vi "SubMatrixVg.vi"(0 "Target Voltage, V":dbl=1.0 min=-4.0 max=4.0 step=0.1 format="%.4f", 2 "Sweep rate, V/min":dbl=0.1 min=0.0 max=1.0 step=0.01 format="%.4f", 3 "Custom Folder":string, 4 "Time Stamp":timestamp, 5 "optional Bias (V)":dbl=1e-08) -> ()   [LabVIEW 2015]
uses:
  <vilib>/Utility/file.llb/Write To Spreadsheet File (DBL).vi
panel:
  out "Comments":string[](array[string])
  out "ArrayBoolian":bool[][](array[boolean])
  out "Numeric 4":i32
  in  "Commutator":bool
  in  "Commute SorceMeter":enum32{"Radio Selection 1", "Radio Selection 2"}(radio)
  out "Numeric 3":i32
  in  "Channel 2 (Vnano3b)":bool
  in  "Channel 1 (Vnano3)":bool
  out "Numeric":i32
  in  "Capacitance (C) and Loss (L)":bool
  in  "Magnetic Field (B)":bool=TRUE
  in  "Current (Ik3)":bool
  in  "Voltage (Vk3)":bool
  in  "Current (Ik2)":bool
  in  "Voltage (Vk2)":bool
  in  "Channel 2 (Vnano2b)":bool
  in  "Channel 1 (Vnano2)":bool
  in  "Thermometer 1 (T1)":bool=TRUE
  in  "Channel 2 (Vnano1b)":bool
  in  "Channel 1 (Vnano1)":bool
  in  "Current (Ik1)":bool=TRUE
  in  "Voltage (Vk1)":bool
  out "Numeric Current":dbl
  out "Main Keithly2614B address":string="12"
  out "Delib Time delay":i32
  in  "points at each Vg":i32=1
  out "XY Graph":cluster{dbl[], dbl[]}(graph)={[1.0, 0.8, 0.6000000000000001, 0.4000000000000001, 0.20000000000000007, 5.551115123125783e-17, -0.19999999999999996, -0.39999999999999997, -0.6, -0.8, -1.0], [0.03352775, 0.056811, 0.03911575, 0.04330675, -0.02468015, 0.011641600000000002, 0.10151450000000001, 0.12386675000000001, 0.08288825000000001, -0.00186266, -0.038650000000000004]}
  in  "Time btw \npoints, sec":dbl=1.0 format="%.2f"
  out "Array 2":dbl[][](array[numeric])
  out "array for data":dbl[](array[numeric])
  out "Array":string[](array[string])
  in  "Addr 1 lock-in oop":bool=TRUE
  in  "Ring":u16(ring) caption="Y-axis:" items=["Vg", "I", "R1", "R1oop", "Ik1", "T1", "B"]
  out "String":string
  out "Data file:":path
  in  "Set compliance limit, mkA":dbl=0.05 min=0.0 max=1.0 step=0.01 format="%.3f"
  in  "error in (no error)":errorcluster
  in  "Ring 3":u16(ring)=1 items=["1 kOhm", "10 kOhm", "100 kOhm", "1 Mohm", "10 mOhm"]
  in  "Ring 2":u16(ring)=4 items=["1 kOhm", "10 kOhm", "100 kOhm", "1 Mohm", "10 mOhm"]
  in  "Fixed Current mkA":dbl=0.5
  in  "Current is:":T1(radio)
  in  "Ressitance measurements?":bool=TRUE
  in  "Addr 5 lock-in oop":bool
  in  "Addr 4 lock-in oop":bool
  in  "Addr 3 lock-in oop":bool
  in  "Addr 2 lock-in oop":bool
  in  "Addr 5 lock-in":bool
  in  "Addr 4 lock-in":bool
  in  "Addr 3 lock-in":bool
  in  "Addr 2 lock-in":bool
  in  "Addr 1 lock-in":bool=TRUE
  # "Keithley 2400: address 12"
  # "0"
  # "SourceMeters"
  # "Nanovoltmeters"
  # "Temperature"
  # "Main"
  # "Magnetic Field"
  # "(not recommended, too slow)"
  # "Capacitance & Loss"
  # "(not recommended, too slow)"
  # "(not recommended, too slow)"
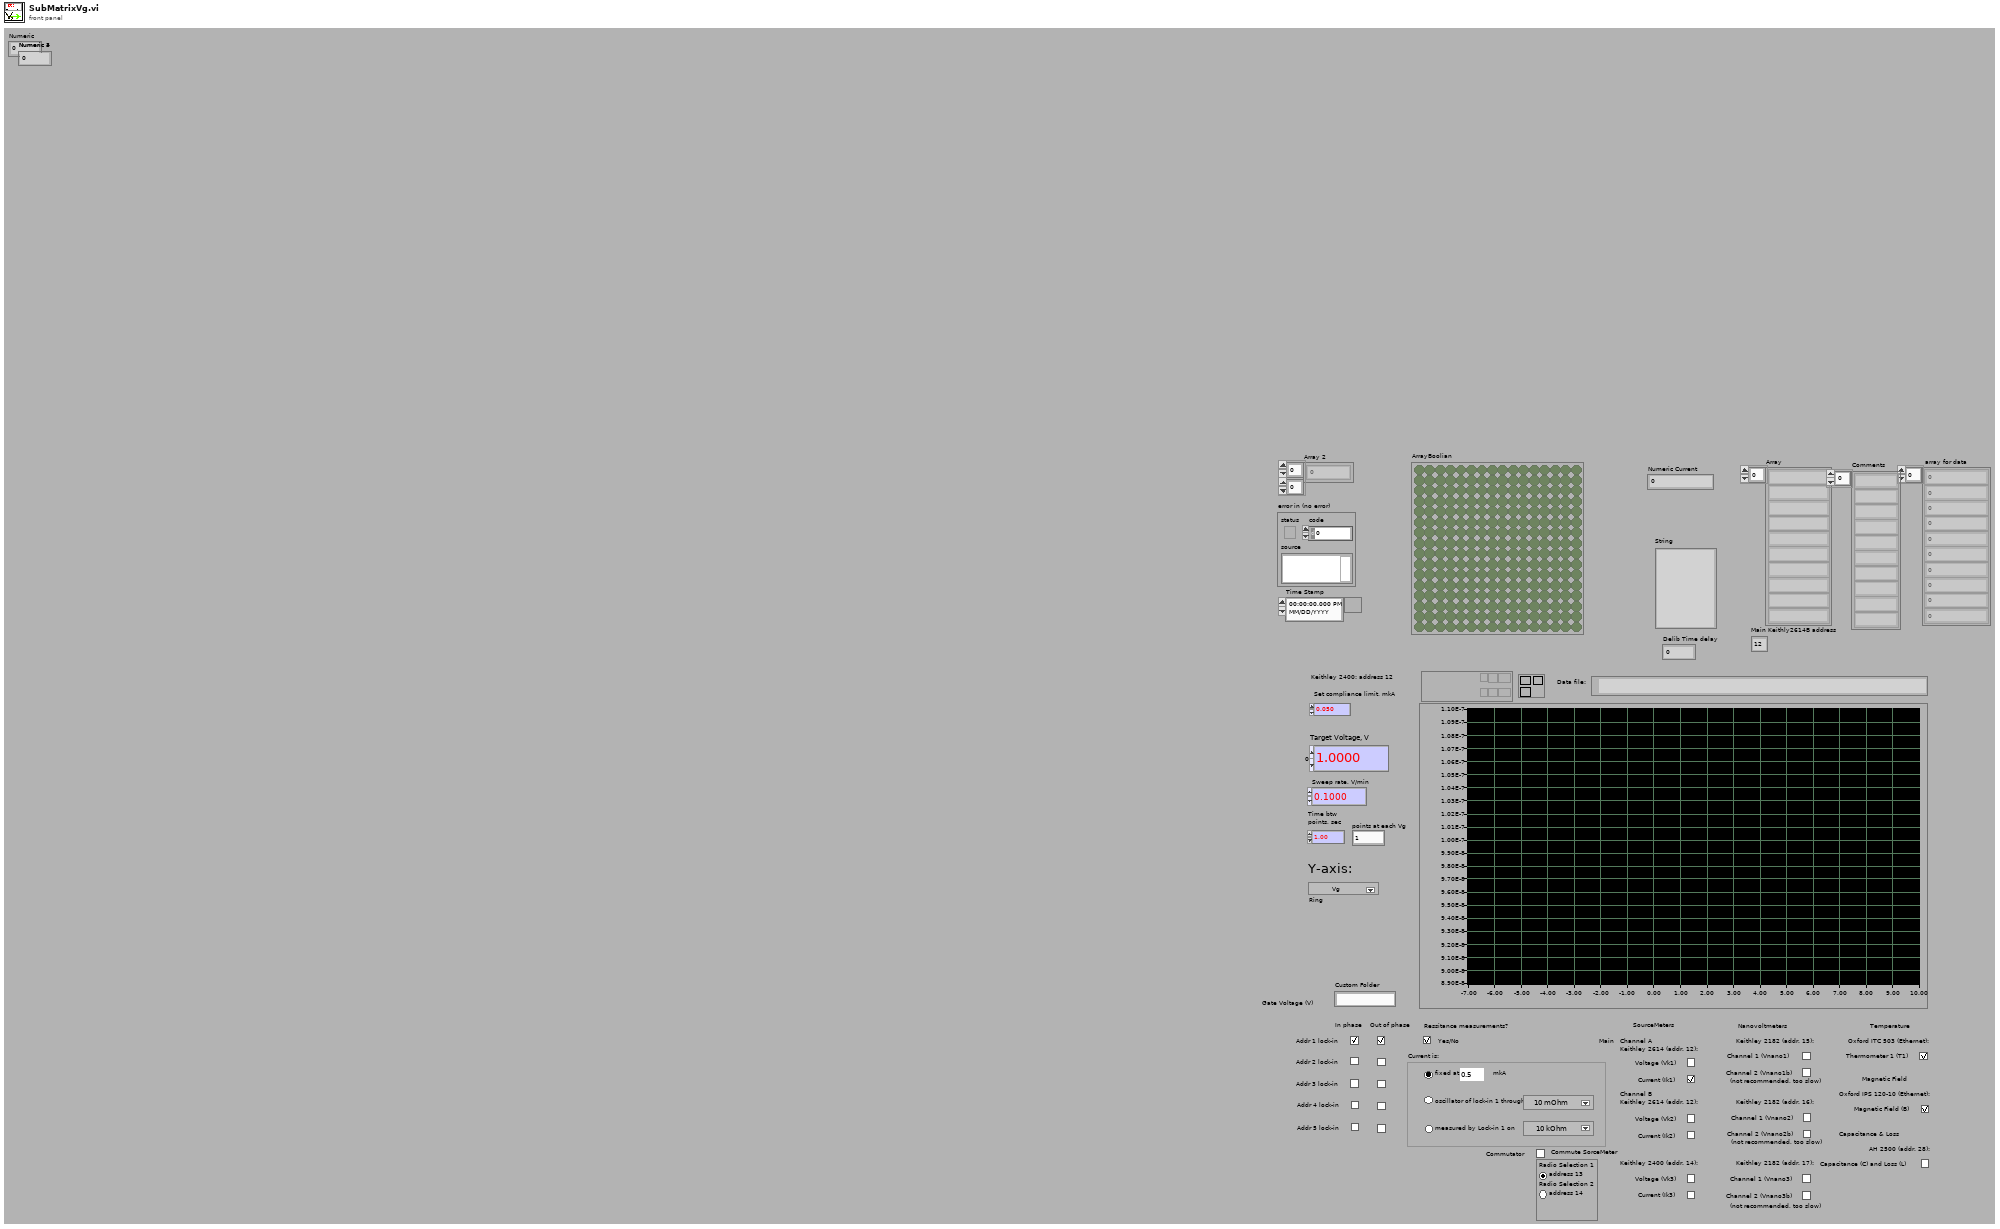
[diagram p1: front panel]
types:
  T1 = enum32{"Radio Selection 1", "Radio Selection 2", "Radio Selection 3"}
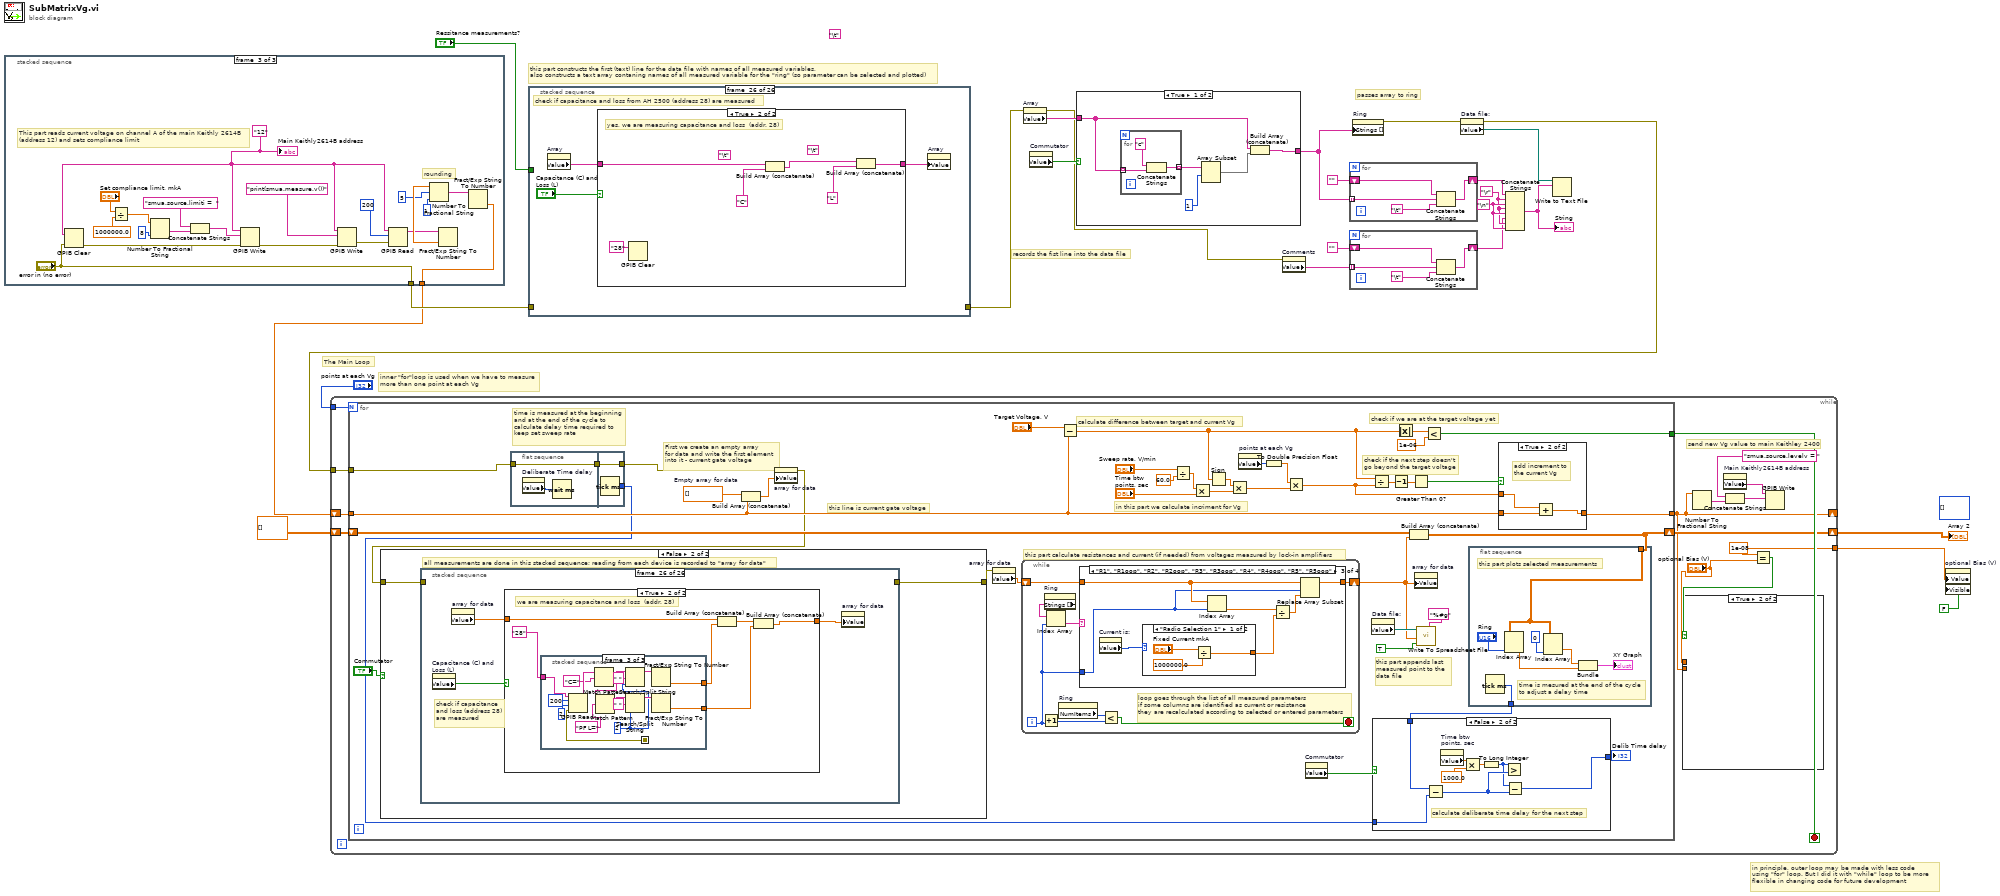
[diagram p0: block diagram]
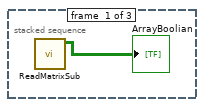
[diagram p3: hidden frame]
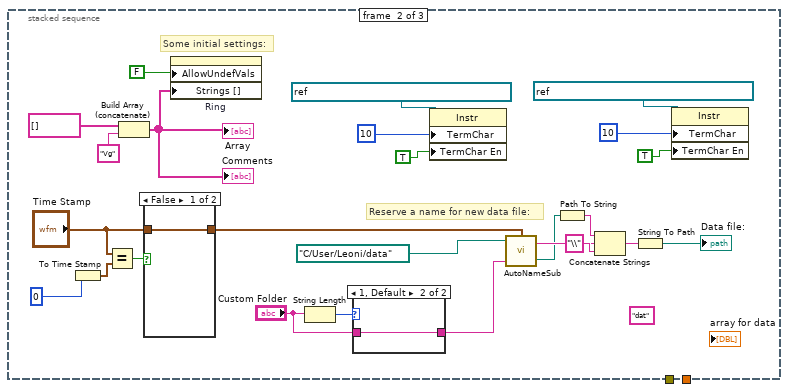
[diagram p4: hidden frame]
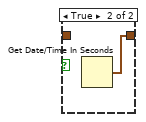
[diagram p5: hidden frame]
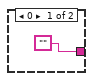
[diagram p6: hidden frame]
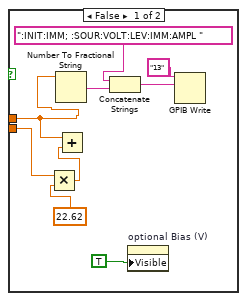
[diagram p7: hidden frame]
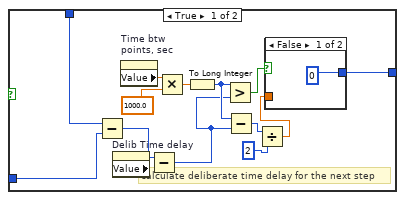
[diagram p8: hidden frame]
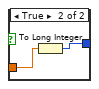
[diagram p9: hidden frame]
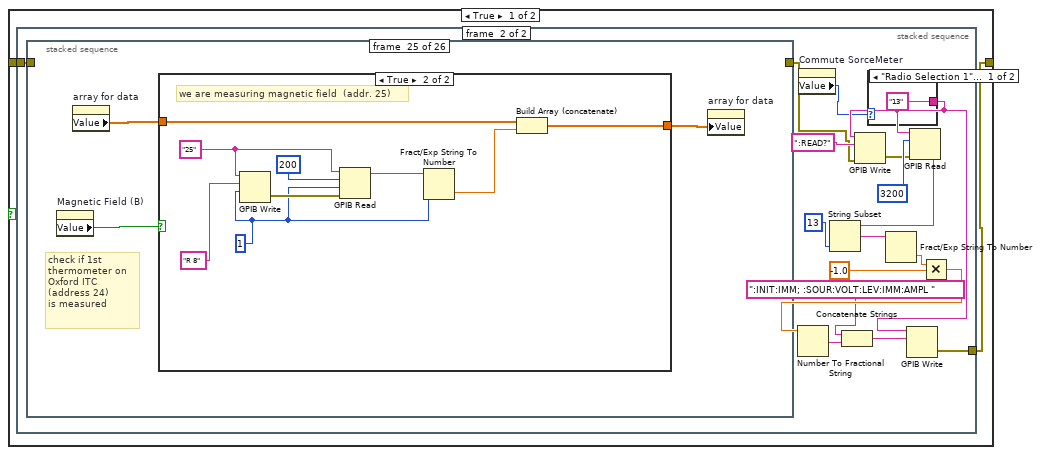
[diagram p10: hidden frame]
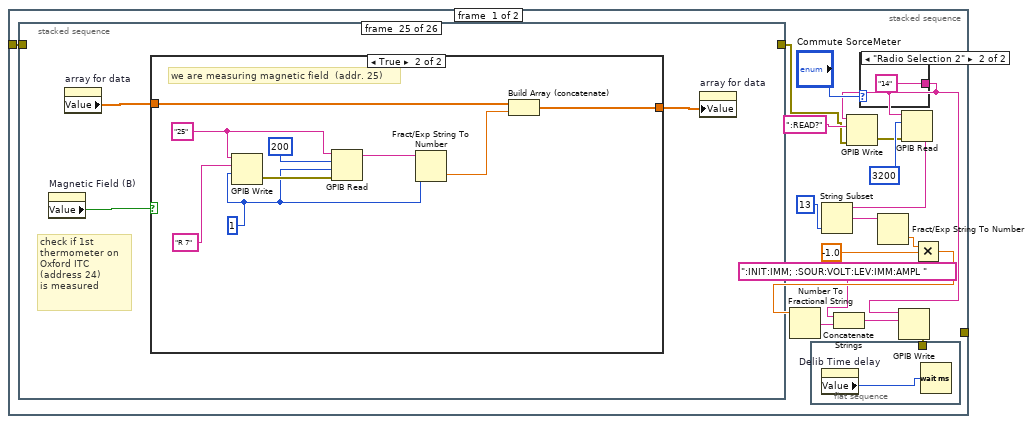
[diagram p11: hidden frame]
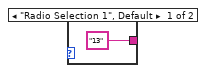
[diagram p12: hidden frame]
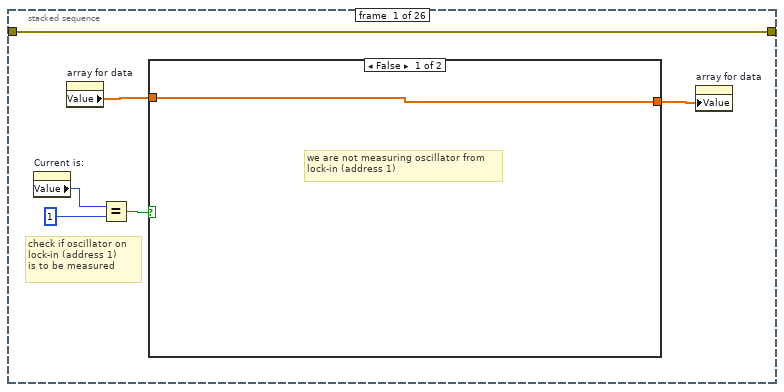
[diagram p13: hidden frame]
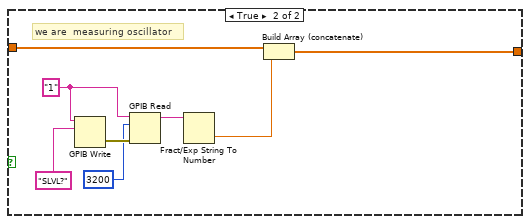
[diagram p14: hidden frame]
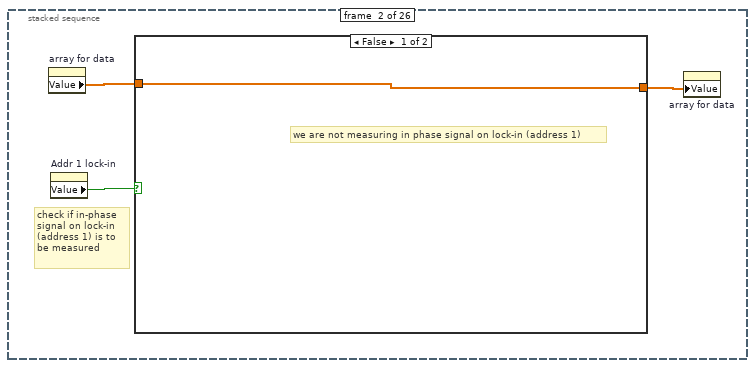
[diagram p15: hidden frame]
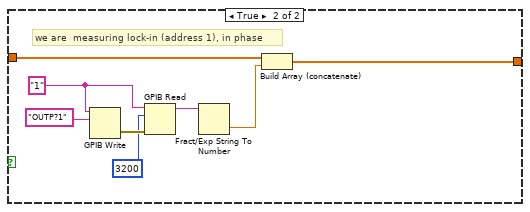
[diagram p16: hidden frame]
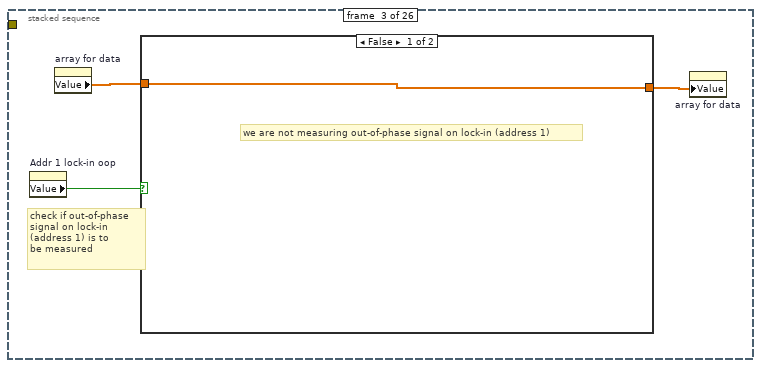
[diagram p17: hidden frame]
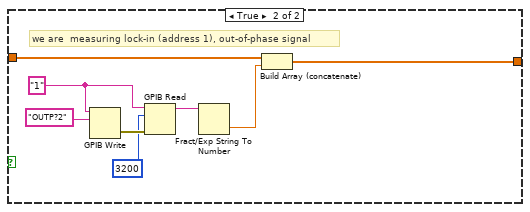
[diagram p18: hidden frame]
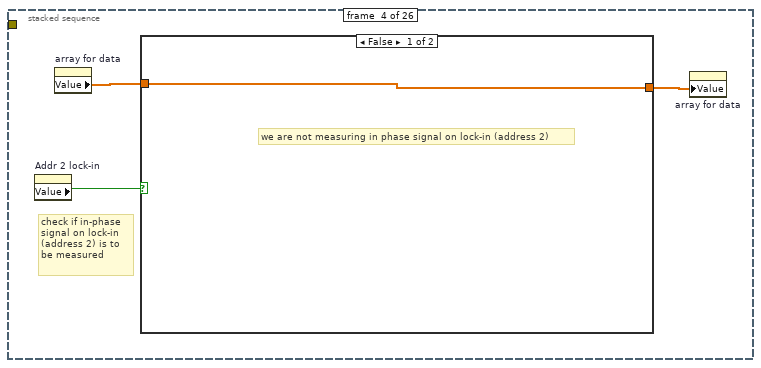
[diagram p19: hidden frame]
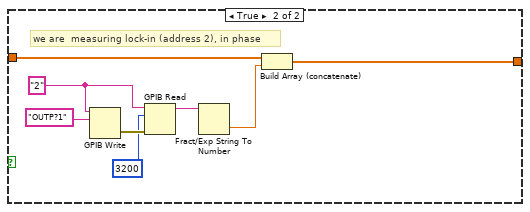
[diagram p20: hidden frame]
diagram:
  (unwired) "\t"
  w3 = "\r"
  w4 = "\n"
  (unwired) i32[][] []
  # "passes array to ring"
  # "in principle, outer loop may be made with less code\nusing \"for\" loop. But I did it with \"while\" loop to be more \nflexible in changing code for future development"
  # "inner \"for\"loop is used when we have to measure\nmore than one point at each Vg"
  # "The Main Loop"
  # "records the fist line into the data file"
  # "this part constructs the first (text) line for the data file with names of all measured variables,\nalso constructs a text array contaning names of all measured variable for the \"ring\" (so parameter can be selected and plotted)"
  n1 = stacked-sequence {
    tunnel: [_ _ "error in (no error)"] -> w24
    tunnel: [_ _ w55] -> w13
    frame #0 {
      n2 = call "ReadMatrixSub.vi"() -> ("Array"=→"ArrayBoolian":bool[][])  [unwired: 9 in, 2 out]
    }
    frame #1 {
      (unwired) "dat"
      # "Some initial settings:"
      # "Reserve a name for new data file:"
      n3 = To Time Stamp(1:0) -> (0:w29:timestamp)
      n4 = Equal?(x="Time Stamp", y=w29) -> (x = y?=w28:bool)
      n5 = Build Array (concatenate)(string[] [], "Vg") -> (w31:string[])
      "Array" <- w31
      "Comments" <- w31
      n6 = case shown="False" w28 {
        tunnel: "Time Stamp" -> [w51 _]
        tunnel: [w51 w52] -> w26
        frame False {
        }
        frame True {
          n7 = Get Date/Time In Seconds() -> (seconds since 1Jan1904=w52:timestamp)
        }
      }
      n8 = property on="Ring" class="Ring (strict)"("AllowUndefVals"=FALSE, "Strings []"=w31) -> ()  [unwired: 2 in, 2 out]
      n9 = String Length(string="Custom Folder") -> (length=w41:i32)
      n10 = case shown="1, Default" w41 {
        tunnel: "Custom Folder" -> [_ w54]
        tunnel: ["" w54] -> w39
        frame 0 {
        }
        frame 1, Default {
        }
      }
      n11 = property class="Instr"(reference=refnum<visa-resource-name> "TCPIP0::192.168.128.3::7020::SOCKET" ("VISA resource name"), "TermChar"=10, "TermChar En"=TRUE) -> ()  [unwired: 1 in, 2 out]
      n12 = call "AutoNameSub.vi"("Time Stamp"=w26, "Custom Folder"=w39, "User Data Folder"=path "C:/User/Leoni/data") -> ("created path"=w49:path, "String"=w50:string)  [unwired: 1 in]
      n13 = Path To String(path=w49) -> (string=w44:string)
      n14 = Concatenate Strings(w44, "\\", w50) -> (w46:string)
      n15 = String To Path(string=w46) -> (path=→"Data file:":path)
      n16 = property class="Instr"(reference=refnum<visa-resource-name> "TCPIP0::192.168.128.2::7020::SOCKET" ("VISA resource name"), "TermChar"=10, "TermChar En"=TRUE) -> ()  [unwired: 1 in, 2 out]
    }
    frame #2 {
      w62 = "12"
      # "rounding"
      # "This part reads current voltage on channel A of the main Keithly 2614B \n(address 12) and sets compliance limit"
      n17 = GPIB Clear(2:"error in (no error)", 3:w62) -> (0:w67:errorcluster)  [unwired: 1 out]
      n18 = Divide(x="Set compliance limit, mkA", y=1000000.0) -> (x/y=w73:dbl)
      n19 = Number To Fractional String(number=w73, precision (6)=i16 8) -> (F-format string=w69:string)  [unwired: 2 in]
      n20 = Concatenate Strings("smua.source.limiti =  " ("data"), w69) -> (w68:string)
      n21 = GPIB Write(0:w62, 1:w68, 3:w67) -> (6:w63:errorcluster)  [unwired: 2 in, 1 out]
      n22 = GPIB Write(0:w62, 1:"print(smua.measure.v())" ("data"), 3:w63) -> (6:w66:errorcluster)  [unwired: 2 in, 1 out]
      n23 = GPIB Read(0:w62, 1:200 ("byte count"), 3:w66) -> (5:w56:string)  [unwired: 2 in, 2 out]
      n24 = Fract/Exp String To Number(string=w56) -> (number=w60:dbl)  [unwired: 3 in, 1 out]
      n25 = Number To Fractional String(number=w60, width (-)=5, precision (6)=1) -> (F-format string=w57:string)  [unwired: 1 in]
      n26 = Fract/Exp String To Number(string=w57) -> (number=w55:dbl)  [unwired: 3 in, 1 out]
      "Main Keithly2614B address" <- w62
    }
  }
  n27 = stacked-sequence {
    tunnel: "Ressitance measurements?" -> [w82 w103 w130 w147 w167 w179 w191 w203 w215 w227 w239 _ _ _ _ _ _ _ _ _ _ _ _ _ _ _]
    tunnel: w24 -> [_ w102 _ _ _ _ _ _ _ _ _ _ _ _ _ _ _ _ _ _ _ _ _ _ _ _]
    tunnel: [_ w102 _ _ _ _ _ _ _ _ _ _ _ _ _ _ _ _ _ _ _ _ _ _ _ _] -> w21
    frame #0 {
      # "check if oscillator of  lock-in (address 1) is to be measured"
      n28 = property on="Array" class="Arr (strict)"() -> ("Value"=w78:string[])  [unwired: 2 in, 2 out]
      n29 = property on="Comments" class="Arr (strict)"() -> ("Value"=w75:string[])  [unwired: 2 in, 2 out]
      n30 = Equal?(x="Current is:", y=1) -> (x = y?=w80:bool)
      n31 = case shown="True" w80 {
        tunnel: w82 -> [_ _]
        tunnel: w78 -> [w84 w95]
        tunnel: [w84 w94] -> w77
        tunnel: [w83 w87] -> w76
        tunnel: w75 -> [w83 w86]
        frame False {
          # "we are not measuring oscillator from\nlock-in (address 1)"
        }
        frame True {
          # "This subVI takes the matrix column # (instrument\nconnection point) as an argument and finds the raw\n# (contact) to which the instrument is connected"
          # "we are  measuring oscillator"
          n32 = property on="ArrayBoolian" class="Arr (strict)"() -> ("Value"=w91:bool[][])  [unwired: 2 in, 2 out]
          n33 = GPIB Clear(3:"1") -> ()  [unwired: 1 in, 2 out]
          n34 = call "FindInstrConnect.vi"("Column #"=1, "ArrayBoolian"=w91) -> ("String"=w92:string)  [unwired: 1 in, 2 out]
          n35 = call "FindInstrConnect.vi"("Column #"=0, "ArrayBoolian"=w91) -> ("String"=w89:string)  [unwired: 1 in, 2 out]
          n36 = Concatenate Strings(w89, "-", w92) -> (w85:string)
          n37 = Build Array (concatenate)(w95, "I") -> (w94:string[])
          n38 = Build Array (concatenate)(w86, w85) -> (w87:string[])
        }
      }
      n39 = property on="Comments" class="Arr (strict)"("Value"=w76) -> ()  [unwired: 2 in, 2 out]
      n40 = property on="Array" class="Arr (strict)"("Value"=w77) -> ()  [unwired: 2 in, 2 out]
    }
    frame #1 {
      # "check if lock-in (address 1) is to be measured"
      n41 = property on="Array" class="Arr (strict)"() -> ("Value"=w101:string[])  [unwired: 2 in, 2 out]
      n42 = property on="Comments" class="Arr (strict)"() -> ("Value"=w99:string[])  [unwired: 2 in, 2 out]
      n43 = case shown="True" "Addr 1 lock-in" {
        tunnel: w103 -> [_ w119]
        tunnel: w101 -> [w106 w117]
        tunnel: [w106 w118] -> w100
        tunnel: w99 -> [w105 w108]
        tunnel: [w105 w109] -> w98
        frame False {
          # "we are not measuring in phase signal from\nlock-in (address 1)"
        }
        frame True {
          # "are we measuring resistance?"
          n44 = case shown="True" w119 {
            tunnel: ["V1" w121] -> w110
            frame False {
              # "no, we are not measuring resistanse;\nall lock-ins are measuring voltage"
            }
            frame True {
              # "are we measuring current as well?"
              n45 = property on="Current is:" class="RadioBtnsControl (strict)"() -> ("Value"=w123:T1)  [unwired: 2 in, 2 out]
              n46 = Equal?(x=w123, y=2) -> (x = y?=w124:bool)
              n47 = case shown="False" w124 {
                tunnel: ["R1" "I"] -> w121
                frame False {
                  # "no, we are not \nmeasuring current\nby lock-in \n(address 1); \nso this lock-in is \nmeasuring resistance"
                }
                frame True {
                  # "yes, we are measuring \ncurrent by lock-in \n(address 1) as \nvoltage drop on \nknown resistance"
                }
              }
            }
          }
          n48 = property on="ArrayBoolian" class="Arr (strict)"() -> ("Value"=w111:bool[][])  [unwired: 2 in, 2 out]
          n49 = call "FindInstrConnect.vi"("Column #"=3, "ArrayBoolian"=w111) -> ("String"=w114:string)  [unwired: 1 in, 2 out]
          n50 = call "FindInstrConnect.vi"("Column #"=2, "ArrayBoolian"=w111) -> ("String"=w112:string)  [unwired: 1 in, 2 out]
          n51 = Concatenate Strings(w112, "-", w114) -> (w107:string)
          n52 = Build Array (concatenate)(w117, w110) -> (w118:string[])
          n53 = Build Array (concatenate)(w108, w107) -> (w109:string[])
        }
      }
      n54 = property on="Array" class="Arr (strict)"("Value"=w100) -> ()  [unwired: 2 in, 2 out]
      n55 = property on="Comments" class="Arr (strict)"("Value"=w98) -> ()  [unwired: 2 in, 2 out]
    }
    frame #2 {
      # "check if out-of-phase signal on  lock-in (address 1) is to be measured"
      n56 = property on="Array" class="Arr (strict)"() -> ("Value"=w129:string[])  [unwired: 2 in, 2 out]
      n57 = case shown="True" "Addr 1 lock-in oop" {
        tunnel: w130 -> [_ w136]
        tunnel: w129 -> [w131 w133]
        tunnel: [w131 w134] -> w128
        frame False {
          # "we are not measuring iout-of-phase signal from\nlock-in (address 1)"
        }
        frame True {
          # "are we measuring resistance?"
          n58 = GPIB Clear(3:"1") -> ()  [unwired: 1 in, 2 out]
          n59 = case shown="False" w136 {
            tunnel: ["V1oop" w138] -> w132
            frame False {
              # "no, we are not measuring resistance;\nall lock-ins are measuring voltage"
            }
            frame True {
              # "are we measuring out-of-phase current as well?"
              n60 = property on="Current is:" class="RadioBtnsControl (strict)"() -> ("Value"=w140:T1)  [unwired: 2 in, 2 out]
              n61 = Equal?(x=w140, y=2) -> (x = y?=w141:bool)
              n62 = case shown="True" w141 {
                tunnel: ["R1oop" "Ioop"] -> w138
                frame False {
                  # "no, we are not \nmeasuring current\nby lock-in \n(address 1); so this \nlock-in is measuring\nout-of-phase resistance"
                }
                frame True {
                  # "yes, we are measuring \nout-of phase current \nby lock-in (address 1) \nas voltage drop on \nknown resistance"
                }
              }
            }
          }
          n63 = Build Array (concatenate)(w133, w132) -> (w134:string[])
        }
      }
      n64 = property on="Array" class="Arr (strict)"("Value"=w128) -> ()  [unwired: 2 in, 2 out]
    }
    frame #3 {
      # "check if in-phase signal on  lock-in (address 2) is to be measured"
      n65 = property on="Array" class="Arr (strict)"() -> ("Value"=w146:string[])  [unwired: 2 in, 2 out]
      n66 = case shown="False" "Addr 2 lock-in" {
        tunnel: w147 -> [_ w161]
        tunnel: w146 -> [w148 w158]
        tunnel: [w148 w159] -> w145
        frame False {
          # "we are not measuring in-phase signal from\nlock-in (address 2)"
        }
        frame True {
          (unwired) "\t"
          # "are we measuring resistance?"
          n67 = GPIB Clear(3:"2") -> ()  [unwired: 1 in, 2 out]
          n68 = case shown="False" w161 {
            tunnel: ["R2 (" "V2 ("] -> w150
            frame True {
              # "we are measuring \nresistance by lock-in \n(address 2)"
            }
            frame False, Default {
              # "no, we are not \nmeasuring resistance;\nall lock-ins are \nmeasuring voltage"
            }
          }
          n69 = property on="ArrayBoolian" class="Arr (strict)"() -> ("Value"=w149:bool[][])  [unwired: 2 in, 2 out]
          n70 = call "FindInstrConnect.vi"("Column #"=5, "ArrayBoolian"=w149) -> ("String"=w154:string)  [unwired: 1 in, 2 out]
          n71 = call "FindInstrConnect.vi"("Column #"=4, "ArrayBoolian"=w149) -> ("String"=w152:string)  [unwired: 1 in, 2 out]
          n72 = Concatenate Strings(w150, w152, "-", w154, ")") -> (w151:string)
          n73 = Build Array (concatenate)(w158, w151) -> (w159:string[])
        }
      }
      n74 = property on="Array" class="Arr (strict)"("Value"=w145) -> ()  [unwired: 2 in, 2 out]
    }
    frame #4 {
      # "check if out-of-phase signal on  lock-in (address 2) is to be measured"
      n75 = property on="Array" class="Arr (strict)"() -> ("Value"=w166:string[])  [unwired: 2 in, 2 out]
      n76 = case shown="True" "Addr 2 lock-in oop" {
        tunnel: w167 -> [_ w173]
        tunnel: w166 -> [w168 w170]
        tunnel: [w168 w171] -> w165
        frame False {
          # "we are not measuring out-of-phase signal from\nlock-in (address 2)"
        }
        frame True {
          (unwired) "\t"
          # "are we measuring resistance?"
          n77 = GPIB Clear(3:"2") -> ()  [unwired: 1 in, 2 out]
          n78 = case shown="True" w173 {
            tunnel: ["R2oop" "V2oop"] -> w169
            frame True {
              # "we are measuring out-of-phase resistance by lock-in (address 2)\n(address 2)"
            }
            frame False, Default {
              # "no, we are not measuring resistance;\nall lock-ins are measuring voltage"
            }
          }
          n79 = Build Array (concatenate)(w170, w169) -> (w171:string[])
        }
      }
      n80 = property on="Array" class="Arr (strict)"("Value"=w165) -> ()  [unwired: 2 in, 2 out]
    }
    frame #5 {
      # "check if in-phase signal on  lock-in (address 3) is to be measured"
      n81 = property on="Array" class="Arr (strict)"() -> ("Value"=w178:string[])  [unwired: 2 in, 2 out]
      n82 = case shown="True" "Addr 3 lock-in" {
        tunnel: w179 -> [_ w185]
        tunnel: w178 -> [w180 w182]
        tunnel: [w180 w183] -> w177
        frame False {
          # "we are not measuring in-phase signal from\nlock-in (address 3)"
        }
        frame True {
          (unwired) "\t"
          # "are we measuring resistance?"
          n83 = GPIB Clear(3:"3") -> ()  [unwired: 1 in, 2 out]
          n84 = case shown="True" w185 {
            tunnel: ["R3" "V3"] -> w181
            frame True {
              # "we are measuring \nresistance by lock-in \n(address 3)"
            }
            frame False, Default {
              # "no, we are not measuring resistance;\nall lock-ins are measuring voltage"
            }
          }
          n85 = Build Array (concatenate)(w182, w181) -> (w183:string[])
        }
      }
      n86 = property on="Array" class="Arr (strict)"("Value"=w177) -> ()  [unwired: 2 in, 2 out]
    }
    frame #6 {
      # "check if out-of-phase signal on  lock-in (address 3) is to be measured"
      n87 = property on="Array" class="Arr (strict)"() -> ("Value"=w190:string[])  [unwired: 2 in, 2 out]
      n88 = case shown="False" "Addr 3 lock-in oop" {
        tunnel: w191 -> [_ w197]
        tunnel: w190 -> [w192 w194]
        tunnel: [w192 w195] -> w189
        frame False {
          # "we are not measuring out-of-phase signal from\nlock-in (address 3)"
        }
        frame True {
          (unwired) "\t"
          # "are we measuring resistance?"
          n89 = GPIB Clear(3:"3") -> ()  [unwired: 1 in, 2 out]
          n90 = case shown="True" w197 {
            tunnel: ["R3oop" "V3oop"] -> w193
            frame True {
              # "we are measuring out-of-phase resistance by lock-in (address 3)\n(address 2)"
            }
            frame False, Default {
              # "no, we are not measuring resistance;\nall lock-ins are measuring voltage"
            }
          }
          n91 = Build Array (concatenate)(w194, w193) -> (w195:string[])
        }
      }
      n92 = property on="Array" class="Arr (strict)"("Value"=w189) -> ()  [unwired: 2 in, 2 out]
    }
    frame #7 {
      # "check if in-phase signal on  lock-in (address 4) is to be measured"
      n93 = property on="Array" class="Arr (strict)"() -> ("Value"=w202:string[])  [unwired: 2 in, 2 out]
      n94 = case shown="False" "Addr 4 lock-in" {
        tunnel: w203 -> [_ w209]
        tunnel: w202 -> [w204 w206]
        tunnel: [w204 w207] -> w201
        frame False {
          # "we are not measuring in-phase signal from\nlock-in (address 4)"
        }
        frame True {
          (unwired) "\t"
          # "are we measuring resistance?"
          n95 = GPIB Clear(3:"4") -> ()  [unwired: 1 in, 2 out]
          n96 = case shown="True" w209 {
            tunnel: ["R4" "V4"] -> w205
            frame True {
              # "we are measuring \nresistance by lock-in \n(address 4)"
            }
            frame False, Default {
              # "no, we are not measuring resistance;\nall lock-ins are measuring voltage"
            }
          }
          n97 = Build Array (concatenate)(w206, w205) -> (w207:string[])
        }
      }
      n98 = property on="Array" class="Arr (strict)"("Value"=w201) -> ()  [unwired: 2 in, 2 out]
    }
    frame #8 {
      # "check if out-of-phase signal on  lock-in (address 4) is to be measured"
      n99 = property on="Array" class="Arr (strict)"() -> ("Value"=w214:string[])  [unwired: 2 in, 2 out]
      n100 = case shown="False" "Addr 4 lock-in oop" {
        tunnel: w215 -> [_ w221]
        tunnel: w214 -> [w216 w218]
        tunnel: [w216 w219] -> w213
        frame False {
          # "we are not measuring out-of-phase signal from\nlock-in (address 4)"
        }
        frame True {
          (unwired) "\t"
          # "are we measuring resistance?"
          n101 = GPIB Clear(3:"4") -> ()  [unwired: 1 in, 2 out]
          n102 = case shown="True" w221 {
            tunnel: ["R4oop" "V4oop"] -> w217
            frame True {
              # "we are measuring out-of-phase resistance by lock-in (address 4)\n(address 2)"
            }
            frame False, Default {
              # "no, we are not measuring resistance;\nall lock-ins are measuring voltage"
            }
          }
          n103 = Build Array (concatenate)(w218, w217) -> (w219:string[])
        }
      }
      n104 = property on="Array" class="Arr (strict)"("Value"=w213) -> ()  [unwired: 2 in, 2 out]
    }
    frame #9 {
      # "check if in-phase signal on  lock-in (address 5) is to be measured"
      n105 = property on="Array" class="Arr (strict)"() -> ("Value"=w226:string[])  [unwired: 2 in, 2 out]
      n106 = case shown="False" "Addr 5 lock-in" {
        tunnel: w227 -> [_ w233]
        tunnel: w226 -> [w228 w230]
        tunnel: [w228 w231] -> w225
        frame False {
          # "we are not measuring in-phase signal from\nlock-in (address 5)"
        }
        frame True {
          (unwired) "\t"
          # "are we measuring resistance?"
          n107 = GPIB Clear(3:"5") -> ()  [unwired: 1 in, 2 out]
          n108 = case shown="True" w233 {
            tunnel: ["R5" "V5"] -> w229
            frame True {
              # "we are measuring \nresistance by lock-in \n(address 5)"
            }
            frame False, Default {
              # "no, we are not measuring resistance;\nall lock-ins are measuring voltage"
            }
          }
          n109 = Build Array (concatenate)(w230, w229) -> (w231:string[])
        }
      }
      n110 = property on="Array" class="Arr (strict)"("Value"=w225) -> ()  [unwired: 2 in, 2 out]
    }
    frame #10 {
      # "check if out-of-phase signal on  lock-in (address 5) is to be measured"
      n111 = property on="Array" class="Arr (strict)"() -> ("Value"=w238:string[])  [unwired: 2 in, 2 out]
      n112 = case shown="False" "Addr 5 lock-in oop" {
        tunnel: w239 -> [_ w245]
        tunnel: w238 -> [w240 w242]
        tunnel: [w240 w243] -> w237
        frame False {
          # "we are not measuring out-of-phase signal from\nlock-in (address 5)"
        }
        frame True {
          (unwired) "\t"
          # "are we measuring resistance?"
          n113 = GPIB Clear(3:"5") -> ()  [unwired: 1 in, 2 out]
          n114 = case shown="True" w245 {
            tunnel: ["R5oop" "V5oop"] -> w241
            frame True {
              # "we are measuring out-of-phase resistance by lock-in (address 5)\n(address 2)"
            }
            frame False, Default {
              # "no, we are not measuring resistance;\nall lock-ins are measuring voltage"
            }
          }
          n115 = Build Array (concatenate)(w242, w241) -> (w243:string[])
        }
      }
      n116 = property on="Array" class="Arr (strict)"("Value"=w237) -> ()  [unwired: 2 in, 2 out]
    }
    frame #11 {
      # "check if voltage on main Keithley 2400 (addr. 12) is measured"
      n117 = property on="Array" class="Arr (strict)"() -> ("Value"=w250:string[])  [unwired: 2 in, 2 out]
      n118 = case shown="False" "Voltage (Vk1)" {
        tunnel: w250 -> [w251 w253]
        tunnel: [w251 w254] -> w249
        frame False {
          # "no , we aren't measuring voltage \non main Keithley 2400 (addr. 12)"
        }
        frame True {
          (unwired) "\t"
          # "yes , we are measuring voltage \non main Keithley 2400 (addr. 12)"
          n119 = GPIB Clear(3:"12") -> ()  [unwired: 1 in, 2 out]
          n120 = Build Array (concatenate)(w253, "Vk1") -> (w254:string[])
        }
      }
      n121 = property on="Array" class="Arr (strict)"("Value"=w249) -> ()  [unwired: 2 in, 2 out]
    }
    frame #12 {
      # "check if current on main Keithley 2400 (addr. 12) is measured"
      n122 = property on="Array" class="Arr (strict)"() -> ("Value"=w258:string[])  [unwired: 2 in, 2 out]
      n123 = case shown="True" "Current (Ik1)" {
        tunnel: w258 -> [w259 w261]
        tunnel: [w259 w262] -> w257
        frame False {
          # "no , we aren't measuring current\non main Keithley 2400 (addr. 12)"
        }
        frame True {
          (unwired) "\t"
          # "yes , we are measuring current \non main Keithley 2400 (addr. 12)"
          n124 = GPIB Clear(3:"12") -> ()  [unwired: 1 in, 2 out]
          n125 = Build Array (concatenate)(w261, "Ik1") -> (w262:string[])
        }
      }
      n126 = property on="Array" class="Arr (strict)"("Value"=w257) -> ()  [unwired: 2 in, 2 out]
    }
    frame #13 {
      # "check if voltage on additional Keithley 2400 (addr. 13) is measured"
      n127 = property on="Array" class="Arr (strict)"() -> ("Value"=w266:string[])  [unwired: 2 in, 2 out]
      n128 = case shown="False" "Voltage (Vk2)" {
        tunnel: w266 -> [w267 w269]
        tunnel: [w267 w270] -> w265
        frame False {
          # "no , we aren't measuring voltage \non Keithley 2400 (addr. 13)"
        }
        frame True {
          (unwired) "\t"
          # "yes , we are measuring voltage \non Keithley 2400 (addr. 13)"
          n129 = GPIB Clear(3:"13") -> ()  [unwired: 1 in, 2 out]
          n130 = Build Array (concatenate)(w269, "Vk2") -> (w270:string[])
        }
      }
      n131 = property on="Array" class="Arr (strict)"("Value"=w265) -> ()  [unwired: 2 in, 2 out]
    }
    frame #14 {
      # "check if current on additional Keithley 2400 (addr. 13) is measured"
      n132 = property on="Array" class="Arr (strict)"() -> ("Value"=w274:string[])  [unwired: 2 in, 2 out]
      n133 = case shown="False" "Current (Ik2)" {
        tunnel: w274 -> [w275 w277]
        tunnel: [w275 w278] -> w273
        frame False {
          # "no , we aren't measuring current\non Keithley 2400 (addr. 13)"
        }
        frame True {
          (unwired) "\t"
          # "yes , we are measuring current \non Keithley 2400 (addr. 13)"
          n134 = GPIB Clear(3:"13") -> ()  [unwired: 1 in, 2 out]
          n135 = Build Array (concatenate)(w277, "Ik2") -> (w278:string[])
        }
      }
      n136 = property on="Array" class="Arr (strict)"("Value"=w273) -> ()  [unwired: 2 in, 2 out]
    }
    frame #15 {
      # "check if voltage on additional Keithley 2400 (addr. 14) is measured"
      n137 = property on="Array" class="Arr (strict)"() -> ("Value"=w282:string[])  [unwired: 2 in, 2 out]
      n138 = case shown="False" "Voltage (Vk3)" {
        tunnel: w282 -> [w283 w285]
        tunnel: [w283 w286] -> w281
        frame False {
          # "no , we aren't measuring voltage \non Keithley 2400 (addr. 14)"
        }
        frame True {
          (unwired) "\t"
          # "yes , we are measuring voltage \non Keithley 2400 (addr. 14)"
          n139 = GPIB Clear(3:"14") -> ()  [unwired: 1 in, 2 out]
          n140 = Build Array (concatenate)(w285, "Vk3") -> (w286:string[])
        }
      }
      n141 = property on="Array" class="Arr (strict)"("Value"=w281) -> ()  [unwired: 2 in, 2 out]
    }
    frame #16 {
      # "check if current on additional Keithley 2400 (addr. 14) is measured"
      n142 = property on="Array" class="Arr (strict)"() -> ("Value"=w290:string[])  [unwired: 2 in, 2 out]
      n143 = case shown="False" "Current (Ik3)" {
        tunnel: w290 -> [w291 w293]
        tunnel: [w291 w294] -> w289
        frame False {
          # "no , we aren't measuring current\non Keithley 2400 (addr. 14)"
        }
        frame True {
          (unwired) "\t"
          # "yes , we are measuring current \non Keithley 2400 (addr. 14)"
          n144 = GPIB Clear(3:"14") -> ()  [unwired: 1 in, 2 out]
          n145 = Build Array (concatenate)(w293, "Ik3") -> (w294:string[])
        }
      }
      n146 = property on="Array" class="Arr (strict)"("Value"=w289) -> ()  [unwired: 2 in, 2 out]
    }
    frame #17 {
      # "check if 1st channel of nanovoltmeter Keithley 2182 (addr. 15) is measured"
      n147 = property on="Array" class="Arr (strict)"() -> ("Value"=w298:string[])  [unwired: 2 in, 2 out]
      n148 = case shown="True" "Channel 1 (Vnano1)" {
        tunnel: w298 -> [w299 w302]
        tunnel: [w299 w303] -> w297
        frame False {
          # "no , we are not measuring 1st channel\non Keithley 2182 (addr. 15)"
        }
        frame True {
          (unwired) "\t"
          # "yes , we are measuring 1st channel\non Keithley 2182 (addr. 15)"
          n149 = GPIB Clear(3:"15") -> ()  [unwired: 1 in, 2 out]
          n150 = Build Array (concatenate)(w302, "Vnano1") -> (w303:string[])
        }
      }
      n151 = property on="Array" class="Arr (strict)"("Value"=w297) -> ()  [unwired: 2 in, 2 out]
    }
    frame #18 {
      # "check if 2nd channel of nanovoltmeter Keithley 2182 (addr. 15) is measured"
      n152 = property on="Array" class="Arr (strict)"() -> ("Value"=w306:string[])  [unwired: 2 in, 2 out]
      n153 = case shown="True" "Channel 2 (Vnano1b)" {
        tunnel: w306 -> [w307 w309]
        tunnel: [w307 w310] -> w305
        frame False {
          # "no , we are not measuring 2nd channel\non Keithley 2182 (addr. 15)"
        }
        frame True {
          (unwired) "\t"
          # "yes , we are measuring 2nd channel\non Keithley 2182 (addr. 15)"
          n154 = GPIB Clear(3:"15") -> ()  [unwired: 1 in, 2 out]
          n155 = Build Array (concatenate)(w309, "Vnano1b") -> (w310:string[])
        }
      }
      n156 = property on="Array" class="Arr (strict)"("Value"=w305) -> ()  [unwired: 2 in, 2 out]
    }
    frame #19 {
      # "check if 1st channel of nanovoltmeter Keithley 2182 (addr. 16) is measured"
      n157 = property on="Array" class="Arr (strict)"() -> ("Value"=w314:string[])  [unwired: 2 in, 2 out]
      n158 = case shown="False" "Channel 1 (Vnano2)" {
        tunnel: w314 -> [w315 w318]
        tunnel: [w315 w319] -> w313
        frame False {
          # "no , we are not measuring 1st channel\non Keithley 2182 (addr. 16)"
        }
        frame True {
          (unwired) "\t"
          # "yes , we are measuring 1st channel\non Keithley 2182 (addr. 16)"
          n159 = GPIB Clear(3:"16") -> ()  [unwired: 1 in, 2 out]
          n160 = Build Array (concatenate)(w318, "Vnano2") -> (w319:string[])
        }
      }
      n161 = property on="Array" class="Arr (strict)"("Value"=w313) -> ()  [unwired: 2 in, 2 out]
    }
    frame #20 {
      # "check if 2nd channel of nanovoltmeter Keithley 2182 (addr. 16) is measured"
      n162 = property on="Array" class="Arr (strict)"() -> ("Value"=w322:string[])  [unwired: 2 in, 2 out]
      n163 = case shown="False" "Channel 2 (Vnano2b)" {
        tunnel: w322 -> [w323 w325]
        tunnel: [w323 w326] -> w321
        frame False {
          # "no , we are not measuring 2nd channel\non Keithley 2182 (addr. 16)"
        }
        frame True {
          (unwired) "\t"
          # "yes , we are measuring 2nd channel\non Keithley 2182 (addr. 16)"
          n164 = GPIB Clear(3:"16") -> ()  [unwired: 1 in, 2 out]
          n165 = Build Array (concatenate)(w325, "Vnano2b") -> (w326:string[])
        }
      }
      n166 = property on="Array" class="Arr (strict)"("Value"=w321) -> ()  [unwired: 2 in, 2 out]
    }
    frame #21 {
      # "check if 1st channel of nanovoltmeter Keithley 2182 (addr. 17) is measured"
      n167 = property on="Array" class="Arr (strict)"() -> ("Value"=w330:string[])  [unwired: 2 in, 2 out]
      n168 = case shown="False" "Channel 1 (Vnano3)" {
        tunnel: w330 -> [w331 w333]
        tunnel: [w331 w334] -> w329
        frame False {
          # "no , we are not measuring 1st channel\non Keithley 2182 (addr. 17)"
        }
        frame True {
          (unwired) "\t"
          # "yes , we are measuring 1st channel\non Keithley 2182 (addr. 17)"
          n169 = GPIB Clear(3:"17") -> ()  [unwired: 1 in, 2 out]
          n170 = Build Array (concatenate)(w333, "Vnano3") -> (w334:string[])
        }
      }
      n171 = property on="Array" class="Arr (strict)"("Value"=w329) -> ()  [unwired: 2 in, 2 out]
    }
    frame #22 {
      # "check if 2nd channel of nanovoltmeter Keithley 2182 (addr. 16) is measured"
      n172 = property on="Array" class="Arr (strict)"() -> ("Value"=w338:string[])  [unwired: 2 in, 2 out]
      n173 = case shown="False" "Channel 2 (Vnano3b)" {
        tunnel: w338 -> [w339 w341]
        tunnel: [w339 w342] -> w337
        frame False {
          # "no , we are not measuring 2nd channel\non Keithley 2182 (addr. 17)"
        }
        frame True {
          (unwired) "\t"
          # "yes , we are measuring 2nd channel\non Keithley 2182 (addr. 17)"
          n174 = GPIB Clear(3:"17") -> ()  [unwired: 1 in, 2 out]
          n175 = Build Array (concatenate)(w341, "Vnano3b") -> (w342:string[])
        }
      }
      n176 = property on="Array" class="Arr (strict)"("Value"=w337) -> ()  [unwired: 2 in, 2 out]
    }
    frame #23 {
      # "check if 1st thermometer on Oxford ITC (address 24) is measured"
      n177 = property on="Array" class="Arr (strict)"() -> ("Value"=w346:string[])  [unwired: 2 in, 2 out]
      n178 = case shown="True" "Thermometer 1 (T1)" {
        tunnel: w346 -> [w347 w349]
        tunnel: [w347 w350] -> w345
        frame False {
          # "no, we are not measuring temperature\non thermometer 1 (addr. 24)"
        }
        frame True {
          (unwired) "\t"
          # "yes, we are measuring temperature,\nthermometer 1 (addr. 24)"
          n179 = GPIB Clear(3:"24") -> ()  [unwired: 1 in, 2 out]
          n180 = Build Array (concatenate)(w349, "T1") -> (w350:string[])
        }
      }
      n181 = property on="Array" class="Arr (strict)"("Value"=w345) -> ()  [unwired: 2 in, 2 out]
    }
    frame #24 {
      # "check if magnetic field from Oxford IPS 120 (address 25) is measured"
      n182 = property on="Array" class="Arr (strict)"() -> ("Value"=w354:string[])  [unwired: 2 in, 2 out]
      n183 = case shown="True" "Magnetic Field (B)" {
        tunnel: w354 -> [w355 w357]
        tunnel: [w355 w358] -> w353
        frame False {
          # "no, we are not measuring magnetic field  (addr. 25)"
        }
        frame True {
          (unwired) "\t"
          # "yes, we are measuring magnetic field  (addr. 25)"
          n184 = GPIB Clear(3:"25") -> ()  [unwired: 1 in, 2 out]
          n185 = Build Array (concatenate)(w357, "B") -> (w358:string[])
        }
      }
      n186 = property on="Array" class="Arr (strict)"("Value"=w353) -> ()  [unwired: 2 in, 2 out]
    }
    frame #25 {
      # "check if capacitance and loss from AH 2500 (address 28) are measured"
      n187 = property on="Array" class="Arr (strict)"() -> ("Value"=w362:string[])  [unwired: 2 in, 2 out]
      n188 = case shown="True" "Capacitance (C) and Loss (L)" {
        tunnel: w362 -> [w363 w365]
        tunnel: [w363 w368] -> w361
        frame False {
          # "no, we are not measuring capacitance  (addr. 28)"
        }
        frame True {
          (unwired) "\t"
          (unwired) "\t"
          # "yes, we are measuring capacitance and loss  (addr. 28)"
          n189 = GPIB Clear(3:"28") -> ()  [unwired: 1 in, 2 out]
          n190 = Build Array (concatenate)(w365, "C") -> (w364:string[])
          n191 = Build Array (concatenate)(w364, "L") -> (w368:string[])
        }
      }
      n192 = property on="Array" class="Arr (strict)"("Value"=w361) -> ()  [unwired: 2 in, 2 out]
    }
  }
  n193 = property on="Array" class="Arr (strict)"(error in=w21) -> (error out=w1:errorcluster, "Value"=w12:string[])  [unwired: 1 in, 1 out]
  n194 = property on="Commutator" class="Bool (strict)"() -> ("Value"=w11:bool)  [unwired: 2 in, 2 out]
  n195 = case shown="True" w11 {
    tunnel: w12 -> [w371 w378]
    tunnel: [w370 w378] -> w9
    frame True {
      n196 = for {
        tunnel: [w377] -> w374 mode=indexing
        tunnel: w371 -> [w375] mode=indexing
        n197 = Concatenate Strings("c", w375) -> (w377:string)
      }
      n198 = Array Subset(array=w374, index=1) -> (w372:string[])  [unwired: 1 in]
      n199 = Build Array (concatenate)(w371, w372) -> (w370:string[])
    }
    frame False {
    }
  }
  n200 = property on="Comments" class="Arr (strict)"(error in=w1) -> ("Value"=w5:string[])  [unwired: 1 in, 2 out]
  n201 = for {
    tunnel: w9 -> [w381] mode=indexing
    shift-right: [w379] -> w7
    shift-left: "" -> [w380]
    n202 = Concatenate Strings(w380, w381, "\t") -> (w379:string)
  }
  n203 = for {
    tunnel: w5 -> [w385] mode=indexing
    shift-right: [w383] -> w2
    shift-left: "" -> [w384]
    n204 = Concatenate Strings(w384, w385, "\t") -> (w383:string)
  }
  n205 = property on="Ring" class="Ring (strict)"("Strings []"=w9) -> (error out=w10:errorcluster)  [unwired: 2 in, 1 out]
  n206 = property on="Data file:" class="Path"(error in=w10) -> (error out=w18:errorcluster, "Value"=w20:path)  [unwired: 1 in, 1 out]
  n207 = while {
    tunnel: w18 -> [w400]
    shift-right: [w397] -> w17
    shift-left: dbl[][] [] -> [w399]
    shift-right: [w389] -> _
    shift-left: w13 -> [w396]
    tunnel: "points at each Vg" -> [w391]
    tunnel: [w387] -> w15
    stop <- w398 stop-if-true
    w387 = 1e-08
    # "send new Vg value to main Keithley 2400"
    n208 = for {
      N: w391 -> [_]
      tunnel: w400 -> [w416]
      tunnel: [w434] -> w398
      shift-right: [w421] -> w397
      shift-left: w399 -> [w447]
      tunnel: w396 -> [w432]
      tunnel: [w439] -> w389
      w433 = dbl[] []  # Empty array for data
      # "this part appends last\nmeasured point to the \ndata file"
      # "this line is current gate voltage"
      # "First we create an empty array \nfor data and write the first element \ninto it - current gate voltage"
      # "time is measured at the beginning\nand at the end of the cycle to\ncalculate delay time required to\nkeep set sweep rate"
      # "this part calculate resistances and current (if needed) from voltages measured by lock-in amplifiers"
      # "check if the next step doesn't\ngo beyond the target voltage"
      # "calculate difference between target and current Vg"
      # "check if we are at the target voltage yet"
      # "in this part we calculate incriment for Vg"
      n209 = flat-sequence {
        tunnel: w416 -> [w1621]
        tunnel: [w1621] -> w414
        tunnel: [w1623] -> w415
        tunnel: w414 -> [w1623]
        tunnel: [w1622] -> w413
        frame #0 {
          n210 = property on="Deliberate Time delay" class="DigNum (strict)"() -> ("Value"=w1620:i32)  [unwired: 2 in, 2 out]
          n211 = Wait (ms)(milliseconds to wait=w1620) -> ()  [unwired: 1 out]
        }
        frame #1 {
          n212 = Tick Count (ms)() -> (millisecond timer value=w1622:u32)
        }
      }
      n213 = Build Array (concatenate)(w433, w432) -> (w431:dbl[])
      n214 = property on="array for data" class="Arr (strict)"(error in=w415, "Value"=w431) -> (error out=w430:errorcluster)  [unwired: 1 in, 1 out]
      n215 = case shown="False" "Commutator" {
        tunnel: [w474 w1254] -> w448
        tunnel: w430 -> [w475 w1253]
        frame True {
          n216 = stacked-sequence {
            tunnel: w475 -> [w492 w881]
            tunnel: [_ w866] -> w474
            frame #0 {
              n217 = stacked-sequence {
                tunnel: w492 -> [w496 _ _ _ _ _ _ _ _ _ _ _ _ _ _ _ _ _ _ _ _ _ _ _ _ _]
                tunnel: [w496 _ _ _ _ _ _ _ _ _ _ _ _ _ _ _ _ _ _ _ _ _ _ _ _ _] -> w476
                frame #0 {
                  # "check if oscillator on \nlock-in (address 1)\nis to be measured"
                  n218 = property on="Current is:" class="RadioBtnsControl (strict)"() -> ("Value"=w499:T1)  [unwired: 2 in, 2 out]
                  n219 = property on="array for data" class="Arr (strict)"() -> ("Value"=w498:dbl[])  [unwired: 2 in, 2 out]
                  n220 = Equal?(x=w499, y=1) -> (x = y?=w500:bool)
                  n221 = case shown="False" w500 {
                    tunnel: w498 -> [w502 w510]
                    tunnel: [w502 w509] -> w497
                    frame False {
                      # "we are not measuring oscillator from\nlock-in (address 1)"
                    }
                    frame True {
                      w506 = "1"
                      # "we are  measuring oscillator"
                      n222 = GPIB Write(0:w506, 1:"SLVL?") -> (6:w507:errorcluster)  [unwired: 3 in, 1 out]
                      n223 = GPIB Read(0:w506, 1:3200, 3:w507) -> (5:w504:string)  [unwired: 2 in, 2 out]
                      n224 = Fract/Exp String To Number(string=w504) -> (number=w503:dbl)  [unwired: 3 in, 1 out]
                      n225 = Build Array (concatenate)(w510, w503) -> (w509:dbl[])
                    }
                  }
                  n226 = property on="array for data" class="Arr (strict)"("Value"=w497) -> ()  [unwired: 2 in, 2 out]
                }
                frame #1 {
                  # "check if in-phase\nsignal on lock-in \n(address 1) is to\nbe measured"
                  n227 = property on="array for data" class="Arr (strict)"() -> ("Value"=w513:dbl[])  [unwired: 2 in, 2 out]
                  n228 = property on="Addr 1 lock-in" class="Bool (strict)"() -> ("Value"=w511:bool)  [unwired: 2 in, 2 out]
                  n229 = case shown="False" w511 {
                    tunnel: w513 -> [w514 w522]
                    tunnel: [w514 w521] -> w512
                    frame False {
                      # "we are not measuring in phase signal on lock-in (address 1)"
                    }
                    frame True {
                      w519 = "1"
                      # "we are  measuring lock-in (address 1), in phase"
                      n230 = GPIB Write(0:w519, 1:"OUTP?1") -> (6:w520:errorcluster)  [unwired: 3 in, 1 out]
                      n231 = GPIB Read(0:w519, 1:3200, 3:w520) -> (5:w517:string)  [unwired: 2 in, 2 out]
                      n232 = Fract/Exp String To Number(string=w517) -> (number=w516:dbl)  [unwired: 3 in, 1 out]
                      n233 = Build Array (concatenate)(w522, w516) -> (w521:dbl[])
                    }
                  }
                  n234 = property on="array for data" class="Arr (strict)"("Value"=w512) -> ()  [unwired: 2 in, 2 out]
                }
                frame #2 {
                  # "check if out-of-phase\nsignal on lock-in \n(address 1) is to\nbe measured"
                  n235 = property on="Addr 1 lock-in oop" class="Bool (strict)"() -> ("Value"=w523:bool)  [unwired: 2 in, 2 out]
                  n236 = property on="array for data" class="Arr (strict)"() -> ("Value"=w525:dbl[])  [unwired: 2 in, 2 out]
                  n237 = case shown="False" w523 {
                    tunnel: w525 -> [w526 w534]
                    tunnel: [w526 w533] -> w524
                    frame False {
                      # "we are not measuring out-of-phase signal on lock-in (address 1)"
                    }
                    frame True {
                      w531 = "1"
                      # "we are  measuring lock-in (address 1), out-of-phase signal"
                      n238 = GPIB Write(0:w531, 1:"OUTP?2") -> (6:w532:errorcluster)  [unwired: 3 in, 1 out]
                      n239 = GPIB Read(0:w531, 1:3200, 3:w532) -> (5:w529:string)  [unwired: 2 in, 2 out]
                      n240 = Fract/Exp String To Number(string=w529) -> (number=w528:dbl)  [unwired: 3 in, 1 out]
                      n241 = Build Array (concatenate)(w534, w528) -> (w533:dbl[])
                    }
                  }
                  n242 = property on="array for data" class="Arr (strict)"("Value"=w524) -> ()  [unwired: 2 in, 2 out]
                }
                frame #3 {
                  # "check if in-phase\nsignal on lock-in \n(address 2) is to\nbe measured"
                  n243 = property on="Addr 2 lock-in" class="Bool (strict)"() -> ("Value"=w535:bool)  [unwired: 2 in, 2 out]
                  n244 = property on="array for data" class="Arr (strict)"() -> ("Value"=w537:dbl[])  [unwired: 2 in, 2 out]
                  n245 = case shown="False" w535 {
                    tunnel: w537 -> [w538 w546]
                    tunnel: [w538 w545] -> w536
                    frame False {
                      # "we are not measuring in phase signal on lock-in (address 2)"
                    }
                    frame True {
                      w543 = "2"
                      # "we are  measuring lock-in (address 2), in phase"
                      n246 = GPIB Write(0:w543, 1:"OUTP?1") -> (6:w544:errorcluster)  [unwired: 3 in, 1 out]
                      n247 = GPIB Read(0:w543, 1:3200, 3:w544) -> (5:w541:string)  [unwired: 2 in, 2 out]
                      n248 = Fract/Exp String To Number(string=w541) -> (number=w540:dbl)  [unwired: 3 in, 1 out]
                      n249 = Build Array (concatenate)(w546, w540) -> (w545:dbl[])
                    }
                  }
                  n250 = property on="array for data" class="Arr (strict)"("Value"=w536) -> ()  [unwired: 2 in, 2 out]
                }
                frame #4 {
                  # "check if out-of-phase\nsignal on lock-in \n(address 2) is to\nbe measured"
                  n251 = property on="Addr 2 lock-in oop" class="Bool (strict)"() -> ("Value"=w547:bool)  [unwired: 2 in, 2 out]
                  n252 = property on="array for data" class="Arr (strict)"() -> ("Value"=w549:dbl[])  [unwired: 2 in, 2 out]
                  n253 = case shown="False" w547 {
                    tunnel: w549 -> [w550 w558]
                    tunnel: [w550 w557] -> w548
                    tunnel: w547 -> [_ _]
                    frame False {
                      # "we are not measuring out-of-phase signal on lock-in (address 2)"
                    }
                    frame True {
                      w555 = "2"
                      # "we are  measuring lock-in (address 2), out-of-phase"
                      n254 = GPIB Write(0:w555, 1:"OUTP?2") -> (6:w556:errorcluster)  [unwired: 3 in, 1 out]
                      n255 = GPIB Read(0:w555, 1:3200, 3:w556) -> (5:w553:string)  [unwired: 2 in, 2 out]
                      n256 = Fract/Exp String To Number(string=w553) -> (number=w552:dbl)  [unwired: 3 in, 1 out]
                      n257 = Build Array (concatenate)(w558, w552) -> (w557:dbl[])
                    }
                  }
                  n258 = property on="array for data" class="Arr (strict)"("Value"=w548) -> ()  [unwired: 2 in, 2 out]
                }
                frame #5 {
                  # "check if in-phase\nsignal on lock-in \n(address 3) is to\nbe measured"
                  n259 = property on="Addr 3 lock-in" class="Bool (strict)"() -> ("Value"=w559:bool)  [unwired: 2 in, 2 out]
                  n260 = property on="array for data" class="Arr (strict)"() -> ("Value"=w561:dbl[])  [unwired: 2 in, 2 out]
                  n261 = case shown="False" w559 {
                    tunnel: w561 -> [w562 w570]
                    tunnel: [w562 w569] -> w560
                    frame False {
                      # "we are not measuring in phase signal on lock-in (address 3)"
                    }
                    frame True {
                      w567 = "3"
                      # "we are  measuring lock-in (address 3), in phase"
                      n262 = GPIB Write(0:w567, 1:"OUTP?1") -> (6:w568:errorcluster)  [unwired: 3 in, 1 out]
                      n263 = GPIB Read(0:w567, 1:3200, 3:w568) -> (5:w565:string)  [unwired: 2 in, 2 out]
                      n264 = Fract/Exp String To Number(string=w565) -> (number=w564:dbl)  [unwired: 3 in, 1 out]
                      n265 = Build Array (concatenate)(w570, w564) -> (w569:dbl[])
                    }
                  }
                  n266 = property on="array for data" class="Arr (strict)"("Value"=w560) -> ()  [unwired: 2 in, 2 out]
                }
                frame #6 {
                  # "check if out-of-phase\nsignal on lock-in \n(address 3) is to\nbe measured"
                  n267 = property on="Addr 3 lock-in oop" class="Bool (strict)"() -> ("Value"=w571:bool)  [unwired: 2 in, 2 out]
                  n268 = property on="array for data" class="Arr (strict)"() -> ("Value"=w573:dbl[])  [unwired: 2 in, 2 out]
                  n269 = case shown="False" w571 {
                    tunnel: w573 -> [w574 w582]
                    tunnel: [w574 w581] -> w572
                    frame False {
                      # "we are not measuring out-of-phase signal on lock-in (address 3)"
                    }
                    frame True {
                      w579 = "3"
                      # "we are  measuring lock-in (address 3), out-of-phase"
                      n270 = GPIB Write(0:w579, 1:"OUTP?2") -> (6:w580:errorcluster)  [unwired: 3 in, 1 out]
                      n271 = GPIB Read(0:w579, 1:3200, 3:w580) -> (5:w577:string)  [unwired: 2 in, 2 out]
                      n272 = Fract/Exp String To Number(string=w577) -> (number=w576:dbl)  [unwired: 3 in, 1 out]
                      n273 = Build Array (concatenate)(w582, w576) -> (w581:dbl[])
                    }
                  }
                  n274 = property on="array for data" class="Arr (strict)"("Value"=w572) -> ()  [unwired: 2 in, 2 out]
                }
                frame #7 {
                  # "check if in-phase\nsignal on lock-in \n(address 4) is to\nbe measured"
                  n275 = property on="Addr 4 lock-in" class="Bool (strict)"() -> ("Value"=w583:bool)  [unwired: 2 in, 2 out]
                  n276 = property on="array for data" class="Arr (strict)"() -> ("Value"=w585:dbl[])  [unwired: 2 in, 2 out]
                  n277 = case shown="False" w583 {
                    tunnel: w585 -> [w586 w594]
                    tunnel: [w586 w593] -> w584
                    frame False {
                      # "we are not measuring in phase signal on lock-in (address 4)"
                    }
                    frame True {
                      w591 = "4"
                      # "we are  measuring lock-in (address 4), in phase"
                      n278 = GPIB Write(0:w591, 1:"OUTP?1") -> (6:w592:errorcluster)  [unwired: 3 in, 1 out]
                      n279 = GPIB Read(0:w591, 1:3200, 3:w592) -> (5:w589:string)  [unwired: 2 in, 2 out]
                      n280 = Fract/Exp String To Number(string=w589) -> (number=w588:dbl)  [unwired: 3 in, 1 out]
                      n281 = Build Array (concatenate)(w594, w588) -> (w593:dbl[])
                    }
                  }
                  n282 = property on="array for data" class="Arr (strict)"("Value"=w584) -> ()  [unwired: 2 in, 2 out]
                }
                frame #8 {
                  # "check if out-of-phase\nsignal on lock-in \n(address 4) is to\nbe measured"
                  n283 = property on="Addr 4 lock-in oop" class="Bool (strict)"() -> ("Value"=w595:bool)  [unwired: 2 in, 2 out]
                  n284 = property on="array for data" class="Arr (strict)"() -> ("Value"=w597:dbl[])  [unwired: 2 in, 2 out]
                  n285 = case shown="False" w595 {
                    tunnel: w597 -> [w598 w606]
                    tunnel: [w598 w605] -> w596
                    frame False {
                      # "we are not measuring out-of-phase signal on lock-in (address 4)"
                    }
                    frame True {
                      w603 = "4"
                      # "we are  measuring lock-in (address 4), out-of-phase"
                      n286 = GPIB Write(0:w603, 1:"OUTP?2") -> (6:w604:errorcluster)  [unwired: 3 in, 1 out]
                      n287 = GPIB Read(0:w603, 1:3200, 3:w604) -> (5:w601:string)  [unwired: 2 in, 2 out]
                      n288 = Fract/Exp String To Number(string=w601) -> (number=w600:dbl)  [unwired: 3 in, 1 out]
                      n289 = Build Array (concatenate)(w606, w600) -> (w605:dbl[])
                    }
                  }
                  n290 = property on="array for data" class="Arr (strict)"("Value"=w596) -> ()  [unwired: 2 in, 2 out]
                }
                frame #9 {
                  # "check if in-phase\nsignal on lock-in \n(address 5) is to\nbe measured"
                  n291 = property on="Addr 5 lock-in" class="Bool (strict)"() -> ("Value"=w607:bool)  [unwired: 2 in, 2 out]
                  n292 = property on="array for data" class="Arr (strict)"() -> ("Value"=w609:dbl[])  [unwired: 2 in, 2 out]
                  n293 = case shown="False" w607 {
                    tunnel: w609 -> [w610 w618]
                    tunnel: [w610 w617] -> w608
                    frame False {
                      # "we are not measuring in phase signal on lock-in (address 5)"
                    }
                    frame True {
                      w615 = "5"
                      # "we are  measuring lock-in (address 5), in phase"
                      n294 = GPIB Write(0:w615, 1:"OUTP?1") -> (6:w616:errorcluster)  [unwired: 3 in, 1 out]
                      n295 = GPIB Read(0:w615, 1:3200, 3:w616) -> (5:w613:string)  [unwired: 2 in, 2 out]
                      n296 = Fract/Exp String To Number(string=w613) -> (number=w612:dbl)  [unwired: 3 in, 1 out]
                      n297 = Build Array (concatenate)(w618, w612) -> (w617:dbl[])
                    }
                  }
                  n298 = property on="array for data" class="Arr (strict)"("Value"=w608) -> ()  [unwired: 2 in, 2 out]
                }
                frame #10 {
                  # "check if out-of-phase\nsignal on lock-in \n(address 5) is to\nbe measured"
                  n299 = property on="Addr 5 lock-in oop" class="Bool (strict)"() -> ("Value"=w619:bool)  [unwired: 2 in, 2 out]
                  n300 = property on="array for data" class="Arr (strict)"() -> ("Value"=w621:dbl[])  [unwired: 2 in, 2 out]
                  n301 = case shown="False" w619 {
                    tunnel: w621 -> [w622 w630]
                    tunnel: [w622 w629] -> w620
                    frame False {
                      # "we are not measuring out-of-phase signal on lock-in (address 5)"
                    }
                    frame True {
                      w627 = "5"
                      # "we are  measuring lock-in (address 5), out-of-phase"
                      n302 = GPIB Write(0:w627, 1:"OUTP?2") -> (6:w628:errorcluster)  [unwired: 3 in, 1 out]
                      n303 = GPIB Read(0:w627, 1:3200, 3:w628) -> (5:w625:string)  [unwired: 2 in, 2 out]
                      n304 = Fract/Exp String To Number(string=w625) -> (number=w624:dbl)  [unwired: 3 in, 1 out]
                      n305 = Build Array (concatenate)(w630, w624) -> (w629:dbl[])
                    }
                  }
                  n306 = property on="array for data" class="Arr (strict)"("Value"=w620) -> ()  [unwired: 2 in, 2 out]
                }
                frame #11 {
                  # "check if voltage on \nmain Keithley 2400 \n(addr. 12) is to\nbe measured"
                  n307 = property on="Voltage (Vk1)" class="Bool (strict)"() -> ("Value"=w631:bool)  [unwired: 2 in, 2 out]
                  n308 = property on="array for data" class="Arr (strict)"() -> ("Value"=w633:dbl[])  [unwired: 2 in, 2 out]
                  n309 = case shown="False" w631 {
                    tunnel: w633 -> [w634 w644]
                    tunnel: [w634 w643] -> w632
                    frame False {
                      # "we aren't measuring voltage \non main Keithley 2400 (addr. 12)"
                    }
                    frame True {
                      w641 = "12"
                      # "we are measuring voltage \non main Keithley 2400 (addr. 12)"
                      n310 = GPIB Write(0:w641, 1:":READ?") -> (6:w642:errorcluster)  [unwired: 3 in, 1 out]
                      n311 = GPIB Read(0:w641, 1:3200, 3:w642) -> (5:w637:string)  [unwired: 2 in, 2 out]
                      n312 = String Subset(string=w637, length (rest)=13) -> (substring=w636:string)  [unwired: 1 in]
                      n313 = Fract/Exp String To Number(string=w636) -> (number=w639:dbl)  [unwired: 3 in, 1 out]
                      n314 = Build Array (concatenate)(w644, w639) -> (w643:dbl[])
                    }
                  }
                  n315 = property on="array for data" class="Arr (strict)"("Value"=w632) -> ()  [unwired: 2 in, 2 out]
                }
                frame #12 {
                  # "check if  current on \nmain Keithley 2400 \n(addr. 12) is to\nbe measured"
                  n316 = property on="Current (Ik1)" class="Bool (strict)"() -> ("Value"=w645:bool)  [unwired: 2 in, 2 out]
                  n317 = property on="array for data" class="Arr (strict)"() -> ("Value"=w647:dbl[])  [unwired: 2 in, 2 out]
                  n318 = case shown="True" w645 {
                    tunnel: w647 -> [w648 w659]
                    tunnel: [w648 w658] -> w646
                    frame False {
                      # "we aren't measuring current \non main Keithley 2400 (addr. 12)"
                    }
                    frame True {
                      w656 = "12"
                      # "we are measuring current\non main Keithley 2400 (addr. 12)"
                      n319 = GPIB Write(0:w656, 1:":READ?") -> (6:w657:errorcluster)  [unwired: 3 in, 1 out]
                      n320 = GPIB Read(0:w656, 1:3200, 3:w657) -> (5:w652:string)  [unwired: 2 in, 2 out]
                      n321 = String Subset(string=w652, offset (0)=14, length (rest)=13) -> (substring=w651:string)
                      n322 = Fract/Exp String To Number(string=w651) -> (number=w654:dbl)  [unwired: 3 in, 1 out]
                      n323 = Build Array (concatenate)(w659, w654) -> (w658:dbl[])
                    }
                  }
                  n324 = property on="array for data" class="Arr (strict)"("Value"=w646) -> ()  [unwired: 2 in, 2 out]
                }
                frame #13 {
                  # "check if voltage on \nadd. Keithley 2400 \n(addr. 13) is to\nbe measured"
                  n325 = property on="Voltage (Vk2)" class="Bool (strict)"() -> ("Value"=w660:bool)  [unwired: 2 in, 2 out]
                  n326 = property on="array for data" class="Arr (strict)"() -> ("Value"=w662:dbl[])  [unwired: 2 in, 2 out]
                  n327 = case shown="True" w660 {
                    tunnel: w662 -> [w663 w673]
                    tunnel: [w663 w672] -> w661
                    frame False {
                      # "we aren't measuring voltage \non additional Keithley 2400 (addr. 13)"
                    }
                    frame True {
                      w670 = "13"
                      # "we are measuring voltage \non additional Keithley 2400 (addr. 13)"
                      n328 = GPIB Write(0:w670, 1:":READ?") -> (6:w671:errorcluster)  [unwired: 3 in, 1 out]
                      n329 = GPIB Read(0:w670, 1:3200, 3:w671) -> (5:w666:string)  [unwired: 2 in, 2 out]
                      n330 = String Subset(string=w666, length (rest)=13) -> (substring=w665:string)  [unwired: 1 in]
                      n331 = Fract/Exp String To Number(string=w665) -> (number=w668:dbl)  [unwired: 3 in, 1 out]
                      n332 = Build Array (concatenate)(w673, w668) -> (w672:dbl[])
                    }
                  }
                  n333 = property on="array for data" class="Arr (strict)"("Value"=w661) -> ()  [unwired: 2 in, 2 out]
                }
                frame #14 {
                  # "check if  current on \nadd. Keithley 2400 \n(addr. 13) is to\nbe measured"
                  n334 = property on="Current (Ik2)" class="Bool (strict)"() -> ("Value"=w674:bool)  [unwired: 2 in, 2 out]
                  n335 = property on="array for data" class="Arr (strict)"() -> ("Value"=w676:dbl[])  [unwired: 2 in, 2 out]
                  n336 = case shown="True" w674 {
                    tunnel: w676 -> [w677 w688]
                    tunnel: [w677 w687] -> w675
                    frame False {
                      # "we aren't measuring current \non additional Keithley 2400 (addr. 13)"
                    }
                    frame True {
                      w685 = "13"
                      # "we are measuring current\non additional Keithley 2400 (addr. 13)"
                      n337 = GPIB Write(0:w685, 1:":READ?") -> (6:w686:errorcluster)  [unwired: 3 in, 1 out]
                      n338 = GPIB Read(0:w685, 1:3200, 3:w686) -> (5:w681:string)  [unwired: 2 in, 2 out]
                      n339 = String Subset(string=w681, offset (0)=14, length (rest)=13) -> (substring=w680:string)
                      n340 = Fract/Exp String To Number(string=w680) -> (number=w683:dbl)  [unwired: 3 in, 1 out]
                      n341 = Build Array (concatenate)(w688, w683) -> (w687:dbl[])
                    }
                  }
                  n342 = property on="array for data" class="Arr (strict)"("Value"=w675) -> ()  [unwired: 2 in, 2 out]
                }
                frame #15 {
                  # "check if voltage on \nadd. Keithley 2400 \n(addr. 14) is to\nbe measured"
                  n343 = property on="Voltage (Vk3)" class="Bool (strict)"() -> ("Value"=w689:bool)  [unwired: 2 in, 2 out]
                  n344 = property on="array for data" class="Arr (strict)"() -> ("Value"=w691:dbl[])  [unwired: 2 in, 2 out]
                  n345 = case shown="True" w689 {
                    tunnel: w691 -> [w692 w702]
                    tunnel: [w692 w701] -> w690
                    frame False {
                      # "we aren't measuring voltage \non additional Keithley 2400 (addr. 14)"
                    }
                    frame True {
                      w699 = "14"
                      # "we are measuring voltage \non additional Keithley 2400 (addr. 14)"
                      n346 = GPIB Write(0:w699, 1:":READ?") -> (6:w700:errorcluster)  [unwired: 3 in, 1 out]
                      n347 = GPIB Read(0:w699, 1:3200, 3:w700) -> (5:w695:string)  [unwired: 2 in, 2 out]
                      n348 = String Subset(string=w695, length (rest)=13) -> (substring=w694:string)  [unwired: 1 in]
                      n349 = Fract/Exp String To Number(string=w694) -> (number=w697:dbl)  [unwired: 3 in, 1 out]
                      n350 = Build Array (concatenate)(w702, w697) -> (w701:dbl[])
                    }
                  }
                  n351 = property on="array for data" class="Arr (strict)"("Value"=w690) -> ()  [unwired: 2 in, 2 out]
                }
                frame #16 {
                  # "check if  current on \nadd. Keithley 2400 \n(addr. 14) is to\nbe measured"
                  n352 = property on="Current (Ik3)" class="Bool (strict)"() -> ("Value"=w703:bool)  [unwired: 2 in, 2 out]
                  n353 = property on="array for data" class="Arr (strict)"() -> ("Value"=w705:dbl[])  [unwired: 2 in, 2 out]
                  n354 = case shown="True" w703 {
                    tunnel: w705 -> [w706 w717]
                    tunnel: [w706 w716] -> w704
                    frame False {
                      # "we aren't measuring current \non additional Keithley 2400 (addr. 14)"
                    }
                    frame True {
                      w714 = "14"
                      # "we are measuring current\non additional Keithley 2400 (addr. 14)"
                      n355 = GPIB Write(0:w714, 1:":READ?") -> (6:w715:errorcluster)  [unwired: 3 in, 1 out]
                      n356 = GPIB Read(0:w714, 1:3200, 3:w715) -> (5:w710:string)  [unwired: 2 in, 2 out]
                      n357 = String Subset(string=w710, offset (0)=14, length (rest)=13) -> (substring=w709:string)
                      n358 = Fract/Exp String To Number(string=w709) -> (number=w712:dbl)  [unwired: 3 in, 1 out]
                      n359 = Build Array (concatenate)(w717, w712) -> (w716:dbl[])
                    }
                  }
                  n360 = property on="array for data" class="Arr (strict)"("Value"=w704) -> ()  [unwired: 2 in, 2 out]
                }
                frame #17 {
                  # "check if 1st channel\non Keithley 2182 \n(addr. 15) is to\nbe measured"
                  n361 = property on="Channel 1 (Vnano1)" class="Bool (strict)"() -> ("Value"=w718:bool)  [unwired: 2 in, 2 out]
                  n362 = property on="array for data" class="Arr (strict)"() -> ("Value"=w720:dbl[])  [unwired: 2 in, 2 out]
                  n363 = case shown="True" w718 {
                    tunnel: w720 -> [w721 w729]
                    tunnel: [w721 w728] -> w719
                    frame False {
                      # "we are not measuring 1st channel\non Keithley 2182 (addr. 15)"
                    }
                    frame True {
                      w726 = "15"
                      # "we are measuring 1st channel\non Keithley 2182 (addr. 15)"
                      n364 = GPIB Write(0:w726, 1:":SENSe:DATA:FRES?") -> (6:w727:errorcluster)  [unwired: 3 in, 1 out]
                      n365 = GPIB Read(0:w726, 1:200, 3:w727) -> (5:w722:string)  [unwired: 2 in, 2 out]
                      n366 = Fract/Exp String To Number(string=w722) -> (number=w724:dbl)  [unwired: 3 in, 1 out]
                      n367 = Build Array (concatenate)(w729, w724) -> (w728:dbl[])
                    }
                  }
                  n368 = property on="array for data" class="Arr (strict)"("Value"=w719) -> ()  [unwired: 2 in, 2 out]
                }
                frame #18 {
                  # "check if 2nd channel\non Keithley 2182 \n(addr. 15) is to\nbe measured"
                  n369 = property on="Channel 2 (Vnano1b)" class="Bool (strict)"() -> ("Value"=w730:bool)  [unwired: 2 in, 2 out]
                  n370 = property on="array for data" class="Arr (strict)"() -> ("Value"=w732:dbl[])  [unwired: 2 in, 2 out]
                  n371 = case shown="False" w730 {
                    tunnel: w732 -> [w733 w745]
                    tunnel: [w733 w744] -> w731
                    frame False {
                      # "we are not measuring 1st channel\non Keithley 2182 (addr. 15)"
                    }
                    frame True {
                      w736 = "15"
                      # "switching to channel 2 and then\nback to channel 1"
                      # "we are measuring 2nd channel\non Keithley 2182 (addr. 15)"
                      n372 = GPIB Write(0:w736, 1:":SENSe:CHAN 2") -> (6:w737:errorcluster)  [unwired: 3 in, 1 out]
                      n373 = GPIB Write(0:w736, 1:":SENSe:DATA:FRES?", 3:w737) -> (6:w743:errorcluster)  [unwired: 2 in, 1 out]
                      n374 = GPIB Read(0:w736, 1:200, 3:w743) -> (5:w739:string, 7:w735:errorcluster)  [unwired: 2 in, 1 out]
                      n375 = GPIB Write(0:w736, 1:":SENSe:CHAN 1", 3:w735) -> ()  [unwired: 2 in, 2 out]
                      n376 = Fract/Exp String To Number(string=w739) -> (number=w741:dbl)  [unwired: 3 in, 1 out]
                      n377 = Build Array (concatenate)(w745, w741) -> (w744:dbl[])
                    }
                  }
                  n378 = property on="array for data" class="Arr (strict)"("Value"=w731) -> ()  [unwired: 2 in, 2 out]
                }
                frame #19 {
                  # "check if 1st channel\non Keithley 2182 \n(addr. 16) is to\nbe measured"
                  n379 = property on="Channel 1 (Vnano2)" class="Bool (strict)"() -> ("Value"=w746:bool)  [unwired: 2 in, 2 out]
                  n380 = property on="array for data" class="Arr (strict)"() -> ("Value"=w748:dbl[])  [unwired: 2 in, 2 out]
                  n381 = case shown="True" w746 {
                    tunnel: w748 -> [w749 w757]
                    tunnel: [w749 w756] -> w747
                    frame False {
                      # "we are not measuring 1st channel\non Keithley 2182 (addr. 16)"
                    }
                    frame True {
                      w754 = "16"
                      # "we are measuring 1st channel\non Keithley 2182 (addr. 16)"
                      n382 = GPIB Write(0:w754, 1:":SENSe:DATA:FRES?") -> (6:w755:errorcluster)  [unwired: 3 in, 1 out]
                      n383 = GPIB Read(0:w754, 1:200, 3:w755) -> (5:w750:string)  [unwired: 2 in, 2 out]
                      n384 = Fract/Exp String To Number(string=w750) -> (number=w752:dbl)  [unwired: 3 in, 1 out]
                      n385 = Build Array (concatenate)(w757, w752) -> (w756:dbl[])
                    }
                  }
                  n386 = property on="array for data" class="Arr (strict)"("Value"=w747) -> ()  [unwired: 2 in, 2 out]
                }
                frame #20 {
                  # "check if 2nd channel\non Keithley 2182 \n(addr. 16) is to\nbe measured"
                  n387 = property on="Channel 2 (Vnano2b)" class="Bool (strict)"() -> ("Value"=w758:bool)  [unwired: 2 in, 2 out]
                  n388 = property on="array for data" class="Arr (strict)"() -> ("Value"=w760:dbl[])  [unwired: 2 in, 2 out]
                  n389 = case shown="False" w758 {
                    tunnel: w760 -> [w761 w773]
                    tunnel: [w761 w772] -> w759
                    frame False {
                      # "we are not measuring 1st channel\non Keithley 2182 (addr. 16)"
                    }
                    frame True {
                      w764 = "16"
                      # "switching to channel 2 and then\nback to channel 1"
                      # "we are measuring 2nd channel\non Keithley 2182 (addr. 16)"
                      n390 = GPIB Write(0:w764, 1:":SENSe:CHAN 2") -> (6:w765:errorcluster)  [unwired: 3 in, 1 out]
                      n391 = GPIB Write(0:w764, 1:":SENSe:DATA:FRES?", 3:w765) -> (6:w771:errorcluster)  [unwired: 2 in, 1 out]
                      n392 = GPIB Read(0:w764, 1:200, 3:w771) -> (5:w767:string, 7:w763:errorcluster)  [unwired: 2 in, 1 out]
                      n393 = GPIB Write(0:w764, 1:":SENSe:CHAN 1", 3:w763) -> ()  [unwired: 2 in, 2 out]
                      n394 = Fract/Exp String To Number(string=w767) -> (number=w769:dbl)  [unwired: 3 in, 1 out]
                      n395 = Build Array (concatenate)(w773, w769) -> (w772:dbl[])
                    }
                  }
                  n396 = property on="array for data" class="Arr (strict)"("Value"=w759) -> ()  [unwired: 2 in, 2 out]
                }
                frame #21 {
                  # "check if 1st channel\non Keithley 2182 \n(addr. 17) is to\nbe measured"
                  n397 = property on="Channel 1 (Vnano3)" class="Bool (strict)"() -> ("Value"=w774:bool)  [unwired: 2 in, 2 out]
                  n398 = property on="array for data" class="Arr (strict)"() -> ("Value"=w776:dbl[])  [unwired: 2 in, 2 out]
                  n399 = case shown="True" w774 {
                    tunnel: w776 -> [w777 w785]
                    tunnel: [w777 w784] -> w775
                    frame False {
                      # "we are not measuring 1st channel\non Keithley 2182 (addr. 17)"
                    }
                    frame True {
                      w782 = "17"
                      # "we are measuring 1st channel\non Keithley 2182 (addr. 17)"
                      n400 = GPIB Write(0:w782, 1:":SENSe:DATA:FRES?") -> (6:w783:errorcluster)  [unwired: 3 in, 1 out]
                      n401 = GPIB Read(0:w782, 1:200, 3:w783) -> (5:w778:string)  [unwired: 2 in, 2 out]
                      n402 = Fract/Exp String To Number(string=w778) -> (number=w780:dbl)  [unwired: 3 in, 1 out]
                      n403 = Build Array (concatenate)(w785, w780) -> (w784:dbl[])
                    }
                  }
                  n404 = property on="array for data" class="Arr (strict)"("Value"=w775) -> ()  [unwired: 2 in, 2 out]
                }
                frame #22 {
                  # "check if 2nd channel\non Keithley 2182 \n(addr. 17) is to\nbe measured"
                  n405 = property on="Channel 2 (Vnano3b)" class="Bool (strict)"() -> ("Value"=w786:bool)  [unwired: 2 in, 2 out]
                  n406 = property on="array for data" class="Arr (strict)"() -> ("Value"=w788:dbl[])  [unwired: 2 in, 2 out]
                  n407 = case shown="False" w786 {
                    tunnel: w788 -> [w789 w801]
                    tunnel: [w789 w800] -> w787
                    frame False {
                      # "we are not measuring 1st channel\non Keithley 2182 (addr. 17)"
                    }
                    frame True {
                      w792 = "17"
                      # "switching to channel 2 and then\nback to channel 1"
                      # "we are measuring 2nd channel\non Keithley 2182 (addr. 17)"
                      n408 = GPIB Write(0:w792, 1:":SENSe:CHAN 2") -> (6:w793:errorcluster)  [unwired: 3 in, 1 out]
                      n409 = GPIB Write(0:w792, 1:":SENSe:DATA:FRES?", 3:w793) -> (6:w799:errorcluster)  [unwired: 2 in, 1 out]
                      n410 = GPIB Read(0:w792, 1:200, 3:w799) -> (5:w795:string, 7:w791:errorcluster)  [unwired: 2 in, 1 out]
                      n411 = GPIB Write(0:w792, 1:":SENSe:CHAN 1", 3:w791) -> ()  [unwired: 2 in, 2 out]
                      n412 = Fract/Exp String To Number(string=w795) -> (number=w797:dbl)  [unwired: 3 in, 1 out]
                      n413 = Build Array (concatenate)(w801, w797) -> (w800:dbl[])
                    }
                  }
                  n414 = property on="array for data" class="Arr (strict)"("Value"=w787) -> ()  [unwired: 2 in, 2 out]
                }
                frame #23 {
                  # "check if 1st \nthermometer on \nOxford ITC \n(address 24) \nis measured"
                  n415 = property on="Thermometer 1 (T1)" class="Bool (strict)"() -> ("Value"=w802:bool)  [unwired: 2 in, 2 out]
                  n416 = property on="array for data" class="Arr (strict)"() -> ("Value"=w804:dbl[])  [unwired: 2 in, 2 out]
                  n417 = case shown="True" w802 {
                    tunnel: w804 -> [w805 w814]
                    tunnel: [w805 w813] -> w803
                    frame False {
                      # "we are not measuring temperature on\nthermometer 1 (addr. 24)"
                    }
                    frame True {
                      w806 = 1
                      w811 = "24"
                      # "we are measuring temperature,\nthermometer 1 (addr. 24)"
                      n418 = GPIB Write(0:w811, 1:"R 1", 2:w806) -> (6:w812:errorcluster)  [unwired: 2 in, 1 out]
                      n419 = GPIB Read(0:w811, 1:200, 2:w806, 3:w812) -> (5:w807:string)  [unwired: 1 in, 2 out]
                      n420 = Fract/Exp String To Number(string=w807, offset=w806) -> (number=w809:dbl)  [unwired: 2 in, 1 out]
                      n421 = Build Array (concatenate)(w814, w809) -> (w813:dbl[])
                    }
                  }
                  n422 = property on="array for data" class="Arr (strict)"("Value"=w803) -> ()  [unwired: 2 in, 2 out]
                }
                frame #24 {
                  # "check if 1st \nthermometer on \nOxford ITC \n(address 24) \nis measured"
                  n423 = property on="Magnetic Field (B)" class="Bool (strict)"() -> ("Value"=w815:bool)  [unwired: 2 in, 2 out]
                  n424 = property on="array for data" class="Arr (strict)"() -> ("Value"=w817:dbl[])  [unwired: 2 in, 2 out]
                  n425 = case shown="True" w815 {
                    tunnel: w817 -> [w818 w827]
                    tunnel: [w818 w826] -> w816
                    frame False {
                      # "we are not measuringmagnetic field (addr. 25)"
                    }
                    frame True {
                      w819 = 1
                      w824 = "25"
                      # "we are measuring magnetic field  (addr. 25)"
                      n426 = GPIB Write(0:w824, 1:"R 7", 2:w819) -> (6:w825:errorcluster)  [unwired: 2 in, 1 out]
                      n427 = GPIB Read(0:w824, 1:200, 2:w819, 3:w825) -> (5:w820:string)  [unwired: 1 in, 2 out]
                      n428 = Fract/Exp String To Number(string=w820, offset=w819) -> (number=w822:dbl)  [unwired: 2 in, 1 out]
                      n429 = Build Array (concatenate)(w827, w822) -> (w826:dbl[])
                    }
                  }
                  n430 = property on="array for data" class="Arr (strict)"("Value"=w816) -> ()  [unwired: 2 in, 2 out]
                }
                frame #25 {
                  # "check if capacitance\nand loss (address 28)\nare measured"
                  n431 = property on="Capacitance (C) and Loss (L)" class="Bool (strict)"() -> ("Value"=w828:bool)  [unwired: 2 in, 2 out]
                  n432 = property on="array for data" class="Arr (strict)"() -> ("Value"=w830:dbl[])  [unwired: 2 in, 2 out]
                  n433 = case shown="False" w828 {
                    tunnel: w830 -> [w831 w837]
                    tunnel: [w831 w833] -> w829
                    frame False {
                      # "we are not measuringmagnetic capacitance (addr. 28)"
                    }
                    frame True {
                      # "we are measuring capacitance and loss  (addr. 28)"
                      n434 = stacked-sequence {
                        seq-local: [w839 _ _] -> [_ _ w862]
                        tunnel: [_ _ w856] -> w832
                        tunnel: [_ _ w857] -> w835
                        tunnel: "28" ("data") -> [w838 w842 w851]
                        frame #0 {
                          n435 = GPIB Write(0:w838, 1:"SINGLE" ("data"), 2:i16 0 ("mode (0)")) -> (6:w839:errorcluster)  [unwired: 2 in, 1 out]
                        }
                        frame #1 {
                          n436 = while {
                            tunnel: w842 -> [w843]
                            i -> [w844]
                            stop <- w846 continue-if-true
                            n437 = GPIB Serial Poll(0:w843) -> (2:w848:i16)  [unwired: 1 in, 2 out]
                            n438 = Less?(x=w848, y=i16 128) -> (x < y?=w846:bool)
                            n439 = Wait (ms)(milliseconds to wait=u32 50) -> ()  [unwired: 1 out]
                            "Numeric" <- w844
                          }
                        }
                        frame #2 {
                          w849 = i16 2 ("mode (0)")
                          n440 = GPIB Read(0:w851, 1:200 ("byte count"), 2:i16 2 ("mode (0)"), 3:w862) -> (5:w855:string)  [unwired: 1 in, 2 out]
                          n441 = Match Pattern(string=w855, regular expression="C=") -> (after substring=w854:string)  [unwired: 1 in, 3 out]
                          n442 = Match Pattern(string=w854, regular expression="PF L=") -> (after substring=w852:string)  [unwired: 1 in, 3 out]
                          n443 = Search/Split String(string=w854, search string/char (-)=" ", offset (0)=w849) -> (substring before match=w859:string)  [unwired: 2 out]
                          n444 = Search/Split String(string=w852, search string/char (-)=" ", offset (0)=w849) -> (substring before match=w858:string)  [unwired: 2 out]
                          n445 = Fract/Exp String To Number(string=w858) -> (number=w856:dbl)  [unwired: 3 in, 1 out]
                          n446 = Fract/Exp String To Number(string=w859) -> (number=w857:dbl)  [unwired: 3 in, 1 out]
                        }
                      }
                      n447 = Build Array (concatenate)(w837, w835) -> (w834:dbl[])
                      n448 = Build Array (concatenate)(w834, w832) -> (w833:dbl[])
                    }
                  }
                  n449 = property on="array for data" class="Arr (strict)"("Value"=w829) -> ()  [unwired: 2 in, 2 out]
                }
              }
              n450 = flat-sequence {
                tunnel: w477 -> [_]
                frame #0 {
                  n451 = property on="Delib Time delay" class="DigNum (strict)"() -> ("Value"=w493:i32)  [unwired: 2 in, 2 out]
                  n452 = Wait (ms)(milliseconds to wait=w493) -> ()  [unwired: 1 out]
                }
              }
              n453 = case shown="\"Radio Selection 2\"" "Commute SorceMeter" {
                tunnel: ["13" "14"] -> w478
                frame "Radio Selection 1", Default {
                }
                frame "Radio Selection 2" {
                }
              }
              n454 = GPIB Write(0:w478, 1:":READ?", 3:w476) -> (6:w479:errorcluster)  [unwired: 2 in, 1 out]
              n455 = GPIB Read(0:w478, 1:3200, 3:w479) -> (5:w482:string)  [unwired: 2 in, 2 out]
              n456 = String Subset(string=w482, length (rest)=13) -> (substring=w483:string)  [unwired: 1 in]
              n457 = Fract/Exp String To Number(string=w483) -> (number=w485:dbl)  [unwired: 3 in, 1 out]
              n458 = Multiply(x=w485, y=-1.0) -> (x*y=w490:dbl)
              n459 = Number To Fractional String(number=w490) -> (F-format string=w487:string)  [unwired: 3 in]
              n460 = Concatenate Strings(":INIT:IMM; :SOUR:VOLT:LEV:IMM:AMPL " ("data"), w487) -> (w488:string)
              n461 = GPIB Write(0:w478, 1:w488) -> (6:w477:errorcluster)  [unwired: 3 in, 1 out]
            }
            frame #1 {
              n462 = stacked-sequence {
                tunnel: w881 -> [w884 _ _ _ _ _ _ _ _ _ _ _ _ _ _ _ _ _ _ _ _ _ _ _ _ _]
                tunnel: [w884 _ _ _ _ _ _ _ _ _ _ _ _ _ _ _ _ _ _ _ _ _ _ _ _ _] -> w867
                frame #0 {
                  # "check if oscillator on \nlock-in (address 1)\nis to be measured"
                  n463 = property on="Current is:" class="RadioBtnsControl (strict)"() -> ("Value"=w887:T1)  [unwired: 2 in, 2 out]
                  n464 = property on="array for data" class="Arr (strict)"() -> ("Value"=w886:dbl[])  [unwired: 2 in, 2 out]
                  n465 = Equal?(x=w887, y=1) -> (x = y?=w888:bool)
                  n466 = case shown="False" w888 {
                    tunnel: w886 -> [w890 w898]
                    tunnel: [w890 w897] -> w885
                    frame False {
                      # "we are not measuring oscillator from\nlock-in (address 1)"
                    }
                    frame True {
                      w894 = "1"
                      # "we are  measuring oscillator"
                      n467 = GPIB Write(0:w894, 1:"SLVL?") -> (6:w895:errorcluster)  [unwired: 3 in, 1 out]
                      n468 = GPIB Read(0:w894, 1:3200, 3:w895) -> (5:w892:string)  [unwired: 2 in, 2 out]
                      n469 = Fract/Exp String To Number(string=w892) -> (number=w891:dbl)  [unwired: 3 in, 1 out]
                      n470 = Build Array (concatenate)(w898, w891) -> (w897:dbl[])
                    }
                  }
                  n471 = property on="array for data" class="Arr (strict)"("Value"=w885) -> ()  [unwired: 2 in, 2 out]
                }
                frame #1 {
                  # "check if in-phase\nsignal on lock-in \n(address 1) is to\nbe measured"
                  n472 = property on="array for data" class="Arr (strict)"() -> ("Value"=w901:dbl[])  [unwired: 2 in, 2 out]
                  n473 = property on="Addr 1 lock-in" class="Bool (strict)"() -> ("Value"=w899:bool)  [unwired: 2 in, 2 out]
                  n474 = case shown="True" w899 {
                    tunnel: w901 -> [w902 w910]
                    tunnel: [w902 w909] -> w900
                    frame False {
                      # "we are not measuring in phase signal on lock-in (address 1)"
                    }
                    frame True {
                      w907 = "1"
                      # "we are  measuring lock-in (address 1), in phase"
                      n475 = GPIB Write(0:w907, 1:"OUTP?1") -> (6:w908:errorcluster)  [unwired: 3 in, 1 out]
                      n476 = GPIB Read(0:w907, 1:3200, 3:w908) -> (5:w905:string)  [unwired: 2 in, 2 out]
                      n477 = Fract/Exp String To Number(string=w905) -> (number=w904:dbl)  [unwired: 3 in, 1 out]
                      n478 = Build Array (concatenate)(w910, w904) -> (w909:dbl[])
                    }
                  }
                  n479 = property on="array for data" class="Arr (strict)"("Value"=w900) -> ()  [unwired: 2 in, 2 out]
                }
                frame #2 {
                  # "check if out-of-phase\nsignal on lock-in \n(address 1) is to\nbe measured"
                  n480 = property on="Addr 1 lock-in oop" class="Bool (strict)"() -> ("Value"=w911:bool)  [unwired: 2 in, 2 out]
                  n481 = property on="array for data" class="Arr (strict)"() -> ("Value"=w913:dbl[])  [unwired: 2 in, 2 out]
                  n482 = case shown="True" w911 {
                    tunnel: w913 -> [w914 w922]
                    tunnel: [w914 w921] -> w912
                    frame False {
                      # "we are not measuring out-of-phase signal on lock-in (address 1)"
                    }
                    frame True {
                      w919 = "1"
                      # "we are  measuring lock-in (address 1), out-of-phase signal"
                      n483 = GPIB Write(0:w919, 1:"OUTP?2") -> (6:w920:errorcluster)  [unwired: 3 in, 1 out]
                      n484 = GPIB Read(0:w919, 1:3200, 3:w920) -> (5:w917:string)  [unwired: 2 in, 2 out]
                      n485 = Fract/Exp String To Number(string=w917) -> (number=w916:dbl)  [unwired: 3 in, 1 out]
                      n486 = Build Array (concatenate)(w922, w916) -> (w921:dbl[])
                    }
                  }
                  n487 = property on="array for data" class="Arr (strict)"("Value"=w912) -> ()  [unwired: 2 in, 2 out]
                }
                frame #3 {
                  # "check if in-phase\nsignal on lock-in \n(address 2) is to\nbe measured"
                  n488 = property on="Addr 2 lock-in" class="Bool (strict)"() -> ("Value"=w923:bool)  [unwired: 2 in, 2 out]
                  n489 = property on="array for data" class="Arr (strict)"() -> ("Value"=w925:dbl[])  [unwired: 2 in, 2 out]
                  n490 = case shown="False" w923 {
                    tunnel: w925 -> [w926 w934]
                    tunnel: [w926 w933] -> w924
                    frame False {
                      # "we are not measuring in phase signal on lock-in (address 2)"
                    }
                    frame True {
                      w931 = "2"
                      # "we are  measuring lock-in (address 2), in phase"
                      n491 = GPIB Write(0:w931, 1:"OUTP?1") -> (6:w932:errorcluster)  [unwired: 3 in, 1 out]
                      n492 = GPIB Read(0:w931, 1:3200, 3:w932) -> (5:w929:string)  [unwired: 2 in, 2 out]
                      n493 = Fract/Exp String To Number(string=w929) -> (number=w928:dbl)  [unwired: 3 in, 1 out]
                      n494 = Build Array (concatenate)(w934, w928) -> (w933:dbl[])
                    }
                  }
                  n495 = property on="array for data" class="Arr (strict)"("Value"=w924) -> ()  [unwired: 2 in, 2 out]
                }
                frame #4 {
                  # "check if out-of-phase\nsignal on lock-in \n(address 2) is to\nbe measured"
                  n496 = property on="Addr 2 lock-in oop" class="Bool (strict)"() -> ("Value"=w935:bool)  [unwired: 2 in, 2 out]
                  n497 = property on="array for data" class="Arr (strict)"() -> ("Value"=w937:dbl[])  [unwired: 2 in, 2 out]
                  n498 = case shown="False" w935 {
                    tunnel: w937 -> [w938 w946]
                    tunnel: [w938 w945] -> w936
                    tunnel: w935 -> [_ _]
                    frame False {
                      # "we are not measuring out-of-phase signal on lock-in (address 2)"
                    }
                    frame True {
                      w943 = "2"
                      # "we are  measuring lock-in (address 2), out-of-phase"
                      n499 = GPIB Write(0:w943, 1:"OUTP?2") -> (6:w944:errorcluster)  [unwired: 3 in, 1 out]
                      n500 = GPIB Read(0:w943, 1:3200, 3:w944) -> (5:w941:string)  [unwired: 2 in, 2 out]
                      n501 = Fract/Exp String To Number(string=w941) -> (number=w940:dbl)  [unwired: 3 in, 1 out]
                      n502 = Build Array (concatenate)(w946, w940) -> (w945:dbl[])
                    }
                  }
                  n503 = property on="array for data" class="Arr (strict)"("Value"=w936) -> ()  [unwired: 2 in, 2 out]
                }
                frame #5 {
                  # "check if in-phase\nsignal on lock-in \n(address 3) is to\nbe measured"
                  n504 = property on="Addr 3 lock-in" class="Bool (strict)"() -> ("Value"=w947:bool)  [unwired: 2 in, 2 out]
                  n505 = property on="array for data" class="Arr (strict)"() -> ("Value"=w949:dbl[])  [unwired: 2 in, 2 out]
                  n506 = case shown="True" w947 {
                    tunnel: w949 -> [w950 w958]
                    tunnel: [w950 w957] -> w948
                    frame False {
                      # "we are not measuring in phase signal on lock-in (address 3)"
                    }
                    frame True {
                      w955 = "3"
                      # "we are  measuring lock-in (address 3), in phase"
                      n507 = GPIB Write(0:w955, 1:"OUTP?1") -> (6:w956:errorcluster)  [unwired: 3 in, 1 out]
                      n508 = GPIB Read(0:w955, 1:3200, 3:w956) -> (5:w953:string)  [unwired: 2 in, 2 out]
                      n509 = Fract/Exp String To Number(string=w953) -> (number=w952:dbl)  [unwired: 3 in, 1 out]
                      n510 = Build Array (concatenate)(w958, w952) -> (w957:dbl[])
                    }
                  }
                  n511 = property on="array for data" class="Arr (strict)"("Value"=w948) -> ()  [unwired: 2 in, 2 out]
                }
                frame #6 {
                  # "check if out-of-phase\nsignal on lock-in \n(address 3) is to\nbe measured"
                  n512 = property on="Addr 3 lock-in oop" class="Bool (strict)"() -> ("Value"=w959:bool)  [unwired: 2 in, 2 out]
                  n513 = property on="array for data" class="Arr (strict)"() -> ("Value"=w961:dbl[])  [unwired: 2 in, 2 out]
                  n514 = case shown="True" w959 {
                    tunnel: w961 -> [w962 w970]
                    tunnel: [w962 w969] -> w960
                    frame False {
                      # "we are not measuring out-of-phase signal on lock-in (address 3)"
                    }
                    frame True {
                      w967 = "3"
                      # "we are  measuring lock-in (address 3), out-of-phase"
                      n515 = GPIB Write(0:w967, 1:"OUTP?2") -> (6:w968:errorcluster)  [unwired: 3 in, 1 out]
                      n516 = GPIB Read(0:w967, 1:3200, 3:w968) -> (5:w965:string)  [unwired: 2 in, 2 out]
                      n517 = Fract/Exp String To Number(string=w965) -> (number=w964:dbl)  [unwired: 3 in, 1 out]
                      n518 = Build Array (concatenate)(w970, w964) -> (w969:dbl[])
                    }
                  }
                  n519 = property on="array for data" class="Arr (strict)"("Value"=w960) -> ()  [unwired: 2 in, 2 out]
                }
                frame #7 {
                  # "check if in-phase\nsignal on lock-in \n(address 4) is to\nbe measured"
                  n520 = property on="Addr 4 lock-in" class="Bool (strict)"() -> ("Value"=w971:bool)  [unwired: 2 in, 2 out]
                  n521 = property on="array for data" class="Arr (strict)"() -> ("Value"=w973:dbl[])  [unwired: 2 in, 2 out]
                  n522 = case shown="True" w971 {
                    tunnel: w973 -> [w974 w982]
                    tunnel: [w974 w981] -> w972
                    frame False {
                      # "we are not measuring in phase signal on lock-in (address 4)"
                    }
                    frame True {
                      w979 = "4"
                      # "we are  measuring lock-in (address 4), in phase"
                      n523 = GPIB Write(0:w979, 1:"OUTP?1") -> (6:w980:errorcluster)  [unwired: 3 in, 1 out]
                      n524 = GPIB Read(0:w979, 1:3200, 3:w980) -> (5:w977:string)  [unwired: 2 in, 2 out]
                      n525 = Fract/Exp String To Number(string=w977) -> (number=w976:dbl)  [unwired: 3 in, 1 out]
                      n526 = Build Array (concatenate)(w982, w976) -> (w981:dbl[])
                    }
                  }
                  n527 = property on="array for data" class="Arr (strict)"("Value"=w972) -> ()  [unwired: 2 in, 2 out]
                }
                frame #8 {
                  # "check if out-of-phase\nsignal on lock-in \n(address 4) is to\nbe measured"
                  n528 = property on="Addr 4 lock-in oop" class="Bool (strict)"() -> ("Value"=w983:bool)  [unwired: 2 in, 2 out]
                  n529 = property on="array for data" class="Arr (strict)"() -> ("Value"=w985:dbl[])  [unwired: 2 in, 2 out]
                  n530 = case shown="True" w983 {
                    tunnel: w985 -> [w986 w994]
                    tunnel: [w986 w993] -> w984
                    frame False {
                      # "we are not measuring out-of-phase signal on lock-in (address 4)"
                    }
                    frame True {
                      w991 = "4"
                      # "we are  measuring lock-in (address 4), out-of-phase"
                      n531 = GPIB Write(0:w991, 1:"OUTP?2") -> (6:w992:errorcluster)  [unwired: 3 in, 1 out]
                      n532 = GPIB Read(0:w991, 1:3200, 3:w992) -> (5:w989:string)  [unwired: 2 in, 2 out]
                      n533 = Fract/Exp String To Number(string=w989) -> (number=w988:dbl)  [unwired: 3 in, 1 out]
                      n534 = Build Array (concatenate)(w994, w988) -> (w993:dbl[])
                    }
                  }
                  n535 = property on="array for data" class="Arr (strict)"("Value"=w984) -> ()  [unwired: 2 in, 2 out]
                }
                frame #9 {
                  # "check if in-phase\nsignal on lock-in \n(address 5) is to\nbe measured"
                  n536 = property on="Addr 5 lock-in" class="Bool (strict)"() -> ("Value"=w995:bool)  [unwired: 2 in, 2 out]
                  n537 = property on="array for data" class="Arr (strict)"() -> ("Value"=w997:dbl[])  [unwired: 2 in, 2 out]
                  n538 = case shown="False" w995 {
                    tunnel: w997 -> [w998 w1006]
                    tunnel: [w998 w1005] -> w996
                    frame False {
                      # "we are not measuring in phase signal on lock-in (address 5)"
                    }
                    frame True {
                      w1003 = "5"
                      # "we are  measuring lock-in (address 5), in phase"
                      n539 = GPIB Write(0:w1003, 1:"OUTP?1") -> (6:w1004:errorcluster)  [unwired: 3 in, 1 out]
                      n540 = GPIB Read(0:w1003, 1:3200, 3:w1004) -> (5:w1001:string)  [unwired: 2 in, 2 out]
                      n541 = Fract/Exp String To Number(string=w1001) -> (number=w1000:dbl)  [unwired: 3 in, 1 out]
                      n542 = Build Array (concatenate)(w1006, w1000) -> (w1005:dbl[])
                    }
                  }
                  n543 = property on="array for data" class="Arr (strict)"("Value"=w996) -> ()  [unwired: 2 in, 2 out]
                }
                frame #10 {
                  # "check if out-of-phase\nsignal on lock-in \n(address 5) is to\nbe measured"
                  n544 = property on="Addr 5 lock-in oop" class="Bool (strict)"() -> ("Value"=w1007:bool)  [unwired: 2 in, 2 out]
                  n545 = property on="array for data" class="Arr (strict)"() -> ("Value"=w1009:dbl[])  [unwired: 2 in, 2 out]
                  n546 = case shown="False" w1007 {
                    tunnel: w1009 -> [w1010 w1018]
                    tunnel: [w1010 w1017] -> w1008
                    frame False {
                      # "we are not measuring out-of-phase signal on lock-in (address 5)"
                    }
                    frame True {
                      w1015 = "5"
                      # "we are  measuring lock-in (address 5), out-of-phase"
                      n547 = GPIB Write(0:w1015, 1:"OUTP?2") -> (6:w1016:errorcluster)  [unwired: 3 in, 1 out]
                      n548 = GPIB Read(0:w1015, 1:3200, 3:w1016) -> (5:w1013:string)  [unwired: 2 in, 2 out]
                      n549 = Fract/Exp String To Number(string=w1013) -> (number=w1012:dbl)  [unwired: 3 in, 1 out]
                      n550 = Build Array (concatenate)(w1018, w1012) -> (w1017:dbl[])
                    }
                  }
                  n551 = property on="array for data" class="Arr (strict)"("Value"=w1008) -> ()  [unwired: 2 in, 2 out]
                }
                frame #11 {
                  # "check if voltage on \nmain Keithley 2400 \n(addr. 12) is to\nbe measured"
                  n552 = property on="Voltage (Vk1)" class="Bool (strict)"() -> ("Value"=w1019:bool)  [unwired: 2 in, 2 out]
                  n553 = property on="array for data" class="Arr (strict)"() -> ("Value"=w1021:dbl[])  [unwired: 2 in, 2 out]
                  n554 = case shown="False" w1019 {
                    tunnel: w1021 -> [w1022 w1032]
                    tunnel: [w1022 w1031] -> w1020
                    frame False {
                      # "we aren't measuring voltage \non main Keithley 2400 (addr. 12)"
                    }
                    frame True {
                      w1029 = "12"
                      # "we are measuring voltage \non main Keithley 2400 (addr. 12)"
                      n555 = GPIB Write(0:w1029, 1:":READ?") -> (6:w1030:errorcluster)  [unwired: 3 in, 1 out]
                      n556 = GPIB Read(0:w1029, 1:3200, 3:w1030) -> (5:w1025:string)  [unwired: 2 in, 2 out]
                      n557 = String Subset(string=w1025, length (rest)=13) -> (substring=w1024:string)  [unwired: 1 in]
                      n558 = Fract/Exp String To Number(string=w1024) -> (number=w1027:dbl)  [unwired: 3 in, 1 out]
                      n559 = Build Array (concatenate)(w1032, w1027) -> (w1031:dbl[])
                    }
                  }
                  n560 = property on="array for data" class="Arr (strict)"("Value"=w1020) -> ()  [unwired: 2 in, 2 out]
                }
                frame #12 {
                  # "check if  current on \nmain Keithley 2400 \n(addr. 12) is to\nbe measured"
                  n561 = property on="Current (Ik1)" class="Bool (strict)"() -> ("Value"=w1033:bool)  [unwired: 2 in, 2 out]
                  n562 = property on="array for data" class="Arr (strict)"() -> ("Value"=w1035:dbl[])  [unwired: 2 in, 2 out]
                  n563 = case shown="True" w1033 {
                    tunnel: w1035 -> [w1036 w1047]
                    tunnel: [w1036 w1046] -> w1034
                    frame False {
                      # "we aren't measuring current \non main Keithley 2400 (addr. 12)"
                    }
                    frame True {
                      w1044 = "12"
                      # "we are measuring current\non main Keithley 2400 (addr. 12)"
                      n564 = GPIB Write(0:w1044, 1:":READ?") -> (6:w1045:errorcluster)  [unwired: 3 in, 1 out]
                      n565 = GPIB Read(0:w1044, 1:3200, 3:w1045) -> (5:w1040:string)  [unwired: 2 in, 2 out]
                      n566 = String Subset(string=w1040, offset (0)=14, length (rest)=13) -> (substring=w1039:string)
                      n567 = Fract/Exp String To Number(string=w1039) -> (number=w1042:dbl)  [unwired: 3 in, 1 out]
                      n568 = Build Array (concatenate)(w1047, w1042) -> (w1046:dbl[])
                    }
                  }
                  n569 = property on="array for data" class="Arr (strict)"("Value"=w1034) -> ()  [unwired: 2 in, 2 out]
                }
                frame #13 {
                  # "check if voltage on \nadd. Keithley 2400 \n(addr. 13) is to\nbe measured"
                  n570 = property on="Voltage (Vk2)" class="Bool (strict)"() -> ("Value"=w1048:bool)  [unwired: 2 in, 2 out]
                  n571 = property on="array for data" class="Arr (strict)"() -> ("Value"=w1050:dbl[])  [unwired: 2 in, 2 out]
                  n572 = case shown="True" w1048 {
                    tunnel: w1050 -> [w1051 w1061]
                    tunnel: [w1051 w1060] -> w1049
                    frame False {
                      # "we aren't measuring voltage \non additional Keithley 2400 (addr. 13)"
                    }
                    frame True {
                      w1058 = "13"
                      # "we are measuring voltage \non additional Keithley 2400 (addr. 13)"
                      n573 = GPIB Write(0:w1058, 1:":READ?") -> (6:w1059:errorcluster)  [unwired: 3 in, 1 out]
                      n574 = GPIB Read(0:w1058, 1:3200, 3:w1059) -> (5:w1054:string)  [unwired: 2 in, 2 out]
                      n575 = String Subset(string=w1054, length (rest)=13) -> (substring=w1053:string)  [unwired: 1 in]
                      n576 = Fract/Exp String To Number(string=w1053) -> (number=w1056:dbl)  [unwired: 3 in, 1 out]
                      n577 = Build Array (concatenate)(w1061, w1056) -> (w1060:dbl[])
                    }
                  }
                  n578 = property on="array for data" class="Arr (strict)"("Value"=w1049) -> ()  [unwired: 2 in, 2 out]
                }
                frame #14 {
                  # "check if  current on \nadd. Keithley 2400 \n(addr. 13) is to\nbe measured"
                  n579 = property on="Current (Ik2)" class="Bool (strict)"() -> ("Value"=w1062:bool)  [unwired: 2 in, 2 out]
                  n580 = property on="array for data" class="Arr (strict)"() -> ("Value"=w1064:dbl[])  [unwired: 2 in, 2 out]
                  n581 = case shown="True" w1062 {
                    tunnel: w1064 -> [w1065 w1076]
                    tunnel: [w1065 w1075] -> w1063
                    frame False {
                      # "we aren't measuring current \non additional Keithley 2400 (addr. 13)"
                    }
                    frame True {
                      w1073 = "13"
                      # "we are measuring current\non additional Keithley 2400 (addr. 13)"
                      n582 = GPIB Write(0:w1073, 1:":READ?") -> (6:w1074:errorcluster)  [unwired: 3 in, 1 out]
                      n583 = GPIB Read(0:w1073, 1:3200, 3:w1074) -> (5:w1069:string)  [unwired: 2 in, 2 out]
                      n584 = String Subset(string=w1069, offset (0)=14, length (rest)=13) -> (substring=w1068:string)
                      n585 = Fract/Exp String To Number(string=w1068) -> (number=w1071:dbl)  [unwired: 3 in, 1 out]
                      n586 = Build Array (concatenate)(w1076, w1071) -> (w1075:dbl[])
                    }
                  }
                  n587 = property on="array for data" class="Arr (strict)"("Value"=w1063) -> ()  [unwired: 2 in, 2 out]
                }
                frame #15 {
                  # "check if voltage on \nadd. Keithley 2400 \n(addr. 14) is to\nbe measured"
                  n588 = property on="Voltage (Vk3)" class="Bool (strict)"() -> ("Value"=w1077:bool)  [unwired: 2 in, 2 out]
                  n589 = property on="array for data" class="Arr (strict)"() -> ("Value"=w1079:dbl[])  [unwired: 2 in, 2 out]
                  n590 = case shown="False" w1077 {
                    tunnel: w1079 -> [w1080 w1090]
                    tunnel: [w1080 w1089] -> w1078
                    frame False {
                      # "we aren't measuring voltage \non additional Keithley 2400 (addr. 14)"
                    }
                    frame True {
                      w1087 = "14"
                      # "we are measuring voltage \non additional Keithley 2400 (addr. 14)"
                      n591 = GPIB Write(0:w1087, 1:":READ?") -> (6:w1088:errorcluster)  [unwired: 3 in, 1 out]
                      n592 = GPIB Read(0:w1087, 1:3200, 3:w1088) -> (5:w1083:string)  [unwired: 2 in, 2 out]
                      n593 = String Subset(string=w1083, length (rest)=13) -> (substring=w1082:string)  [unwired: 1 in]
                      n594 = Fract/Exp String To Number(string=w1082) -> (number=w1085:dbl)  [unwired: 3 in, 1 out]
                      n595 = Build Array (concatenate)(w1090, w1085) -> (w1089:dbl[])
                    }
                  }
                  n596 = property on="array for data" class="Arr (strict)"("Value"=w1078) -> ()  [unwired: 2 in, 2 out]
                }
                frame #16 {
                  # "check if  current on \nadd. Keithley 2400 \n(addr. 14) is to\nbe measured"
                  n597 = property on="Current (Ik3)" class="Bool (strict)"() -> ("Value"=w1091:bool)  [unwired: 2 in, 2 out]
                  n598 = property on="array for data" class="Arr (strict)"() -> ("Value"=w1093:dbl[])  [unwired: 2 in, 2 out]
                  n599 = case shown="True" w1091 {
                    tunnel: w1093 -> [w1094 w1105]
                    tunnel: [w1094 w1104] -> w1092
                    frame False {
                      # "we aren't measuring current \non additional Keithley 2400 (addr. 14)"
                    }
                    frame True {
                      w1102 = "14"
                      # "we are measuring current\non additional Keithley 2400 (addr. 14)"
                      n600 = GPIB Write(0:w1102, 1:":READ?") -> (6:w1103:errorcluster)  [unwired: 3 in, 1 out]
                      n601 = GPIB Read(0:w1102, 1:3200, 3:w1103) -> (5:w1098:string)  [unwired: 2 in, 2 out]
                      n602 = String Subset(string=w1098, offset (0)=14, length (rest)=13) -> (substring=w1097:string)
                      n603 = Fract/Exp String To Number(string=w1097) -> (number=w1100:dbl)  [unwired: 3 in, 1 out]
                      n604 = Build Array (concatenate)(w1105, w1100) -> (w1104:dbl[])
                    }
                  }
                  n605 = property on="array for data" class="Arr (strict)"("Value"=w1092) -> ()  [unwired: 2 in, 2 out]
                }
                frame #17 {
                  # "check if 1st channel\non Keithley 2182 \n(addr. 15) is to\nbe measured"
                  n606 = property on="Channel 1 (Vnano1)" class="Bool (strict)"() -> ("Value"=w1106:bool)  [unwired: 2 in, 2 out]
                  n607 = property on="array for data" class="Arr (strict)"() -> ("Value"=w1108:dbl[])  [unwired: 2 in, 2 out]
                  n608 = case shown="True" w1106 {
                    tunnel: w1108 -> [w1109 w1117]
                    tunnel: [w1109 w1116] -> w1107
                    frame False {
                      # "we are not measuring 1st channel\non Keithley 2182 (addr. 15)"
                    }
                    frame True {
                      w1114 = "15"
                      # "we are measuring 1st channel\non Keithley 2182 (addr. 15)"
                      n609 = GPIB Write(0:w1114, 1:":SENSe:DATA:FRES?") -> (6:w1115:errorcluster)  [unwired: 3 in, 1 out]
                      n610 = GPIB Read(0:w1114, 1:200, 3:w1115) -> (5:w1110:string)  [unwired: 2 in, 2 out]
                      n611 = Fract/Exp String To Number(string=w1110) -> (number=w1112:dbl)  [unwired: 3 in, 1 out]
                      n612 = Build Array (concatenate)(w1117, w1112) -> (w1116:dbl[])
                    }
                  }
                  n613 = property on="array for data" class="Arr (strict)"("Value"=w1107) -> ()  [unwired: 2 in, 2 out]
                }
                frame #18 {
                  # "check if 2nd channel\non Keithley 2182 \n(addr. 15) is to\nbe measured"
                  n614 = property on="Channel 2 (Vnano1b)" class="Bool (strict)"() -> ("Value"=w1118:bool)  [unwired: 2 in, 2 out]
                  n615 = property on="array for data" class="Arr (strict)"() -> ("Value"=w1120:dbl[])  [unwired: 2 in, 2 out]
                  n616 = case shown="False" w1118 {
                    tunnel: w1120 -> [w1121 w1133]
                    tunnel: [w1121 w1132] -> w1119
                    frame False {
                      # "we are not measuring 1st channel\non Keithley 2182 (addr. 15)"
                    }
                    frame True {
                      w1124 = "15"
                      # "switching to channel 2 and then\nback to channel 1"
                      # "we are measuring 2nd channel\non Keithley 2182 (addr. 15)"
                      n617 = GPIB Write(0:w1124, 1:":SENSe:CHAN 2") -> (6:w1125:errorcluster)  [unwired: 3 in, 1 out]
                      n618 = GPIB Write(0:w1124, 1:":SENSe:DATA:FRES?", 3:w1125) -> (6:w1131:errorcluster)  [unwired: 2 in, 1 out]
                      n619 = GPIB Read(0:w1124, 1:200, 3:w1131) -> (5:w1127:string, 7:w1123:errorcluster)  [unwired: 2 in, 1 out]
                      n620 = GPIB Write(0:w1124, 1:":SENSe:CHAN 1", 3:w1123) -> ()  [unwired: 2 in, 2 out]
                      n621 = Fract/Exp String To Number(string=w1127) -> (number=w1129:dbl)  [unwired: 3 in, 1 out]
                      n622 = Build Array (concatenate)(w1133, w1129) -> (w1132:dbl[])
                    }
                  }
                  n623 = property on="array for data" class="Arr (strict)"("Value"=w1119) -> ()  [unwired: 2 in, 2 out]
                }
                frame #19 {
                  # "check if 1st channel\non Keithley 2182 \n(addr. 16) is to\nbe measured"
                  n624 = property on="Channel 1 (Vnano2)" class="Bool (strict)"() -> ("Value"=w1134:bool)  [unwired: 2 in, 2 out]
                  n625 = property on="array for data" class="Arr (strict)"() -> ("Value"=w1136:dbl[])  [unwired: 2 in, 2 out]
                  n626 = case shown="True" w1134 {
                    tunnel: w1136 -> [w1137 w1145]
                    tunnel: [w1137 w1144] -> w1135
                    frame False {
                      # "we are not measuring 1st channel\non Keithley 2182 (addr. 16)"
                    }
                    frame True {
                      w1142 = "16"
                      # "we are measuring 1st channel\non Keithley 2182 (addr. 16)"
                      n627 = GPIB Write(0:w1142, 1:":SENSe:DATA:FRES?") -> (6:w1143:errorcluster)  [unwired: 3 in, 1 out]
                      n628 = GPIB Read(0:w1142, 1:200, 3:w1143) -> (5:w1138:string)  [unwired: 2 in, 2 out]
                      n629 = Fract/Exp String To Number(string=w1138) -> (number=w1140:dbl)  [unwired: 3 in, 1 out]
                      n630 = Build Array (concatenate)(w1145, w1140) -> (w1144:dbl[])
                    }
                  }
                  n631 = property on="array for data" class="Arr (strict)"("Value"=w1135) -> ()  [unwired: 2 in, 2 out]
                }
                frame #20 {
                  # "check if 2nd channel\non Keithley 2182 \n(addr. 16) is to\nbe measured"
                  n632 = property on="Channel 2 (Vnano2b)" class="Bool (strict)"() -> ("Value"=w1146:bool)  [unwired: 2 in, 2 out]
                  n633 = property on="array for data" class="Arr (strict)"() -> ("Value"=w1148:dbl[])  [unwired: 2 in, 2 out]
                  n634 = case shown="True" w1146 {
                    tunnel: w1148 -> [w1149 w1161]
                    tunnel: [w1149 w1160] -> w1147
                    frame False {
                      # "we are not measuring 1st channel\non Keithley 2182 (addr. 16)"
                    }
                    frame True {
                      w1152 = "16"
                      # "switching to channel 2 and then\nback to channel 1"
                      # "we are measuring 2nd channel\non Keithley 2182 (addr. 16)"
                      n635 = GPIB Write(0:w1152, 1:":SENSe:CHAN 2") -> (6:w1153:errorcluster)  [unwired: 3 in, 1 out]
                      n636 = GPIB Write(0:w1152, 1:":SENSe:DATA:FRES?", 3:w1153) -> (6:w1159:errorcluster)  [unwired: 2 in, 1 out]
                      n637 = GPIB Read(0:w1152, 1:200, 3:w1159) -> (5:w1155:string, 7:w1151:errorcluster)  [unwired: 2 in, 1 out]
                      n638 = GPIB Write(0:w1152, 1:":SENSe:CHAN 1", 3:w1151) -> ()  [unwired: 2 in, 2 out]
                      n639 = Fract/Exp String To Number(string=w1155) -> (number=w1157:dbl)  [unwired: 3 in, 1 out]
                      n640 = Build Array (concatenate)(w1161, w1157) -> (w1160:dbl[])
                    }
                  }
                  n641 = property on="array for data" class="Arr (strict)"("Value"=w1147) -> ()  [unwired: 2 in, 2 out]
                }
                frame #21 {
                  # "check if 1st channel\non Keithley 2182 \n(addr. 17) is to\nbe measured"
                  n642 = property on="Channel 1 (Vnano3)" class="Bool (strict)"() -> ("Value"=w1162:bool)  [unwired: 2 in, 2 out]
                  n643 = property on="array for data" class="Arr (strict)"() -> ("Value"=w1164:dbl[])  [unwired: 2 in, 2 out]
                  n644 = case shown="True" w1162 {
                    tunnel: w1164 -> [w1165 w1173]
                    tunnel: [w1165 w1172] -> w1163
                    frame False {
                      # "we are not measuring 1st channel\non Keithley 2182 (addr. 17)"
                    }
                    frame True {
                      w1170 = "17"
                      # "we are measuring 1st channel\non Keithley 2182 (addr. 17)"
                      n645 = GPIB Write(0:w1170, 1:":SENSe:DATA:FRES?") -> (6:w1171:errorcluster)  [unwired: 3 in, 1 out]
                      n646 = GPIB Read(0:w1170, 1:200, 3:w1171) -> (5:w1166:string)  [unwired: 2 in, 2 out]
                      n647 = Fract/Exp String To Number(string=w1166) -> (number=w1168:dbl)  [unwired: 3 in, 1 out]
                      n648 = Build Array (concatenate)(w1173, w1168) -> (w1172:dbl[])
                    }
                  }
                  n649 = property on="array for data" class="Arr (strict)"("Value"=w1163) -> ()  [unwired: 2 in, 2 out]
                }
                frame #22 {
                  # "check if 2nd channel\non Keithley 2182 \n(addr. 17) is to\nbe measured"
                  n650 = property on="Channel 2 (Vnano3b)" class="Bool (strict)"() -> ("Value"=w1174:bool)  [unwired: 2 in, 2 out]
                  n651 = property on="array for data" class="Arr (strict)"() -> ("Value"=w1176:dbl[])  [unwired: 2 in, 2 out]
                  n652 = case shown="True" w1174 {
                    tunnel: w1176 -> [w1177 w1189]
                    tunnel: [w1177 w1188] -> w1175
                    frame False {
                      # "we are not measuring 1st channel\non Keithley 2182 (addr. 17)"
                    }
                    frame True {
                      w1180 = "17"
                      # "switching to channel 2 and then\nback to channel 1"
                      # "we are measuring 2nd channel\non Keithley 2182 (addr. 17)"
                      n653 = GPIB Write(0:w1180, 1:":SENSe:CHAN 2") -> (6:w1181:errorcluster)  [unwired: 3 in, 1 out]
                      n654 = GPIB Write(0:w1180, 1:":SENSe:DATA:FRES?", 3:w1181) -> (6:w1187:errorcluster)  [unwired: 2 in, 1 out]
                      n655 = GPIB Read(0:w1180, 1:200, 3:w1187) -> (5:w1183:string, 7:w1179:errorcluster)  [unwired: 2 in, 1 out]
                      n656 = GPIB Write(0:w1180, 1:":SENSe:CHAN 1", 3:w1179) -> ()  [unwired: 2 in, 2 out]
                      n657 = Fract/Exp String To Number(string=w1183) -> (number=w1185:dbl)  [unwired: 3 in, 1 out]
                      n658 = Build Array (concatenate)(w1189, w1185) -> (w1188:dbl[])
                    }
                  }
                  n659 = property on="array for data" class="Arr (strict)"("Value"=w1175) -> ()  [unwired: 2 in, 2 out]
                }
                frame #23 {
                  # "check if 1st \nthermometer on \nOxford ITC \n(address 24) \nis measured"
                  n660 = property on="Thermometer 1 (T1)" class="Bool (strict)"() -> ("Value"=w1190:bool)  [unwired: 2 in, 2 out]
                  n661 = property on="array for data" class="Arr (strict)"() -> ("Value"=w1192:dbl[])  [unwired: 2 in, 2 out]
                  n662 = case shown="True" w1190 {
                    tunnel: w1192 -> [w1193 w1202]
                    tunnel: [w1193 w1201] -> w1191
                    frame False {
                      # "we are not measuring temperature on\nthermometer 1 (addr. 24)"
                    }
                    frame True {
                      w1194 = 1
                      w1199 = "24"
                      # "we are measuring temperature,\nthermometer 1 (addr. 24)"
                      n663 = GPIB Write(0:w1199, 1:"R 1", 2:w1194) -> (6:w1200:errorcluster)  [unwired: 2 in, 1 out]
                      n664 = GPIB Read(0:w1199, 1:200, 2:w1194, 3:w1200) -> (5:w1195:string)  [unwired: 1 in, 2 out]
                      n665 = Fract/Exp String To Number(string=w1195, offset=w1194) -> (number=w1197:dbl)  [unwired: 2 in, 1 out]
                      n666 = Build Array (concatenate)(w1202, w1197) -> (w1201:dbl[])
                    }
                  }
                  n667 = property on="array for data" class="Arr (strict)"("Value"=w1191) -> ()  [unwired: 2 in, 2 out]
                }
                frame #24 {
                  # "check if 1st \nthermometer on \nOxford ITC \n(address 24) \nis measured"
                  n668 = property on="Magnetic Field (B)" class="Bool (strict)"() -> ("Value"=w1203:bool)  [unwired: 2 in, 2 out]
                  n669 = property on="array for data" class="Arr (strict)"() -> ("Value"=w1205:dbl[])  [unwired: 2 in, 2 out]
                  n670 = case shown="True" w1203 {
                    tunnel: w1205 -> [w1206 w1215]
                    tunnel: [w1206 w1214] -> w1204
                    frame False {
                      # "we are not measuringmagnetic field (addr. 25)"
                    }
                    frame True {
                      w1207 = 1
                      w1212 = "25"
                      # "we are measuring magnetic field  (addr. 25)"
                      n671 = GPIB Write(0:w1212, 1:"R 8", 2:w1207) -> (6:w1213:errorcluster)  [unwired: 2 in, 1 out]
                      n672 = GPIB Read(0:w1212, 1:200, 2:w1207, 3:w1213) -> (5:w1208:string)  [unwired: 1 in, 2 out]
                      n673 = Fract/Exp String To Number(string=w1208, offset=w1207) -> (number=w1210:dbl)  [unwired: 2 in, 1 out]
                      n674 = Build Array (concatenate)(w1215, w1210) -> (w1214:dbl[])
                    }
                  }
                  n675 = property on="array for data" class="Arr (strict)"("Value"=w1204) -> ()  [unwired: 2 in, 2 out]
                }
                frame #25 {
                  # "check if capacitance\nand loss (address 28)\nare measured"
                  n676 = property on="Capacitance (C) and Loss (L)" class="Bool (strict)"() -> ("Value"=w1216:bool)  [unwired: 2 in, 2 out]
                  n677 = property on="array for data" class="Arr (strict)"() -> ("Value"=w1218:dbl[])  [unwired: 2 in, 2 out]
                  n678 = case shown="True" w1216 {
                    tunnel: w1218 -> [w1219 w1225]
                    tunnel: [w1219 w1221] -> w1217
                    frame False {
                      # "we are not measuringmagnetic capacitance (addr. 28)"
                    }
                    frame True {
                      # "we are measuring capacitance and loss  (addr. 28)"
                      n679 = stacked-sequence {
                        seq-local: [w1227 _ _] -> [_ _ w1250]
                        tunnel: [_ _ w1244] -> w1220
                        tunnel: [_ _ w1245] -> w1223
                        tunnel: "28" ("data") -> [w1226 w1230 w1239]
                        frame #0 {
                          n680 = GPIB Write(0:w1226, 1:"SINGLE" ("data"), 2:i16 0 ("mode (0)")) -> (6:w1227:errorcluster)  [unwired: 2 in, 1 out]
                        }
                        frame #1 {
                          n681 = while {
                            tunnel: w1230 -> [w1231]
                            i -> [w1232]
                            stop <- w1234 continue-if-true
                            n682 = GPIB Serial Poll(0:w1231) -> (2:w1236:i16)  [unwired: 1 in, 2 out]
                            n683 = Less?(x=w1236, y=i16 128) -> (x < y?=w1234:bool)
                            n684 = Wait (ms)(milliseconds to wait=u32 50) -> ()  [unwired: 1 out]
                            "Numeric 4" <- w1232
                          }
                        }
                        frame #2 {
                          w1237 = i16 2 ("mode (0)")
                          n685 = GPIB Read(0:w1239, 1:200 ("byte count"), 2:i16 2 ("mode (0)"), 3:w1250) -> (5:w1243:string)  [unwired: 1 in, 2 out]
                          n686 = Match Pattern(string=w1243, regular expression="C=") -> (after substring=w1242:string)  [unwired: 1 in, 3 out]
                          n687 = Match Pattern(string=w1242, regular expression="PF L=") -> (after substring=w1240:string)  [unwired: 1 in, 3 out]
                          n688 = Search/Split String(string=w1242, search string/char (-)=" ", offset (0)=w1237) -> (substring before match=w1247:string)  [unwired: 2 out]
                          n689 = Search/Split String(string=w1240, search string/char (-)=" ", offset (0)=w1237) -> (substring before match=w1246:string)  [unwired: 2 out]
                          n690 = Fract/Exp String To Number(string=w1246) -> (number=w1244:dbl)  [unwired: 3 in, 1 out]
                          n691 = Fract/Exp String To Number(string=w1247) -> (number=w1245:dbl)  [unwired: 3 in, 1 out]
                        }
                      }
                      n692 = Build Array (concatenate)(w1225, w1223) -> (w1222:dbl[])
                      n693 = Build Array (concatenate)(w1222, w1220) -> (w1221:dbl[])
                    }
                  }
                  n694 = property on="array for data" class="Arr (strict)"("Value"=w1217) -> ()  [unwired: 2 in, 2 out]
                }
              }
              n695 = property on="Commute SorceMeter" class="RadioBtnsControl (strict)"() -> ("Value"=w865:enum32{"Radio Selection 1", "Radio Selection 2"})  [unwired: 2 in, 2 out]
              n696 = case shown="\"Radio Selection 1\", Default" w865 {
                tunnel: ["13" "14"] -> w868
                frame "Radio Selection 1", Default {
                }
                frame "Radio Selection 2" {
                }
              }
              n697 = GPIB Write(0:w868, 1:":READ?", 3:w867) -> (6:w869:errorcluster)  [unwired: 2 in, 1 out]
              n698 = GPIB Read(0:w868, 1:3200, 3:w869) -> (5:w872:string)  [unwired: 2 in, 2 out]
              n699 = String Subset(string=w872, length (rest)=13) -> (substring=w873:string)  [unwired: 1 in]
              n700 = Fract/Exp String To Number(string=w873) -> (number=w875:dbl)  [unwired: 3 in, 1 out]
              n701 = Multiply(x=w875, y=-1.0) -> (x*y=w880:dbl)
              n702 = Number To Fractional String(number=w880) -> (F-format string=w877:string)  [unwired: 3 in]
              n703 = Concatenate Strings(":INIT:IMM; :SOUR:VOLT:LEV:IMM:AMPL " ("data"), w877) -> (w878:string)
              n704 = GPIB Write(0:w868, 1:w878) -> (6:w866:errorcluster)  [unwired: 3 in, 1 out]
            }
          }
        }
        frame False {
          # "all measurements are done in this stacked sequence; reading from each device is recorded to \"array for data\""
          n705 = stacked-sequence {
            tunnel: w1253 -> [w1255 _ _ _ _ _ _ _ _ _ _ _ _ _ _ _ _ _ _ _ _ _ _ _ _ _]
            tunnel: [w1255 _ _ _ _ _ _ _ _ _ _ _ _ _ _ _ _ _ _ _ _ _ _ _ _ _] -> w1254
            frame #0 {
              # "check if oscillator on \nlock-in (address 1)\nis to be measured"
              n706 = property on="Current is:" class="RadioBtnsControl (strict)"() -> ("Value"=w1258:T1)  [unwired: 2 in, 2 out]
              n707 = property on="array for data" class="Arr (strict)"() -> ("Value"=w1257:dbl[])  [unwired: 2 in, 2 out]
              n708 = Equal?(x=w1258, y=1) -> (x = y?=w1259:bool)
              n709 = case shown="True" w1259 {
                tunnel: w1257 -> [w1261 w1269]
                tunnel: [w1261 w1268] -> w1256
                frame False {
                  # "we are not measuring oscillator from\nlock-in (address 1)"
                }
                frame True {
                  w1265 = "1"
                  # "we are  measuring oscillator"
                  n710 = GPIB Write(0:w1265, 1:"SLVL?") -> (6:w1266:errorcluster)  [unwired: 3 in, 1 out]
                  n711 = GPIB Read(0:w1265, 1:3200, 3:w1266) -> (5:w1263:string)  [unwired: 2 in, 2 out]
                  n712 = Fract/Exp String To Number(string=w1263) -> (number=w1262:dbl)  [unwired: 3 in, 1 out]
                  n713 = Build Array (concatenate)(w1269, w1262) -> (w1268:dbl[])
                }
              }
              n714 = property on="array for data" class="Arr (strict)"("Value"=w1256) -> ()  [unwired: 2 in, 2 out]
            }
            frame #1 {
              # "check if in-phase\nsignal on lock-in \n(address 1) is to\nbe measured"
              n715 = property on="array for data" class="Arr (strict)"() -> ("Value"=w1272:dbl[])  [unwired: 2 in, 2 out]
              n716 = property on="Addr 1 lock-in" class="Bool (strict)"() -> ("Value"=w1270:bool)  [unwired: 2 in, 2 out]
              n717 = case shown="True" w1270 {
                tunnel: w1272 -> [w1273 w1281]
                tunnel: [w1273 w1280] -> w1271
                frame False {
                  # "we are not measuring in phase signal on lock-in (address 1)"
                }
                frame True {
                  w1278 = "1"
                  # "we are  measuring lock-in (address 1), in phase"
                  n718 = GPIB Write(0:w1278, 1:"OUTP?1") -> (6:w1279:errorcluster)  [unwired: 3 in, 1 out]
                  n719 = GPIB Read(0:w1278, 1:3200, 3:w1279) -> (5:w1276:string)  [unwired: 2 in, 2 out]
                  n720 = Fract/Exp String To Number(string=w1276) -> (number=w1275:dbl)  [unwired: 3 in, 1 out]
                  n721 = Build Array (concatenate)(w1281, w1275) -> (w1280:dbl[])
                }
              }
              n722 = property on="array for data" class="Arr (strict)"("Value"=w1271) -> ()  [unwired: 2 in, 2 out]
            }
            frame #2 {
              # "check if out-of-phase\nsignal on lock-in \n(address 1) is to\nbe measured"
              n723 = property on="Addr 1 lock-in oop" class="Bool (strict)"() -> ("Value"=w1282:bool)  [unwired: 2 in, 2 out]
              n724 = property on="array for data" class="Arr (strict)"() -> ("Value"=w1284:dbl[])  [unwired: 2 in, 2 out]
              n725 = case shown="True" w1282 {
                tunnel: w1284 -> [w1285 w1293]
                tunnel: [w1285 w1292] -> w1283
                frame False {
                  # "we are not measuring out-of-phase signal on lock-in (address 1)"
                }
                frame True {
                  w1290 = "1"
                  # "we are  measuring lock-in (address 1), out-of-phase signal"
                  n726 = GPIB Write(0:w1290, 1:"OUTP?2") -> (6:w1291:errorcluster)  [unwired: 3 in, 1 out]
                  n727 = GPIB Read(0:w1290, 1:3200, 3:w1291) -> (5:w1288:string)  [unwired: 2 in, 2 out]
                  n728 = Fract/Exp String To Number(string=w1288) -> (number=w1287:dbl)  [unwired: 3 in, 1 out]
                  n729 = Build Array (concatenate)(w1293, w1287) -> (w1292:dbl[])
                }
              }
              n730 = property on="array for data" class="Arr (strict)"("Value"=w1283) -> ()  [unwired: 2 in, 2 out]
            }
            frame #3 {
              # "check if in-phase\nsignal on lock-in \n(address 2) is to\nbe measured"
              n731 = property on="Addr 2 lock-in" class="Bool (strict)"() -> ("Value"=w1294:bool)  [unwired: 2 in, 2 out]
              n732 = property on="array for data" class="Arr (strict)"() -> ("Value"=w1296:dbl[])  [unwired: 2 in, 2 out]
              n733 = case shown="True" w1294 {
                tunnel: w1296 -> [w1297 w1305]
                tunnel: [w1297 w1304] -> w1295
                frame False {
                  # "we are not measuring in phase signal on lock-in (address 2)"
                }
                frame True {
                  w1302 = "2"
                  # "we are  measuring lock-in (address 2), in phase"
                  n734 = GPIB Write(0:w1302, 1:"OUTP?1") -> (6:w1303:errorcluster)  [unwired: 3 in, 1 out]
                  n735 = GPIB Read(0:w1302, 1:3200, 3:w1303) -> (5:w1300:string)  [unwired: 2 in, 2 out]
                  n736 = Fract/Exp String To Number(string=w1300) -> (number=w1299:dbl)  [unwired: 3 in, 1 out]
                  n737 = Build Array (concatenate)(w1305, w1299) -> (w1304:dbl[])
                }
              }
              n738 = property on="array for data" class="Arr (strict)"("Value"=w1295) -> ()  [unwired: 2 in, 2 out]
            }
            frame #4 {
              # "check if out-of-phase\nsignal on lock-in \n(address 2) is to\nbe measured"
              n739 = property on="Addr 2 lock-in oop" class="Bool (strict)"() -> ("Value"=w1306:bool)  [unwired: 2 in, 2 out]
              n740 = property on="array for data" class="Arr (strict)"() -> ("Value"=w1308:dbl[])  [unwired: 2 in, 2 out]
              n741 = case shown="True" w1306 {
                tunnel: w1308 -> [w1309 w1317]
                tunnel: [w1309 w1316] -> w1307
                tunnel: w1306 -> [_ _]
                frame False {
                  # "we are not measuring out-of-phase signal on lock-in (address 2)"
                }
                frame True {
                  w1314 = "2"
                  # "we are  measuring lock-in (address 2), out-of-phase"
                  n742 = GPIB Write(0:w1314, 1:"OUTP?2") -> (6:w1315:errorcluster)  [unwired: 3 in, 1 out]
                  n743 = GPIB Read(0:w1314, 1:3200, 3:w1315) -> (5:w1312:string)  [unwired: 2 in, 2 out]
                  n744 = Fract/Exp String To Number(string=w1312) -> (number=w1311:dbl)  [unwired: 3 in, 1 out]
                  n745 = Build Array (concatenate)(w1317, w1311) -> (w1316:dbl[])
                }
              }
              n746 = property on="array for data" class="Arr (strict)"("Value"=w1307) -> ()  [unwired: 2 in, 2 out]
            }
            frame #5 {
              # "check if in-phase\nsignal on lock-in \n(address 3) is to\nbe measured"
              n747 = property on="Addr 3 lock-in" class="Bool (strict)"() -> ("Value"=w1318:bool)  [unwired: 2 in, 2 out]
              n748 = property on="array for data" class="Arr (strict)"() -> ("Value"=w1320:dbl[])  [unwired: 2 in, 2 out]
              n749 = case shown="False" w1318 {
                tunnel: w1320 -> [w1321 w1329]
                tunnel: [w1321 w1328] -> w1319
                frame False {
                  # "we are not measuring in phase signal on lock-in (address 3)"
                }
                frame True {
                  w1326 = "3"
                  # "we are  measuring lock-in (address 3), in phase"
                  n750 = GPIB Write(0:w1326, 1:"OUTP?1") -> (6:w1327:errorcluster)  [unwired: 3 in, 1 out]
                  n751 = GPIB Read(0:w1326, 1:3200, 3:w1327) -> (5:w1324:string)  [unwired: 2 in, 2 out]
                  n752 = Fract/Exp String To Number(string=w1324) -> (number=w1323:dbl)  [unwired: 3 in, 1 out]
                  n753 = Build Array (concatenate)(w1329, w1323) -> (w1328:dbl[])
                }
              }
              n754 = property on="array for data" class="Arr (strict)"("Value"=w1319) -> ()  [unwired: 2 in, 2 out]
            }
            frame #6 {
              # "check if out-of-phase\nsignal on lock-in \n(address 3) is to\nbe measured"
              n755 = property on="Addr 3 lock-in oop" class="Bool (strict)"() -> ("Value"=w1330:bool)  [unwired: 2 in, 2 out]
              n756 = property on="array for data" class="Arr (strict)"() -> ("Value"=w1332:dbl[])  [unwired: 2 in, 2 out]
              n757 = case shown="False" w1330 {
                tunnel: w1332 -> [w1333 w1341]
                tunnel: [w1333 w1340] -> w1331
                frame False {
                  # "we are not measuring out-of-phase signal on lock-in (address 3)"
                }
                frame True {
                  w1338 = "3"
                  # "we are  measuring lock-in (address 3), out-of-phase"
                  n758 = GPIB Write(0:w1338, 1:"OUTP?2") -> (6:w1339:errorcluster)  [unwired: 3 in, 1 out]
                  n759 = GPIB Read(0:w1338, 1:3200, 3:w1339) -> (5:w1336:string)  [unwired: 2 in, 2 out]
                  n760 = Fract/Exp String To Number(string=w1336) -> (number=w1335:dbl)  [unwired: 3 in, 1 out]
                  n761 = Build Array (concatenate)(w1341, w1335) -> (w1340:dbl[])
                }
              }
              n762 = property on="array for data" class="Arr (strict)"("Value"=w1331) -> ()  [unwired: 2 in, 2 out]
            }
            frame #7 {
              # "check if in-phase\nsignal on lock-in \n(address 4) is to\nbe measured"
              n763 = property on="Addr 4 lock-in" class="Bool (strict)"() -> ("Value"=w1342:bool)  [unwired: 2 in, 2 out]
              n764 = property on="array for data" class="Arr (strict)"() -> ("Value"=w1344:dbl[])  [unwired: 2 in, 2 out]
              n765 = case shown="False" w1342 {
                tunnel: w1344 -> [w1345 w1353]
                tunnel: [w1345 w1352] -> w1343
                frame False {
                  # "we are not measuring in phase signal on lock-in (address 4)"
                }
                frame True {
                  w1350 = "4"
                  # "we are  measuring lock-in (address 4), in phase"
                  n766 = GPIB Write(0:w1350, 1:"OUTP?1") -> (6:w1351:errorcluster)  [unwired: 3 in, 1 out]
                  n767 = GPIB Read(0:w1350, 1:3200, 3:w1351) -> (5:w1348:string)  [unwired: 2 in, 2 out]
                  n768 = Fract/Exp String To Number(string=w1348) -> (number=w1347:dbl)  [unwired: 3 in, 1 out]
                  n769 = Build Array (concatenate)(w1353, w1347) -> (w1352:dbl[])
                }
              }
              n770 = property on="array for data" class="Arr (strict)"("Value"=w1343) -> ()  [unwired: 2 in, 2 out]
            }
            frame #8 {
              # "check if out-of-phase\nsignal on lock-in \n(address 4) is to\nbe measured"
              n771 = property on="Addr 4 lock-in oop" class="Bool (strict)"() -> ("Value"=w1354:bool)  [unwired: 2 in, 2 out]
              n772 = property on="array for data" class="Arr (strict)"() -> ("Value"=w1356:dbl[])  [unwired: 2 in, 2 out]
              n773 = case shown="False" w1354 {
                tunnel: w1356 -> [w1357 w1365]
                tunnel: [w1357 w1364] -> w1355
                frame False {
                  # "we are not measuring out-of-phase signal on lock-in (address 4)"
                }
                frame True {
                  w1362 = "4"
                  # "we are  measuring lock-in (address 4), out-of-phase"
                  n774 = GPIB Write(0:w1362, 1:"OUTP?2") -> (6:w1363:errorcluster)  [unwired: 3 in, 1 out]
                  n775 = GPIB Read(0:w1362, 1:3200, 3:w1363) -> (5:w1360:string)  [unwired: 2 in, 2 out]
                  n776 = Fract/Exp String To Number(string=w1360) -> (number=w1359:dbl)  [unwired: 3 in, 1 out]
                  n777 = Build Array (concatenate)(w1365, w1359) -> (w1364:dbl[])
                }
              }
              n778 = property on="array for data" class="Arr (strict)"("Value"=w1355) -> ()  [unwired: 2 in, 2 out]
            }
            frame #9 {
              # "check if in-phase\nsignal on lock-in \n(address 5) is to\nbe measured"
              n779 = property on="Addr 5 lock-in" class="Bool (strict)"() -> ("Value"=w1366:bool)  [unwired: 2 in, 2 out]
              n780 = property on="array for data" class="Arr (strict)"() -> ("Value"=w1368:dbl[])  [unwired: 2 in, 2 out]
              n781 = case shown="False" w1366 {
                tunnel: w1368 -> [w1369 w1377]
                tunnel: [w1369 w1376] -> w1367
                frame False {
                  # "we are not measuring in phase signal on lock-in (address 5)"
                }
                frame True {
                  w1374 = "5"
                  # "we are  measuring lock-in (address 5), in phase"
                  n782 = GPIB Write(0:w1374, 1:"OUTP?1") -> (6:w1375:errorcluster)  [unwired: 3 in, 1 out]
                  n783 = GPIB Read(0:w1374, 1:3200, 3:w1375) -> (5:w1372:string)  [unwired: 2 in, 2 out]
                  n784 = Fract/Exp String To Number(string=w1372) -> (number=w1371:dbl)  [unwired: 3 in, 1 out]
                  n785 = Build Array (concatenate)(w1377, w1371) -> (w1376:dbl[])
                }
              }
              n786 = property on="array for data" class="Arr (strict)"("Value"=w1367) -> ()  [unwired: 2 in, 2 out]
            }
            frame #10 {
              # "check if out-of-phase\nsignal on lock-in \n(address 5) is to\nbe measured"
              n787 = property on="Addr 5 lock-in oop" class="Bool (strict)"() -> ("Value"=w1378:bool)  [unwired: 2 in, 2 out]
              n788 = property on="array for data" class="Arr (strict)"() -> ("Value"=w1380:dbl[])  [unwired: 2 in, 2 out]
              n789 = case shown="False" w1378 {
                tunnel: w1380 -> [w1381 w1389]
                tunnel: [w1381 w1388] -> w1379
                frame False {
                  # "we are not measuring out-of-phase signal on lock-in (address 5)"
                }
                frame True {
                  w1386 = "5"
                  # "we are  measuring lock-in (address 5), out-of-phase"
                  n790 = GPIB Write(0:w1386, 1:"OUTP?2") -> (6:w1387:errorcluster)  [unwired: 3 in, 1 out]
                  n791 = GPIB Read(0:w1386, 1:3200, 3:w1387) -> (5:w1384:string)  [unwired: 2 in, 2 out]
                  n792 = Fract/Exp String To Number(string=w1384) -> (number=w1383:dbl)  [unwired: 3 in, 1 out]
                  n793 = Build Array (concatenate)(w1389, w1383) -> (w1388:dbl[])
                }
              }
              n794 = property on="array for data" class="Arr (strict)"("Value"=w1379) -> ()  [unwired: 2 in, 2 out]
            }
            frame #11 {
              # "check if voltage on \nChannel A of main\nKeithley 2614B \n(addr. 12) is to\nbe measured"
              n795 = property on="Voltage (Vk1)" class="Bool (strict)"() -> ("Value"=w1390:bool)  [unwired: 2 in, 2 out]
              n796 = property on="array for data" class="Arr (strict)"() -> ("Value"=w1392:dbl[])  [unwired: 2 in, 2 out]
              n797 = case shown="True" w1390 {
                tunnel: w1392 -> [w1393 w1401]
                tunnel: [w1393 w1400] -> w1391
                frame False {
                  # "we aren't measuring voltage \non main Keithley 2614B Channel A (addr. 12)"
                }
                frame True {
                  (unwired) 13
                  w1398 = "12"
                  # "we are measuring voltage of Channel A \non the main Keithley 2614B (addr. 12)"
                  n798 = GPIB Write(0:w1398, 1:"print(smua.measure.v())") -> (6:w1399:errorcluster)  [unwired: 3 in, 1 out]
                  n799 = GPIB Read(0:w1398, 1:3200, 3:w1399) -> (5:w1394:string)  [unwired: 2 in, 2 out]
                  n800 = Fract/Exp String To Number(string=w1394) -> (number=w1396:dbl)  [unwired: 3 in, 1 out]
                  n801 = Build Array (concatenate)(w1401, w1396) -> (w1400:dbl[])
                }
              }
              n802 = property on="array for data" class="Arr (strict)"("Value"=w1391) -> ()  [unwired: 2 in, 2 out]
            }
            frame #12 {
              # "check if current on \nChannel A of main\nKeithley 2614B \n(addr. 12) is to\nbe measured"
              n803 = property on="Current (Ik1)" class="Bool (strict)"() -> ("Value"=w1402:bool)  [unwired: 2 in, 2 out]
              n804 = property on="array for data" class="Arr (strict)"() -> ("Value"=w1404:dbl[])  [unwired: 2 in, 2 out]
              n805 = case shown="True" w1402 {
                tunnel: w1404 -> [w1405 w1407]
                tunnel: [w1405 w1406] -> w1403
                frame False {
                  # "we aren't measuring current \non main Keithley 2400 (addr. 12)"
                }
                frame True {
                  w1412 = "12"
                  # "we are measuring current of Channel A \non the main Keithley 2614B (addr. 12)"
                  n806 = GPIB Write(0:w1412, 1:"print(smua.measure.i())") -> (6:w1413:errorcluster)  [unwired: 3 in, 1 out]
                  n807 = GPIB Read(0:w1412, 1:3200, 3:w1413) -> (5:w1408:string)  [unwired: 2 in, 2 out]
                  n808 = Fract/Exp String To Number(string=w1408) -> (number=w1410:dbl)  [unwired: 3 in, 1 out]
                  n809 = Build Array (concatenate)(w1407, w1410) -> (w1406:dbl[])
                }
              }
              n810 = property on="array for data" class="Arr (strict)"("Value"=w1403) -> ()  [unwired: 2 in, 2 out]
            }
            frame #13 {
              # "check if voltage on \nChannel B of main\nKeithley 2614B \n(addr. 12) is to\nbe measured"
              n811 = property on="Voltage (Vk2)" class="Bool (strict)"() -> ("Value"=w1414:bool)  [unwired: 2 in, 2 out]
              n812 = property on="array for data" class="Arr (strict)"() -> ("Value"=w1416:dbl[])  [unwired: 2 in, 2 out]
              n813 = case shown="True" w1414 {
                tunnel: w1416 -> [w1417 w1419]
                tunnel: [w1417 w1418] -> w1415
                frame False {
                  # "we aren't measuring voltage \non additional Keithley 2400 (addr. 13)"
                }
                frame True {
                  w1424 = "12"
                  # "we are measuring voltage of Channel B \non the main Keithley 2614B (addr. 12)"
                  n814 = GPIB Write(0:w1424, 1:"print(smub.measure.v())") -> (6:w1425:errorcluster)  [unwired: 3 in, 1 out]
                  n815 = GPIB Read(0:w1424, 1:3200, 3:w1425) -> (5:w1420:string)  [unwired: 2 in, 2 out]
                  n816 = Fract/Exp String To Number(string=w1420) -> (number=w1422:dbl)  [unwired: 3 in, 1 out]
                  n817 = Build Array (concatenate)(w1419, w1422) -> (w1418:dbl[])
                }
              }
              n818 = property on="array for data" class="Arr (strict)"("Value"=w1415) -> ()  [unwired: 2 in, 2 out]
            }
            frame #14 {
              # "check if current on \nChannel B of main\nKeithley 2614B \n(addr. 12) is to\nbe measured"
              n819 = property on="Current (Ik2)" class="Bool (strict)"() -> ("Value"=w1426:bool)  [unwired: 2 in, 2 out]
              n820 = property on="array for data" class="Arr (strict)"() -> ("Value"=w1428:dbl[])  [unwired: 2 in, 2 out]
              n821 = case shown="False" w1426 {
                tunnel: w1428 -> [w1429 w1431]
                tunnel: [w1429 w1430] -> w1427
                frame False {
                  # "we aren't measuring current \non additional Keithley 2400 (addr. 13)"
                }
                frame True {
                  w1436 = "12"
                  # "we are measuring current of Channel B \non the main Keithley 2614B (addr. 12)"
                  n822 = GPIB Write(0:w1436, 1:"print(smub.measure.i())") -> (6:w1437:errorcluster)  [unwired: 3 in, 1 out]
                  n823 = GPIB Read(0:w1436, 1:3200, 3:w1437) -> (5:w1432:string)  [unwired: 2 in, 2 out]
                  n824 = Fract/Exp String To Number(string=w1432) -> (number=w1434:dbl)  [unwired: 3 in, 1 out]
                  n825 = Build Array (concatenate)(w1431, w1434) -> (w1430:dbl[])
                }
              }
              n826 = property on="array for data" class="Arr (strict)"("Value"=w1427) -> ()  [unwired: 2 in, 2 out]
            }
            frame #15 {
              # "check if voltage on \nadd. Keithley 2400 \n(addr. 14) is to\nbe measured"
              n827 = property on="Voltage (Vk3)" class="Bool (strict)"() -> ("Value"=w1438:bool)  [unwired: 2 in, 2 out]
              n828 = property on="array for data" class="Arr (strict)"() -> ("Value"=w1440:dbl[])  [unwired: 2 in, 2 out]
              n829 = case shown="False" w1438 {
                tunnel: w1440 -> [w1441 w1451]
                tunnel: [w1441 w1450] -> w1439
                frame False {
                  # "we aren't measuring voltage \non additional Keithley 2400 (addr. 14)"
                }
                frame True {
                  w1448 = "14"
                  # "we are measuring voltage \non additional Keithley 2400 (addr. 14)"
                  n830 = GPIB Write(0:w1448, 1:":READ?") -> (6:w1449:errorcluster)  [unwired: 3 in, 1 out]
                  n831 = GPIB Read(0:w1448, 1:3200, 3:w1449) -> (5:w1444:string)  [unwired: 2 in, 2 out]
                  n832 = String Subset(string=w1444, length (rest)=13) -> (substring=w1443:string)  [unwired: 1 in]
                  n833 = Fract/Exp String To Number(string=w1443) -> (number=w1446:dbl)  [unwired: 3 in, 1 out]
                  n834 = Build Array (concatenate)(w1451, w1446) -> (w1450:dbl[])
                }
              }
              n835 = property on="array for data" class="Arr (strict)"("Value"=w1439) -> ()  [unwired: 2 in, 2 out]
            }
            frame #16 {
              # "check if  current on \nadd. Keithley 2400 \n(addr. 14) is to\nbe measured"
              n836 = property on="Current (Ik3)" class="Bool (strict)"() -> ("Value"=w1452:bool)  [unwired: 2 in, 2 out]
              n837 = property on="array for data" class="Arr (strict)"() -> ("Value"=w1454:dbl[])  [unwired: 2 in, 2 out]
              n838 = case shown="False" w1452 {
                tunnel: w1454 -> [w1455 w1466]
                tunnel: [w1455 w1465] -> w1453
                frame False {
                  # "we aren't measuring current \non additional Keithley 2400 (addr. 14)"
                }
                frame True {
                  w1463 = "14"
                  # "we are measuring current\non additional Keithley 2400 (addr. 14)"
                  n839 = GPIB Write(0:w1463, 1:":READ?") -> (6:w1464:errorcluster)  [unwired: 3 in, 1 out]
                  n840 = GPIB Read(0:w1463, 1:3200, 3:w1464) -> (5:w1459:string)  [unwired: 2 in, 2 out]
                  n841 = String Subset(string=w1459, offset (0)=14, length (rest)=13) -> (substring=w1458:string)
                  n842 = Fract/Exp String To Number(string=w1458) -> (number=w1461:dbl)  [unwired: 3 in, 1 out]
                  n843 = Build Array (concatenate)(w1466, w1461) -> (w1465:dbl[])
                }
              }
              n844 = property on="array for data" class="Arr (strict)"("Value"=w1453) -> ()  [unwired: 2 in, 2 out]
            }
            frame #17 {
              # "check if 1st channel\non Keithley 2182 \n(addr. 15) is to\nbe measured"
              n845 = property on="Channel 1 (Vnano1)" class="Bool (strict)"() -> ("Value"=w1467:bool)  [unwired: 2 in, 2 out]
              n846 = property on="array for data" class="Arr (strict)"() -> ("Value"=w1469:dbl[])  [unwired: 2 in, 2 out]
              n847 = case shown="True" w1467 {
                tunnel: w1469 -> [w1470 w1478]
                tunnel: [w1470 w1477] -> w1468
                frame False {
                  # "we are not measuring 1st channel\non Keithley 2182 (addr. 15)"
                }
                frame True {
                  w1475 = "15"
                  # "we are measuring 1st channel\non Keithley 2182 (addr. 15)"
                  n848 = GPIB Write(0:w1475, 1:":SENSe:DATA:FRES?") -> (6:w1476:errorcluster)  [unwired: 3 in, 1 out]
                  n849 = GPIB Read(0:w1475, 1:200, 3:w1476) -> (5:w1471:string)  [unwired: 2 in, 2 out]
                  n850 = Fract/Exp String To Number(string=w1471) -> (number=w1473:dbl)  [unwired: 3 in, 1 out]
                  n851 = Build Array (concatenate)(w1478, w1473) -> (w1477:dbl[])
                }
              }
              n852 = property on="array for data" class="Arr (strict)"("Value"=w1468) -> ()  [unwired: 2 in, 2 out]
            }
            frame #18 {
              # "check if 2nd channel\non Keithley 2182 \n(addr. 15) is to\nbe measured"
              n853 = property on="Channel 2 (Vnano1b)" class="Bool (strict)"() -> ("Value"=w1479:bool)  [unwired: 2 in, 2 out]
              n854 = property on="array for data" class="Arr (strict)"() -> ("Value"=w1481:dbl[])  [unwired: 2 in, 2 out]
              n855 = case shown="True" w1479 {
                tunnel: w1481 -> [w1482 w1494]
                tunnel: [w1482 w1493] -> w1480
                frame False {
                  # "we are not measuring 1st channel\non Keithley 2182 (addr. 15)"
                }
                frame True {
                  w1485 = "15"
                  # "switching to channel 2 and then\nback to channel 1"
                  # "we are measuring 2nd channel\non Keithley 2182 (addr. 15)"
                  n856 = GPIB Write(0:w1485, 1:":SENSe:CHAN 2") -> (6:w1486:errorcluster)  [unwired: 3 in, 1 out]
                  n857 = GPIB Write(0:w1485, 1:":SENSe:DATA:FRES?", 3:w1486) -> (6:w1492:errorcluster)  [unwired: 2 in, 1 out]
                  n858 = GPIB Read(0:w1485, 1:200, 3:w1492) -> (5:w1488:string, 7:w1484:errorcluster)  [unwired: 2 in, 1 out]
                  n859 = GPIB Write(0:w1485, 1:":SENSe:CHAN 1", 3:w1484) -> ()  [unwired: 2 in, 2 out]
                  n860 = Fract/Exp String To Number(string=w1488) -> (number=w1490:dbl)  [unwired: 3 in, 1 out]
                  n861 = Build Array (concatenate)(w1494, w1490) -> (w1493:dbl[])
                }
              }
              n862 = property on="array for data" class="Arr (strict)"("Value"=w1480) -> ()  [unwired: 2 in, 2 out]
            }
            frame #19 {
              # "check if 1st channel\non Keithley 2182 \n(addr. 16) is to\nbe measured"
              n863 = property on="Channel 1 (Vnano2)" class="Bool (strict)"() -> ("Value"=w1495:bool)  [unwired: 2 in, 2 out]
              n864 = property on="array for data" class="Arr (strict)"() -> ("Value"=w1497:dbl[])  [unwired: 2 in, 2 out]
              n865 = case shown="True" w1495 {
                tunnel: w1497 -> [w1498 w1506]
                tunnel: [w1498 w1505] -> w1496
                frame False {
                  # "we are not measuring 1st channel\non Keithley 2182 (addr. 16)"
                }
                frame True {
                  w1503 = "16"
                  # "we are measuring 1st channel\non Keithley 2182 (addr. 16)"
                  n866 = GPIB Write(0:w1503, 1:":SENSe:DATA:FRES?") -> (6:w1504:errorcluster)  [unwired: 3 in, 1 out]
                  n867 = GPIB Read(0:w1503, 1:200, 3:w1504) -> (5:w1499:string)  [unwired: 2 in, 2 out]
                  n868 = Fract/Exp String To Number(string=w1499) -> (number=w1501:dbl)  [unwired: 3 in, 1 out]
                  n869 = Build Array (concatenate)(w1506, w1501) -> (w1505:dbl[])
                }
              }
              n870 = property on="array for data" class="Arr (strict)"("Value"=w1496) -> ()  [unwired: 2 in, 2 out]
            }
            frame #20 {
              # "check if 2nd channel\non Keithley 2182 \n(addr. 16) is to\nbe measured"
              n871 = property on="Channel 2 (Vnano2b)" class="Bool (strict)"() -> ("Value"=w1507:bool)  [unwired: 2 in, 2 out]
              n872 = property on="array for data" class="Arr (strict)"() -> ("Value"=w1509:dbl[])  [unwired: 2 in, 2 out]
              n873 = case shown="False" w1507 {
                tunnel: w1509 -> [w1510 w1522]
                tunnel: [w1510 w1521] -> w1508
                frame False {
                  # "we are not measuring 1st channel\non Keithley 2182 (addr. 16)"
                }
                frame True {
                  w1513 = "16"
                  # "switching to channel 2 and then\nback to channel 1"
                  # "we are measuring 2nd channel\non Keithley 2182 (addr. 16)"
                  n874 = GPIB Write(0:w1513, 1:":SENSe:CHAN 2") -> (6:w1514:errorcluster)  [unwired: 3 in, 1 out]
                  n875 = GPIB Write(0:w1513, 1:":SENSe:DATA:FRES?", 3:w1514) -> (6:w1520:errorcluster)  [unwired: 2 in, 1 out]
                  n876 = GPIB Read(0:w1513, 1:200, 3:w1520) -> (5:w1516:string, 7:w1512:errorcluster)  [unwired: 2 in, 1 out]
                  n877 = GPIB Write(0:w1513, 1:":SENSe:CHAN 1", 3:w1512) -> ()  [unwired: 2 in, 2 out]
                  n878 = Fract/Exp String To Number(string=w1516) -> (number=w1518:dbl)  [unwired: 3 in, 1 out]
                  n879 = Build Array (concatenate)(w1522, w1518) -> (w1521:dbl[])
                }
              }
              n880 = property on="array for data" class="Arr (strict)"("Value"=w1508) -> ()  [unwired: 2 in, 2 out]
            }
            frame #21 {
              # "check if 1st channel\non Keithley 2182 \n(addr. 17) is to\nbe measured"
              n881 = property on="Channel 1 (Vnano3)" class="Bool (strict)"() -> ("Value"=w1523:bool)  [unwired: 2 in, 2 out]
              n882 = property on="array for data" class="Arr (strict)"() -> ("Value"=w1525:dbl[])  [unwired: 2 in, 2 out]
              n883 = case shown="False" w1523 {
                tunnel: w1525 -> [w1526 w1534]
                tunnel: [w1526 w1533] -> w1524
                frame False {
                  # "we are not measuring 1st channel\non Keithley 2182 (addr. 17)"
                }
                frame True {
                  w1531 = "17"
                  # "we are measuring 1st channel\non Keithley 2182 (addr. 17)"
                  n884 = GPIB Write(0:w1531, 1:":SENSe:DATA:FRES?") -> (6:w1532:errorcluster)  [unwired: 3 in, 1 out]
                  n885 = GPIB Read(0:w1531, 1:200, 3:w1532) -> (5:w1527:string)  [unwired: 2 in, 2 out]
                  n886 = Fract/Exp String To Number(string=w1527) -> (number=w1529:dbl)  [unwired: 3 in, 1 out]
                  n887 = Build Array (concatenate)(w1534, w1529) -> (w1533:dbl[])
                }
              }
              n888 = property on="array for data" class="Arr (strict)"("Value"=w1524) -> ()  [unwired: 2 in, 2 out]
            }
            frame #22 {
              # "check if 2nd channel\non Keithley 2182 \n(addr. 17) is to\nbe measured"
              n889 = property on="Channel 2 (Vnano3b)" class="Bool (strict)"() -> ("Value"=w1535:bool)  [unwired: 2 in, 2 out]
              n890 = property on="array for data" class="Arr (strict)"() -> ("Value"=w1537:dbl[])  [unwired: 2 in, 2 out]
              n891 = case shown="False" w1535 {
                tunnel: w1537 -> [w1538 w1550]
                tunnel: [w1538 w1549] -> w1536
                frame False {
                  # "we are not measuring 1st channel\non Keithley 2182 (addr. 17)"
                }
                frame True {
                  w1541 = "17"
                  # "switching to channel 2 and then\nback to channel 1"
                  # "we are measuring 2nd channel\non Keithley 2182 (addr. 17)"
                  n892 = GPIB Write(0:w1541, 1:":SENSe:CHAN 2") -> (6:w1542:errorcluster)  [unwired: 3 in, 1 out]
                  n893 = GPIB Write(0:w1541, 1:":SENSe:DATA:FRES?", 3:w1542) -> (6:w1548:errorcluster)  [unwired: 2 in, 1 out]
                  n894 = GPIB Read(0:w1541, 1:200, 3:w1548) -> (5:w1544:string, 7:w1540:errorcluster)  [unwired: 2 in, 1 out]
                  n895 = GPIB Write(0:w1541, 1:":SENSe:CHAN 1", 3:w1540) -> ()  [unwired: 2 in, 2 out]
                  n896 = Fract/Exp String To Number(string=w1544) -> (number=w1546:dbl)  [unwired: 3 in, 1 out]
                  n897 = Build Array (concatenate)(w1550, w1546) -> (w1549:dbl[])
                }
              }
              n898 = property on="array for data" class="Arr (strict)"("Value"=w1536) -> ()  [unwired: 2 in, 2 out]
            }
            frame #23 {
              # "check if 1st \nthermometer on \nOxford ITC \n(address 24) \nis measured"
              n899 = property on="Thermometer 1 (T1)" class="Bool (strict)"() -> ("Value"=w1551:bool)  [unwired: 2 in, 2 out]
              n900 = property on="array for data" class="Arr (strict)"() -> ("Value"=w1553:dbl[])  [unwired: 2 in, 2 out]
              n901 = case shown="True" w1551 {
                tunnel: w1553 -> [w1554 w1566]
                tunnel: [w1554 w1565] -> w1552
                frame False {
                  # "we are not measuring temperature on\nthermometer 1 (addr. 24)"
                }
                frame True {
                  (unwired) "\r"
                  w1559 = refnum<visa-resource-name> "TCPIP0::192.168.128.2::7020::SOCKET" ("VISA resource name")
                  # "we are measuring temperature,\nthermometer 1 (addr. 24)"
                  n902 = Concatenate Strings("READ:DEV:MB1.T1:TEMP:SIG:TEMP" ("string"), "\n") -> (w1558:string)
                  n903 = VISA Write(VISA resource name=w1559, write buffer=w1558) -> (error out=w1564:errorcluster)  [unwired: 1 in, 2 out]
                  n904 = String Length(string=w1558) -> (length=w1555:i32)
                  n905 = VISA Read(VISA resource name=w1559, byte count=1024, error in (no error)=w1564) -> (read buffer=w1562:string)  [unwired: 3 out]
                  n906 = String Subset(string=w1562, offset (0)=w1555) -> (substring=w1561:string)  [unwired: 1 in]
                  n907 = Fract/Exp String To Number(string=w1561) -> (number=w1557:dbl)  [unwired: 3 in, 1 out]
                  n908 = Build Array (concatenate)(w1566, w1557) -> (w1565:dbl[])
                }
              }
              n909 = property on="array for data" class="Arr (strict)"("Value"=w1552) -> ()  [unwired: 2 in, 2 out]
            }
            frame #24 {
              # "check if 1st \nthermometer on \nOxford ITC \n(address 24) \nis measured"
              n910 = property on="Magnetic Field (B)" class="Bool (strict)"() -> ("Value"=w1567:bool)  [unwired: 2 in, 2 out]
              n911 = property on="array for data" class="Arr (strict)"() -> ("Value"=w1569:dbl[])  [unwired: 2 in, 2 out]
              n912 = case shown="True" w1567 {
                tunnel: w1569 -> [w1570 w1582]
                tunnel: [w1570 w1581] -> w1568
                frame False {
                  # "we are not measuringmagnetic field (addr. 25)"
                }
                frame True {
                  (unwired) "\r"
                  w1575 = refnum<visa-resource-name> "TCPIP0::192.168.128.3::7020::SOCKET" ("VISA resource name")
                  # "we are measuring magnetic field  (addr. 25)"
                  n913 = Concatenate Strings("READ:DEV:GRPZ:PSU:SIG:PFLD" ("string"), "\n") -> (w1574:string)
                  n914 = VISA Write(VISA resource name=w1575, write buffer=w1574) -> (error out=w1580:errorcluster)  [unwired: 1 in, 2 out]
                  n915 = String Length(string=w1574) -> (length=w1571:i32)
                  n916 = VISA Read(VISA resource name=w1575, byte count=1024, error in (no error)=w1580) -> (read buffer=w1578:string)  [unwired: 3 out]
                  n917 = String Subset(string=w1578, offset (0)=w1571) -> (substring=w1577:string)  [unwired: 1 in]
                  n918 = Fract/Exp String To Number(string=w1577) -> (number=w1573:dbl)  [unwired: 3 in, 1 out]
                  n919 = Build Array (concatenate)(w1582, w1573) -> (w1581:dbl[])
                }
              }
              n920 = property on="array for data" class="Arr (strict)"("Value"=w1568) -> ()  [unwired: 2 in, 2 out]
            }
            frame #25 {
              # "check if capacitance\nand loss (address 28)\nare measured"
              n921 = property on="Capacitance (C) and Loss (L)" class="Bool (strict)"() -> ("Value"=w1583:bool)  [unwired: 2 in, 2 out]
              n922 = property on="array for data" class="Arr (strict)"() -> ("Value"=w1585:dbl[])  [unwired: 2 in, 2 out]
              n923 = case shown="True" w1583 {
                tunnel: w1585 -> [w1586 w1592]
                tunnel: [w1586 w1588] -> w1584
                frame False {
                  # "we are not measuringmagnetic capacitance (addr. 28)"
                }
                frame True {
                  # "we are measuring capacitance and loss  (addr. 28)"
                  n924 = stacked-sequence {
                    seq-local: [w1594 _ _] -> [_ _ w1617]
                    tunnel: [_ _ w1611] -> w1587
                    tunnel: [_ _ w1612] -> w1590
                    tunnel: "28" ("data") -> [w1593 w1597 w1606]
                    frame #0 {
                      n925 = GPIB Write(0:w1593, 1:"SINGLE" ("data"), 2:i16 0 ("mode (0)")) -> (6:w1594:errorcluster)  [unwired: 2 in, 1 out]
                    }
                    frame #1 {
                      n926 = while {
                        tunnel: w1597 -> [w1598]
                        i -> [w1599]
                        stop <- w1601 continue-if-true
                        n927 = GPIB Serial Poll(0:w1598) -> (2:w1603:i16)  [unwired: 1 in, 2 out]
                        n928 = Less?(x=w1603, y=i16 128) -> (x < y?=w1601:bool)
                        n929 = Wait (ms)(milliseconds to wait=u32 50) -> ()  [unwired: 1 out]
                        "Numeric 3" <- w1599
                      }
                    }
                    frame #2 {
                      w1604 = i16 2 ("mode (0)")
                      n930 = GPIB Read(0:w1606, 1:200 ("byte count"), 2:i16 2 ("mode (0)"), 3:w1617) -> (5:w1610:string)  [unwired: 1 in, 2 out]
                      n931 = Match Pattern(string=w1610, regular expression="C=") -> (after substring=w1609:string)  [unwired: 1 in, 3 out]
                      n932 = Match Pattern(string=w1609, regular expression="PF L=") -> (after substring=w1607:string)  [unwired: 1 in, 3 out]
                      n933 = Search/Split String(string=w1609, search string/char (-)=" ", offset (0)=w1604) -> (substring before match=w1614:string)  [unwired: 2 out]
                      n934 = Search/Split String(string=w1607, search string/char (-)=" ", offset (0)=w1604) -> (substring before match=w1613:string)  [unwired: 2 out]
                      n935 = Fract/Exp String To Number(string=w1613) -> (number=w1611:dbl)  [unwired: 3 in, 1 out]
                      n936 = Fract/Exp String To Number(string=w1614) -> (number=w1612:dbl)  [unwired: 3 in, 1 out]
                    }
                  }
                  n937 = Build Array (concatenate)(w1592, w1590) -> (w1589:dbl[])
                  n938 = Build Array (concatenate)(w1589, w1587) -> (w1588:dbl[])
                }
              }
              n939 = property on="array for data" class="Arr (strict)"("Value"=w1584) -> ()  [unwired: 2 in, 2 out]
            }
          }
        }
      }
      n940 = property on="array for data" class="Arr (strict)"(error in=w448) -> ("Value"=w426:dbl[])  [unwired: 1 in, 2 out]
      n941 = while {
        shift-right: [w1631] -> w422
        shift-left: w426 -> [w1633]
        i -> [w1632]
        stop <- w1636 stop-if-true
        # "loop goes through the list of all measured parameters\nif some columns are identified as current or resistance\nthey are recalculated according to selected or entered parameters"
        n942 = Increment(x=w1632) -> (x+1=w1637:i32)
        n943 = property on="Ring" class="Ring (strict)"() -> ("Strings []"=w1635:string[])  [unwired: 2 in, 2 out]
        n944 = Index Array(array=w1635, index=w1632) -> (element=w1634:string)
        n945 = property on="Ring" class="Ring (strict)"() -> ("NumItems"=w1638:u32)  [unwired: 2 in, 2 out]
        n946 = case shown="\"R1\", \"R1oop\", \"R2\", \"R2oop\", \"R3\", \"R3oop\", \"R4\", \"R4oop\", \"R5\", \"R5oop\"" w1634 {
          tunnel: w1633 -> [w1644 w1654 w1664 w1671]
          tunnel: w1632 -> [w1642 w1651 w1662 _]
          tunnel: [w1643 w1652 w1663 w1671] -> w1631
          frame "I" {
            n947 = property on="Current is:" class="RadioBtnsControl (strict)"() -> ("Value"=w1640:T1)  [unwired: 2 in, 2 out]
            n948 = case shown="\"Radio Selection 2\"" w1640 {
              tunnel: ["Ring 3" "Ring 2"] -> w1639
              frame "Radio Selection 3", Default {
              }
              frame "Radio Selection 2" {
              }
            }
            n949 = Index Array(array=w1644, index=w1642) -> (element=w1645:dbl)
            n950 = Power Of 10(x=w1639) -> (10^x=w1648:dbl)
            n951 = Multiply(x=1000.0, y=w1648) -> (x*y=w1646:dbl)
            n952 = Divide(x=w1645, y=w1646) -> (x/y=w1641:dbl)
            "Numeric Current" <- w1641
            n953 = Replace Array Subset(array=w1644, new element=w1641, index=w1642) -> (w1643:dbl[])
          }
          frame "Ioop" {
            n954 = property on="Ring 3" class="Ring (strict)"() -> ("Value"=w1653:u16)  [unwired: 2 in, 2 out]
            n955 = Index Array(array=w1654, index=w1651) -> (element=w1656:dbl)
            n956 = Power Of 10(x=w1653) -> (10^x=w1659:dbl)
            n957 = Multiply(x=1000.0, y=w1659) -> (x*y=w1657:dbl)
            n958 = Divide(x=w1656, y=w1657) -> (x/y=w1655:dbl)
            n959 = Replace Array Subset(array=w1654, new element=w1655, index=w1651) -> (w1652:dbl[])
          }
          frame "R1", "R1oop", "R2", "R2oop", "R3", "R3oop", "R4", "R4oop", "R5", "R5oop" {
            n960 = property on="Current is:" class="RadioBtnsControl (strict)"() -> ("Value"=w1661:T1)  [unwired: 2 in, 2 out]
            n961 = case shown="\"Radio Selection 1\"" w1661 {
              tunnel: [w1667 w1670] -> w1660
              frame "Radio Selection 1" {
                n962 = Divide(x="Fixed Current mkA", y=1000000.0) -> (x/y=w1667:dbl)
              }
              frame "Radio Selection 2", Default {
                n963 = property on="Numeric Current" class="DigNum (strict)"() -> ("Value"=w1670:dbl)  [unwired: 2 in, 2 out]
              }
            }
            n964 = Index Array(array=w1664, index=w1662) -> (element=w1666:dbl)
            n965 = Divide(x=w1666, y=w1660) -> (x/y=w1665:dbl)
            n966 = Replace Array Subset(array=w1664, new element=w1665, index=w1662) -> (w1663:dbl[])
          }
          frame "False", Default {
          }
        }
        n967 = Less?(x=w1638, y=w1637) -> (x < y?=w1636:bool)
      }
      n968 = Subtract(x="Target Voltage, V", y=w432) -> (x-y=w435:dbl)
      n969 = Divide(x="Sweep rate, V/min", y=60.0) -> (x/y=w444:dbl)
      n970 = Multiply(x=w444, y="Time btw \npoints, sec") -> (x*y=w427:dbl)
      n971 = Sign(1:w435) -> (0:w428:dbl)
      n972 = Multiply(x=w428, y=w427) -> (x*y=w420:dbl)
      n973 = property on="points at each Vg" class="DigNum (strict)"() -> ("Value"=w419:i32)  [unwired: 2 in, 2 out]
      n974 = To Double Precision Float(number=w419) -> (double precision float=w418:dbl)
      n975 = Multiply(x=w418, y=w420) -> (x*y=w417:dbl)
      n976 = property on="Commutator" class="Bool (strict)"() -> ("Value"=w411:bool)  [unwired: 2 in, 2 out]
      n977 = property on="Data file:" class="Path"() -> ("Value"=w424:path)  [unwired: 2 in, 2 out]
      n978 = Divide(x=w435, y=w417) -> (x/y=w442:dbl)
      n979 = case shown="False" w411 {
        tunnel: w429 -> [w462 w473]
        tunnel: w413 -> [w457 w467]
        tunnel: [w449 w466] -> w410
        frame True {
          # "calculate deliberate time delay for the next step"
          n980 = Subtract(x=w462, y=w457) -> (x-y=w455:u32)
          n981 = property on="Delib Time delay" class="DigNum (strict)"() -> ("Value"=w456:i32)  [unwired: 2 in, 2 out]
          n982 = property on="Time btw \npoints, sec" class="DigNum (strict)"() -> ("Value"=w461:dbl)  [unwired: 2 in, 2 out]
          n983 = Subtract(x=w455, y=w456) -> (x-y=w454:u32)
          n984 = Multiply(x=w461, y=1000.0) -> (x*y=w459:dbl)
          n985 = To Long Integer(number=w459) -> (32bit integer=w458:i32)
          n986 = Greater?(x=w458, y=w454) -> (0:w451:bool)
          n987 = Subtract(x=w458, y=w454) -> (x-y=w453:u32)
          n988 = Divide(x=w453, y=2) -> (x/y=w450:dbl)
          n989 = case shown="False" w451 {
            tunnel: w450 -> [_ w465]
            tunnel: [0 w464] -> w449
            frame False {
            }
            frame True {
              n990 = To Long Integer(number=w465) -> (32bit integer=w464:i32)
            }
          }
        }
        frame False {
          # "calculate deliberate time delay for the next step"
          n991 = Subtract(x=w473, y=w467) -> (x-y=w470:u32)
          n992 = property on="Time btw \npoints, sec" class="DigNum (strict)"() -> ("Value"=w472:dbl)  [unwired: 2 in, 2 out]
          n993 = Multiply(x=w472, y=1000.0) -> (x*y=w469:dbl)
          n994 = To Long Integer(number=w469) -> (32bit integer=w468:i32)
          n995 = Greater?(x=w468, y=w470) -> ()  [unwired: 1 out]
          n996 = Subtract(x=w468, y=w470) -> (x-y=w466:u32)
        }
      }
      "Delib Time delay" <- w410
      n997 = Decrement(x=w442) -> (x-1=w441:dbl)
      n998 = Absolute Value(x=w435) -> (abs(x)=w437:dbl)
      n999 = Build Array (concatenate)(w447, w422) -> (w421:dbl[][])
      n1000 = Greater Than 0?(x=w441) -> (x > 0?=w440:bool)
      n1001 = property on="array for data" class="Arr (strict)"("Value"=w422) -> ()  [unwired: 2 in, 2 out]
      n1002 = call-poly <vilib>:"Write To Spreadsheet File.vi"("format (%.3f)"="%#g", "append to file? (new file:F)"=TRUE, "1D data"=w422, "file path (dialog if empty)"=w424) -> ()  [unwired: 4 in, 1 out]
      n1003 = Less?(x=w437, y=1e-06) -> (x < y?=w434:bool)
      n1004 = flat-sequence {
        tunnel: [w1630] -> w429
        tunnel: w421 -> [w1624]
        frame #0 {
          # "time is mesured at the end of the cycle\nto adjust a delay time"
          # "this part plots selected measurements"
          n1005 = Tick Count (ms)() -> (millisecond timer value=w1630:u32)
          n1006 = Index Array(array=w1624, index (col)="Ring") -> (element=w1629:dbl[])  [unwired: 1 in]
          n1007 = Index Array(array=w1624, index (col)=0) -> (element=w1627:dbl[])  [unwired: 1 in]
          n1008 = Bundle(w1627, w1629) -> (→"XY Graph":cluster{dbl[], dbl[]})  [unwired: 1 in]
        }
      }
      n1009 = case shown="True" w440 {
        tunnel: w432 -> [_ w1675]
        tunnel: w417 -> [_ w1674]
        tunnel: [w1672 w1673] -> w439
        frame False {
          # "if next step is too long\nuse target voltage"
          n1010 = property on="Target Voltage, V" class="DigNum (strict)"() -> ("Value"=w1672:dbl)  [unwired: 2 in, 2 out]
        }
        frame True {
          # "add increment to\nthe current Vg"
          n1011 = Add(x=w1674, y=w1675) -> (x+y=w1673:dbl)
        }
      }
    }
    n1012 = Number To Fractional String(number=w389) -> (F-format string=w394:string)  [unwired: 3 in]
    n1013 = property on="Main Keithly2614B address" class="Str"() -> ("Value"=w392:string)  [unwired: 2 in, 2 out]
    n1014 = Concatenate Strings("smua.source.levelv = " ("data"), w394) -> (w393:string)
    n1015 = Equal?(x=w387, y="optional Bias (V)") -> (x = y?=w390:bool)
    n1016 = case shown="True" w390 {
      tunnel: "optional Bias (V)" -> [w401 _]
      tunnel: w389 -> [w402 _]
      frame False {
        n1017 = Multiply(x=w402, y=22.62) -> (x*y=w403:dbl)
        n1018 = Number To Fractional String(number=w401) -> (F-format string=w409:string)  [unwired: 3 in]
        n1019 = Add(x=w401, y=w403) -> ()  [unwired: 1 out]
        n1020 = Concatenate Strings(":INIT:IMM; :SOUR:VOLT:LEV:IMM:AMPL " ("data"), w409) -> (w408:string)
        n1021 = property on="optional Bias (V)" class="DigNum (strict)"("Visible"=TRUE) -> ()  [unwired: 2 in, 2 out]
        n1022 = GPIB Write(0:"13", 1:w408) -> ()  [unwired: 3 in, 2 out]
      }
      frame True {
      }
    }
    n1023 = GPIB Write(0:w392, 1:w393) -> ()  [unwired: 3 in, 2 out]
  }
  "Array 2" <- w17
  n1024 = Concatenate Strings(w7, w3, w4, w3, w4, w2, w3, w4) -> (w19:string)
  "String" <- w19
  n1025 = Write to Text File(file (use dialog)=w20, text=w19) -> ()  [unwired: 2 in, 3 out]
  n1026 = property on="optional Bias (V)" class="DigNum (strict)"("Value"=w15, "Visible"=FALSE) -> ()  [unwired: 2 in, 2 out]
